vi "Beampointing_Multi_TRA2.vi"() -> ()   [LabVIEW 2020]
uses:
  Shared/GUI_Template/GUI_master/tcp new data cluster.ctl
  <userlib>/_OpenG.lib/array/array.llb/Filter 1D Array with Scalar (String)__ogtk.vi
  <vilib>/Utility/file.llb/Write To Spreadsheet File (string).vi
  <vilib>/Utility/file.llb/Read From Spreadsheet File (string).vi
  <vilib>/Analysis/NI_AALBase.lvlib
  GUI_Beampointing_single_TRA/Ctrs/move.ctl
  Ctrs/beam detection.ctl
  Shared/GUI_Template/GUI_master/tcp_new_data_event.ctl
panel:
  out "size(s) 6":i32
  out "x-y*floor(x/y)":dbl
  out "config path":string
  out "motor refs 7":refnum<vi>[](array[refnum])
  out "Moving Y":string
  out "Moving X":string
  out "particles":T1(array[cluster])
  out "motor refs 6":refnum<vi>[](array[refnum])
  out "millisecond timer value":u32
  out "motor refs 5":refnum<vi>[](array[refnum])
  out "appended path":path
  out "motor refs 4":refnum<vi>[](array[refnum])
  in  "active Axis ref 3":cluster{"Ref X":refnum<vi>, "Ref Y":refnum<vi>}
  out "motor refs 3":refnum<vi>[](array[refnum])
  in  "active man refs":cluster{"Ref X":refnum<vi>, "Ref Y":refnum<vi>}
  out "motor refs 2":refnum<vi>[](array[refnum])
  in  "Numeric":dbl
  out "Current State":string
  in  "output cluster 2":T5 {"detection para"."smal para"."Measurement Parameter" items=["Center of Mass X", "Center of Mass Y", "First Pixel X", "First Pixel Y", "Bounding Rect Left", "Bounding Rect Top", "Bounding Rect Right", "Bounding Rect Bottom", "Max Feret Diameter Start X", "Max Feret Diameter Start Y", "Max Feret Diameter End X", "Max Feret Diameter End Y", "Max Horiz. Segment Length Left", "Max Horiz. Segment Length Right", "Max Horiz. Segment Length Row", "-", "Bounding Rect Width", "Bounding Rect Height", "Bounding Rect Diagonal", "Perimeter", "Convex Hull Perimeter", "Holes' Perimeter", "Max Feret Diameter", "Equivalent Ellipse Major Axis", "Equivalent Ellipse Minor Axis", "Equivalent Ellipse Minor Axis (Feret)", "Equivalent Rect Long Side", "Equivalent Rect Short Side", "Equivalent Rect Diagonal", "Equivalent Rect Short Side (Feret)", "Average Horiz. Segment Length", "Average Vert. Segment Length", "Hydraulic Radius", "Waddel Disk Diameter", "-", "Area", "Holes' Area", "Particle & Holes' Area", "Convex Hull Area", "Image Area", "-", "Number of Holes", "Number of Horiz. Segments", "Number of Vert. Segments", "-", "Orientation", "Max Feret Diameter Orientation", "-", "% Area/Image Area", "% Area/(Particle & Holes' Area)", "Ratio of Equivalent Ellipse Axes", "Ratio of Equivalent Rect Sides", "-", "Elongation Factor", "Compactness Factor", "Heywood Circularity Factor", "Type Factor", "-", "Sum X", "Sum Y", "Sum XX", "Sum XY", "Sum YY", "Sum XXX", "Sum XXY", "Sum XYY", "Sum YYY", "-", "Moment of Inertia XX", "Moment of Inertia XY", "Moment of Inertia YY", "Moment of Inertia XXX", "Moment of Inertia XXY", "Moment of Inertia XYY", "Moment of Inertia YYY", "Norm. Moment of Inertia XX", "Norm. Moment of Inertia XY", "Norm. Moment of Inertia YY", "Norm. Moment of Inertia XXX", "Norm. Moment of Inertia XXY", "Norm. Moment of Inertia XYY", "Norm. Moment of Inertia YYY", "Hu Moment 1", "Hu Moment 2", "Hu Moment 3", "Hu Moment 4", "Hu Moment 5", "Hu Moment 6", "Hu Moment 7"]; "detection para"."smal para"."Range Lower Value" format="%.2f"; "detection para"."smal para"."Range Upper Value" format="%.2f"; "detection para"."detection method" items=["clustering", "entropy", "metric", "moments", "inter-class variance"]; "detection para"."Filter" items=["No Filter", "Median Filter", "Low Pass Filter"]}
  out "CCDs":string[](array[string])
  in  "GUIdevice 12":string
  in  "GUIdevice 11":string
  in  "GUIdevice 10":string
  in  "GUIdevice 9":string
  out "error out 2":errorcluster
  in  "active cams":string[](array[string])
  in  "Motor Y":dbl[][](array[numeric])
  in  "Motor X":dbl[][](array[numeric])
  out "Names":string[](array[string])
  in  "Offset X stats":dbl[][](array[numeric])
  in  "Offset Y stats":dbl[][](array[numeric])
  out "Box":T6(array[cluster])
  in  "Tab Control 2":enum32{"Config ", "Main", "History"}(tab)=enum."Main"
  in  "associated motors":T7 {"Motor CCD 12" items=["M20", "SIM", "M22", ""]; "Motor CCD 11" items=["M20", "SIM", "M22", ""]; "Motor CCD 10" items=["M20", "SIM", "M22", ""]; "Motor CCD 9" items=["M20", "SIM", "M22", ""]; "Motor CCD 8" items=["M20", "SIM", "M22", ""]; "Motor CCD 7" items=["M20", "SIM", "M22", ""]; "Motor CCD 6" items=["M20", "SIM", "M22", ""]; "Motor CCD 5" items=["M20", "SIM", "M22", ""]; "Motor CCD 4" items=["M20", "SIM", "M22", ""]; "Motor CCD 3" items=["M20", "SIM", "M22", ""]; "Motor CCD 2" items=["M20", "SIM", "M22", ""]; "Motor CCD 1" items=["M20", "SIM", "M22", ""]}
  out "Cameras":T8
  out "Status":cluster{i32, i32, "Centroid X":dbl[][]}(graph)
  in  "Exposure:12":dbl=0.095 min=0.0001 max=1.0 format="%#_6f"
  in  "Triggerdelay::12":dbl=0.003 min=0.0 max=0.09 format="%#_6f"
  in  "Exposure::11":dbl=0.095 min=0.0001 max=1.0 format="%#_6f"
  in  "Triggerdelay::11":dbl=0.003 min=0.0 max=0.09 format="%#_6f"
  in  "Exposure::10":dbl=0.095 min=0.0001 max=1.0 format="%#_6f"
  in  "Triggerdelay::10":dbl=0.003 min=0.0 max=0.09 format="%#_6f"
  in  "Exposure::9":dbl=0.095 min=0.0001 max=1.0 format="%#_6f"
  in  "Triggerdelay::9":dbl=0.003 min=0.0 max=0.09 format="%#_6f"
  in  "Trigger::9":bool
  in  "Trigger::10":bool caption="Trigger:10"
  in  "Trigger::11":bool
  in  "Trigger::12":bool
  in  "Target.Y::9":dbl=45.0 caption="T9y" min=0.0 max=2000.0 format="%#_6f"
  in  "Target.X::9":dbl=47.0 caption="Tx9" min=0.0 max=2000.0 format="%#_6f"
  in  "Target.Y::10":dbl=45.0 caption="T10y" min=0.0 max=2000.0 format="%#_6f"
  in  "Target.X::10":dbl=47.0 caption="T10x" min=0.0 max=2000.0 format="%#_6f"
  in  "Target.Y::11":dbl=45.0 caption="T11y" min=0.0 max=2000.0 format="%#_6f"
  in  "Target.X::11":dbl=47.0 caption="T11x" min=0.0 max=2000.0 format="%#_6f"
  in  "Target.Y::12":dbl=45.0 caption="T12y" min=0.0 max=2000.0 format="%#_6f"
  in  "Target.X::12":dbl=47.0 caption="T12x" min=0.0 max=2000.0 format="%#_6f"
  in  "Exposure::8":dbl=0.095 min=0.0001 max=1.0 format="%#_6f"
  in  "Triggerdelay::8":dbl=0.003 min=0.0 max=0.09 format="%#_6f"
  in  "Trigger::8":bool
  in  "Target.Y::8":dbl=45.0 caption="T8y" min=0.0 max=2000.0 format="%#_6f"
  in  "Target.X::8":dbl=47.0 caption="T8x" min=0.0 max=2000.0 format="%#_6f"
  in  "Target.Y::7":dbl=45.0 caption="T7x" min=0.0 max=2000.0 format="%#_6f"
  in  "Target.X::7":dbl=47.0 caption="T7y" min=0.0 max=2000.0 format="%#_6f"
  in  "Target.Y::6":dbl=45.0 caption="T6y" min=0.0 max=2000.0 format="%#_6f"
  in  "Target.X::6":dbl=47.0 caption="T6x" min=0.0 max=2000.0 format="%#_6f"
  in  "Target.Y::5":dbl=45.0 caption="T5y" min=0.0 max=2000.0 format="%#_6f"
  in  "Target.X::5":dbl=47.0 caption="T5x" min=0.0 max=2000.0 format="%#_6f"
  in  "Target.Y::4":dbl=45.0 caption="T4y" min=0.0 max=2000.0 format="%#_6f"
  in  "Target.X::4":dbl=47.0 caption="T4x" min=0.0 max=2000.0 format="%#_6f"
  in  "Target.Y::3":dbl=163.0 caption="T3y" min=0.0 max=2000.0 format="%#_6f"
  in  "Target.X::3":dbl=152.0 caption="T3x" min=0.0 max=2000.0 format="%#_6f"
  in  "Target.Y::2":dbl=74.0 caption="T2y" min=0.0 max=2000.0 format="%#_6f"
  in  "Target.X::2":dbl=75.0 caption="T2x" min=0.0 max=2000.0 format="%#_6f"
  in  "Target.Y::1":dbl=61.0 caption="T1y" min=0.0 max=2000.0 format="%#_6f"
  in  "Target.X::1":dbl=77.0 caption="T1x" min=0.0 max=2000.0 format="%#_6f"
  in  "Exposure::7":dbl=0.095 min=0.0001 max=1.0 format="%#_6f"
  in  "Triggerdelay::7":dbl=0.003 min=0.0 max=0.09 format="%#_6f"
  in  "Trigger::7":bool
  in  "Exposure::6":dbl=0.095 min=0.0001 max=1.0 format="%#_6f"
  in  "Triggerdelay::6":dbl=0.003 min=0.0 max=0.09 format="%#_6f"
  in  "Trigger::6":bool
  in  "Exposure::5":dbl=0.095 min=0.0001 max=1.0 format="%#_6f"
  in  "Triggerdelay::5":dbl=0.003 min=0.0 max=0.09 format="%#_6f"
  in  "Trigger::5":bool
  in  "Exposure::4":dbl=0.095 min=0.0001 max=1.0 format="%#_6f"
  in  "Triggerdelay::4":dbl=0.003 min=0.0 max=0.09 format="%#_6f"
  in  "Trigger::4":bool
  in  "Exposure::3":dbl=0.095 min=0.0001 max=1.0 format="%#_6f"
  in  "Triggerdelay::3":dbl=0.003 min=0.0 max=0.09 format="%#_6f"
  in  "Trigger::3":bool
  in  "Exposure::2":dbl=0.095 min=0.0001 max=1.0 format="%#_6f"
  in  "Triggerdelay::2":dbl=0.003 min=0.0 max=0.09 format="%#_6f"
  in  "Trigger::2":bool
  out "image::1":T9(plugin-control) caption="B3_TelLens2"
  out "image::2":T9(plugin-control) caption="B6_SwitchYNear"
  out "image::3":T9(plugin-control) caption="StagingM1Near"
  out "image::4":T9(plugin-control) caption="StagingM1Far"
  out "image::5":T9(plugin-control)
  out "image::6":T9(plugin-control)
  out "image::7":T9(plugin-control)
  out "image::8":T9(plugin-control)
  in  "Exposure::1":dbl=0.095 min=0.0001 max=1.0 format="%#_6f"
  in  "Triggerdelay::1":dbl=0.003 min=0.0 max=0.09 format="%#_6f"
  in  "Trigger::1":bool
  in  "UDP error message":string
  out "required Y":bool[](array[boolean])
  out "required X":bool[](array[boolean])
  out "detected":bool[](array[boolean])
  out "name array":string[](array[string])
  out "image::9":T9(plugin-control)
  out "image::10":T9(plugin-control)
  out "image::11":T9(plugin-control)
  out "image::12":T9(plugin-control)
  out "speedmode X":bool[](array[boolean])
  out "speedmode Y":bool[](array[boolean])
  out "CCD 9":cluster{timestamp[], dbl[]}[](graph)
  out "CCD 10":cluster{timestamp[], dbl[]}[](graph)
  out "CCD 11":cluster{timestamp[], dbl[]}[](graph)
  out "CCD 12":cluster{timestamp[], dbl[]}[](graph)
  out "CCD 5":cluster{timestamp[], dbl[]}[](graph)
  out "CCD 6":cluster{timestamp[], dbl[]}[](graph)
  out "CCD 7":cluster{timestamp[], dbl[]}[](graph)
  out "CCD 8":cluster{timestamp[], dbl[]}[](graph)
  out "CCD 2":cluster{timestamp[], dbl[]}[](graph)
  out "CCD 1":cluster{timestamp[], dbl[]}[](graph)
  out "CCD 3":cluster{timestamp[], dbl[]}[](graph)
  out "CCD 4":cluster{timestamp[], dbl[]}[](graph)
  in  "History Size":i32=500
  out "History Index":i32
  in  "Feedback Global":bool
  in  "detection para":T3[](array[typedef])=[{"Filter"=1, "Filter Para"={"X Size"=5, "Y Size"=5, "% Tolerance"=1}, "detection method"=4, "smal para"=[{"Measurement Parameter"=35, "Range Lower Value"=0.0, "Range Upper Value"=0.0, "Range"=TRUE, "Measurement Type"=FALSE}], "Remove small Objects"=TRUE, "Restrict to round Objects"=FALSE}, {"Filter"=1, "Filter Para"={"X Size"=5, "Y Size"=5, "% Tolerance"=1}, "detection method"=4, "smal para"=[{"Measurement Parameter"=35, "Range Lower Value"=0.0, "Range Upper Value"=500.0, "Range"=FALSE, "Measurement Type"=FALSE}], "Remove small Objects"=TRUE, "Restrict to round Objects"=FALSE}, {"Filter"=1, "Filter Para"={"X Size"=5, "Y Size"=5, "% Tolerance"=1}, "detection method"=4, "smal para"=[{"Measurement Parameter"=35, "Range Lower Value"=0.0, "Range Upper Value"=500.0, "Range"=TRUE, "Measurement Type"=FALSE}], "Remove small Objects"=TRUE, "Restrict to round Objects"=FALSE}, {"Filter"=1, "Filter Para"={"X Size"=5, "Y Size"=5, "% Tolerance"=1}, "detection method"=4, "smal para"=[{"Measurement Parameter"=35, "Range Lower Value"=0.0, "Range Upper Value"=500.0, "Range"=TRUE, "Measurement Type"=FALSE}], "Remove small Objects"=TRUE, "Restrict to round Objects"=FALSE}, {"Filter"=1, "Filter Para"={"X Size"=5, "Y Size"=5, "% Tolerance"=1}, "detection method"=4, "smal para"=[{"Measurement Parameter"=35, "Range Lower Value"=0.0, "Range Upper Value"=500.0, "Range"=TRUE, "Measurement Type"=FALSE}], "Remove small Objects"=TRUE, "Restrict to round Objects"=FALSE}, {"Filter"=1, "Filter Para"={"X Size"=5, "Y Size"=5, "% Tolerance"=1}, "detection method"=4, "smal para"=[{"Measurement Parameter"=35, "Range Lower Value"=0.0, "Range Upper Value"=500.0, "Range"=TRUE, "Measurement Type"=FALSE}], "Remove small Objects"=TRUE, "Restrict to round Objects"=FALSE}, {"Filter"=1, "Filter Para"={"X Size"=5, "Y Size"=5, "% Tolerance"=1}, "detection method"=4, "smal para"=[{"Measurement Parameter"=35, "Range Lower Value"=0.0, "Range Upper Value"=500.0, "Range"=TRUE, "Measurement Type"=FALSE}], "Remove small Objects"=TRUE, "Restrict to round Objects"=FALSE}, {"Filter"=1, "Filter Para"={"X Size"=5, "Y Size"=5, "% Tolerance"=1}, "detection method"=3, "smal para"=[{"Measurement Parameter"=35, "Range Lower Value"=0.0, "Range Upper Value"=0.0, "Range"=FALSE, "Measurement Type"=FALSE}], "Remove small Objects"=TRUE, "Restrict to round Objects"=FALSE}, {"Filter"=1, "Filter Para"={"X Size"=5, "Y Size"=5, "% Tolerance"=1}, "detection method"=4, "smal para"=[{"Measurement Parameter"=35, "Range Lower Value"=0.0, "Range Upper Value"=0.0, "Range"=FALSE, "Measurement Type"=FALSE}], "Remove small Objects"=TRUE, "Restrict to round Objects"=FALSE}, {"Filter"=1, "Filter Para"={"X Size"=5, "Y Size"=5, "% Tolerance"=1}, "detection method"=4, "smal para"=[{"Measurement Parameter"=35, "Range Lower Value"=0.0, "Range Upper Value"=500.0, "Range"=TRUE, "Measurement Type"=FALSE}], "Remove small Objects"=TRUE, "Restrict to round Objects"=FALSE}, {"Filter"=1, "Filter Para"={"X Size"=5, "Y Size"=5, "% Tolerance"=1}, "detection method"=4, "smal para"=[{"Measurement Parameter"=35, "Range Lower Value"=0.0, "Range Upper Value"=500.0, "Range"=TRUE, "Measurement Type"=FALSE}], "Remove small Objects"=TRUE, "Restrict to round Objects"=FALSE}, {"Filter"=1, "Filter Para"={"X Size"=5, "Y Size"=5, "% Tolerance"=1}, "detection method"=4, "smal para"=[{"Measurement Parameter"=35, "Range Lower Value"=0.0, "Range Upper Value"=500.0, "Range"=TRUE, "Measurement Type"=FALSE}], "Remove small Objects"=TRUE, "Restrict to round Objects"=FALSE}] {"smal para"."Measurement Parameter" items=["Center of Mass X", "Center of Mass Y", "First Pixel X", "First Pixel Y", "Bounding Rect Left", "Bounding Rect Top", "Bounding Rect Right", "Bounding Rect Bottom", "Max Feret Diameter Start X", "Max Feret Diameter Start Y", "Max Feret Diameter End X", "Max Feret Diameter End Y", "Max Horiz. Segment Length Left", "Max Horiz. Segment Length Right", "Max Horiz. Segment Length Row", "-", "Bounding Rect Width", "Bounding Rect Height", "Bounding Rect Diagonal", "Perimeter", "Convex Hull Perimeter", "Holes' Perimeter", "Max Feret Diameter", "Equivalent Ellipse Major Axis", "Equivalent Ellipse Minor Axis", "Equivalent Ellipse Minor Axis (Feret)", "Equivalent Rect Long Side", "Equivalent Rect Short Side", "Equivalent Rect Diagonal", "Equivalent Rect Short Side (Feret)", "Average Horiz. Segment Length", "Average Vert. Segment Length", "Hydraulic Radius", "Waddel Disk Diameter", "-", "Area", "Holes' Area", "Particle & Holes' Area", "Convex Hull Area", "Image Area", "-", "Number of Holes", "Number of Horiz. Segments", "Number of Vert. Segments", "-", "Orientation", "Max Feret Diameter Orientation", "-", "% Area/Image Area", "% Area/(Particle & Holes' Area)", "Ratio of Equivalent Ellipse Axes", "Ratio of Equivalent Rect Sides", "-", "Elongation Factor", "Compactness Factor", "Heywood Circularity Factor", "Type Factor", "-", "Sum X", "Sum Y", "Sum XX", "Sum XY", "Sum YY", "Sum XXX", "Sum XXY", "Sum XYY", "Sum YYY", "-", "Moment of Inertia XX", "Moment of Inertia XY", "Moment of Inertia YY", "Moment of Inertia XXX", "Moment of Inertia XXY", "Moment of Inertia XYY", "Moment of Inertia YYY", "Norm. Moment of Inertia XX", "Norm. Moment of Inertia XY", "Norm. Moment of Inertia YY", "Norm. Moment of Inertia XXX", "Norm. Moment of Inertia XXY", "Norm. Moment of Inertia XYY", "Norm. Moment of Inertia YYY", "Hu Moment 1", "Hu Moment 2", "Hu Moment 3", "Hu Moment 4", "Hu Moment 5", "Hu Moment 6", "Hu Moment 7"]; "smal para"."Range Lower Value" format="%.2f"; "smal para"."Range Upper Value" format="%.2f"; "detection method" items=["clustering", "entropy", "metric", "moments", "inter-class variance"]; "Filter" items=["No Filter", "Median Filter", "Low Pass Filter"]}
  in  "GUIdevice 8":string
  in  "Tab Control":T10(tab)=enum."Detection"
  in  "new tdms":bool
  in  "Save Stats":bool
  in  "Save Config":bool
  in  "Load Config":bool
  in  "update speed [ms]":i32=200
  in  "img to avg":i32=6 min=3 max=200
  in  "Reset History":bool
  in  "save path":path=path "W:/BP_DATA"
  in  "autodetect":bool
  in  "Detection Rate":dbl=0.9 min=0.001 max=1.0
  in  "Center":bool
  in  "Align":bool
  in  "Speedmode @":dbl=3.0 min=1.0 max=20.0
  in  "device ini":bool
  in  "beam detection para":T3={"Filter"=1, "Filter Para"={"X Size"=5, "Y Size"=5, "% Tolerance"=1}, "detection method"=4, "smal para"=[{"Measurement Parameter"=35, "Range Lower Value"=0.0, "Range Upper Value"=500.0, "Range"=FALSE, "Measurement Type"=FALSE}], "Remove small Objects"=TRUE, "Restrict to round Objects"=FALSE} {"smal para"."Measurement Parameter" items=["Center of Mass X", "Center of Mass Y", "First Pixel X", "First Pixel Y", "Bounding Rect Left", "Bounding Rect Top", "Bounding Rect Right", "Bounding Rect Bottom", "Max Feret Diameter Start X", "Max Feret Diameter Start Y", "Max Feret Diameter End X", "Max Feret Diameter End Y", "Max Horiz. Segment Length Left", "Max Horiz. Segment Length Right", "Max Horiz. Segment Length Row", "-", "Bounding Rect Width", "Bounding Rect Height", "Bounding Rect Diagonal", "Perimeter", "Convex Hull Perimeter", "Holes' Perimeter", "Max Feret Diameter", "Equivalent Ellipse Major Axis", "Equivalent Ellipse Minor Axis", "Equivalent Ellipse Minor Axis (Feret)", "Equivalent Rect Long Side", "Equivalent Rect Short Side", "Equivalent Rect Diagonal", "Equivalent Rect Short Side (Feret)", "Average Horiz. Segment Length", "Average Vert. Segment Length", "Hydraulic Radius", "Waddel Disk Diameter", "-", "Area", "Holes' Area", "Particle & Holes' Area", "Convex Hull Area", "Image Area", "-", "Number of Holes", "Number of Horiz. Segments", "Number of Vert. Segments", "-", "Orientation", "Max Feret Diameter Orientation", "-", "% Area/Image Area", "% Area/(Particle & Holes' Area)", "Ratio of Equivalent Ellipse Axes", "Ratio of Equivalent Rect Sides", "-", "Elongation Factor", "Compactness Factor", "Heywood Circularity Factor", "Type Factor", "-", "Sum X", "Sum Y", "Sum XX", "Sum XY", "Sum YY", "Sum XXX", "Sum XXY", "Sum XYY", "Sum YYY", "-", "Moment of Inertia XX", "Moment of Inertia XY", "Moment of Inertia YY", "Moment of Inertia XXX", "Moment of Inertia XXY", "Moment of Inertia XYY", "Moment of Inertia YYY", "Norm. Moment of Inertia XX", "Norm. Moment of Inertia XY", "Norm. Moment of Inertia YY", "Norm. Moment of Inertia XXX", "Norm. Moment of Inertia XXY", "Norm. Moment of Inertia XYY", "Norm. Moment of Inertia YYY", "Hu Moment 1", "Hu Moment 2", "Hu Moment 3", "Hu Moment 4", "Hu Moment 5", "Hu Moment 6", "Hu Moment 7"]; "smal para"."Range Lower Value" format="%.2f"; "smal para"."Range Upper Value" format="%.2f"; "detection method" items=["clustering", "entropy", "metric", "moments", "inter-class variance"]; "Filter" items=["No Filter", "Median Filter", "Low Pass Filter"]}
  in  "move config":T11={"Tolerance [%]"=0.1, "Stepsize"=0.0001, "Invert Axis"=TRUE, "Invert Direction X"=FALSE, "Invert Direction Y"=TRUE, "enable feedback"=FALSE, "Set Centriod Target"=FALSE}
  in  "Position 2":dbl=0.001 caption="Stepsize" min=0.0 max=999999.0 format="%_6f"
  in  "Position 1":dbl=0.001 caption="Stepsize" min=0.0 max=999999.0 format="%_6f"
  in  "Right":bool caption="RelativeMove.Axis 1.CCW::1"
  in  "Left":bool caption="RelativeMove.Axis 1.CW::1"
  in  "Down":bool caption="RelativeMove.Axis. 2.CCW::1"
  in  "Up":bool caption="RelativeMove.Axis 2.CW::1"
  in  "StepSize":dbl=0.001 caption="Stepsize" min=0.0 max=999999.0 format="%_1p"
  in  "active axis refs 2":T12(array[cluster])
  in  "active Axis ref":cluster{"Ref X":refnum<vi>, "Ref Y":refnum<vi>}
  in  "CCDs":u16(ring) items=["B3_TelLens2", "B6_SwitchYNear", "StagingM1Near", "StagingM1Far", "", "", "", "", "", "", "", ""]
  out "motor refs":refnum<vi>[](array[refnum])
  in  "Position.Axis 4::99":dbl=77.0 caption="Motor Axis 1" min=0.0 max=6.0 format="%#_6f"
  in  "Position.Axis 5::99":dbl=77.0 caption="Motor Axis 1" min=0.0 max=6.0 format="%#_6f"
  in  "Position.Axis 6::99":dbl=77.0 caption="Motor Axis 1" min=0.0 max=6.0 format="%#_6f"
  in  "Position.Axis 3::99":dbl=77.0 caption="Motor Axis 1" min=0.0 max=6.0 format="%#_6f"
  in  "Position.Axis 2::99":dbl=77.0 caption="Motor Axis 1" min=0.0 max=6.0 format="%#_6f"
  in  "Position.Axis 1::99":dbl=77.0 caption="Motor Axis 1" min=0.0 max=6.0 format="%#_6f"
  in  "GUIdevice 99":string="TREX TRA1"
  in  "move properties":T2[](array[typedef])=[{"Tolerance [%]"=0.1, "Stepsize"=0.0001, "Invert Direction X"=FALSE, "Invert Direction Y"=TRUE, "enable feedback"=FALSE, "Set Centriod Target"=FALSE}, {"Tolerance [%]"=0.1, "Stepsize"=0.0001, "Invert Direction X"=FALSE, "Invert Direction Y"=TRUE, "enable feedback"=FALSE, "Set Centriod Target"=FALSE}, {"Tolerance [%]"=0.1, "Stepsize"=0.0001, "Invert Direction X"=FALSE, "Invert Direction Y"=TRUE, "enable feedback"=FALSE, "Set Centriod Target"=FALSE}, {"Tolerance [%]"=0.1, "Stepsize"=0.0001, "Invert Direction X"=FALSE, "Invert Direction Y"=TRUE, "enable feedback"=FALSE, "Set Centriod Target"=FALSE}, {"Tolerance [%]"=0.1, "Stepsize"=0.0001, "Invert Direction X"=FALSE, "Invert Direction Y"=TRUE, "enable feedback"=FALSE, "Set Centriod Target"=FALSE}, {"Tolerance [%]"=0.1, "Stepsize"=0.0001, "Invert Direction X"=FALSE, "Invert Direction Y"=TRUE, "enable feedback"=FALSE, "Set Centriod Target"=FALSE}, {"Tolerance [%]"=0.1, "Stepsize"=0.0001, "Invert Direction X"=FALSE, "Invert Direction Y"=TRUE, "enable feedback"=FALSE, "Set Centriod Target"=FALSE}, {"Tolerance [%]"=0.1, "Stepsize"=0.0001, "Invert Direction X"=FALSE, "Invert Direction Y"=TRUE, "enable feedback"=FALSE, "Set Centriod Target"=FALSE}, {"Tolerance [%]"=0.1, "Stepsize"=0.0001, "Invert Direction X"=FALSE, "Invert Direction Y"=TRUE, "enable feedback"=FALSE, "Set Centriod Target"=FALSE}, {"Tolerance [%]"=0.1, "Stepsize"=0.0001, "Invert Direction X"=FALSE, "Invert Direction Y"=TRUE, "enable feedback"=FALSE, "Set Centriod Target"=FALSE}, {"Tolerance [%]"=0.1, "Stepsize"=0.0001, "Invert Direction X"=FALSE, "Invert Direction Y"=TRUE, "enable feedback"=FALSE, "Set Centriod Target"=FALSE}, {"Tolerance [%]"=0.1, "Stepsize"=0.0001, "Invert Direction X"=FALSE, "Invert Direction Y"=TRUE, "enable feedback"=FALSE, "Set Centriod Target"=FALSE}, {"Tolerance [%]"=0.1, "Stepsize"=0.0001, "Invert Direction X"=FALSE, "Invert Direction Y"=TRUE, "enable feedback"=FALSE, "Set Centriod Target"=FALSE}]
  in  "Time":timestamp[][](array[timestamp])
  in  "Mean Size":dbl[][](array[numeric])
  in  "Size":dbl[][](array[numeric])
  in  "active CCDs":i32(listbox)
  in  "Offset Y":dbl[][](array[numeric])
  in  "Offset X":dbl[][](array[numeric])
  in  "Mean Centroid X":dbl[][](array[numeric])
  in  "Mean Centroid Y":dbl[][](array[numeric])
  in  "Centroid Y":dbl[][](array[numeric])
  in  "Centroid X":dbl[][](array[numeric])
  in  "GUIdevice 7":string
  in  "GUIdevice 6":string
  in  "GUIdevice 5":string
  in  "GUIdevice 4":string
  in  "GUIdevice 3":string="TargetCam10Hz_Diode"
  in  "GUIdevice 2":string="StagingM1Far"
  in  "insert tag":bool=TRUE
  in  "stop":bool
  in  "GUIdevice 1":string="StagingM1Near"
  out "tcp data event":T13
  out "error IO 2":errorcluster
  # "x [Tolerance]"
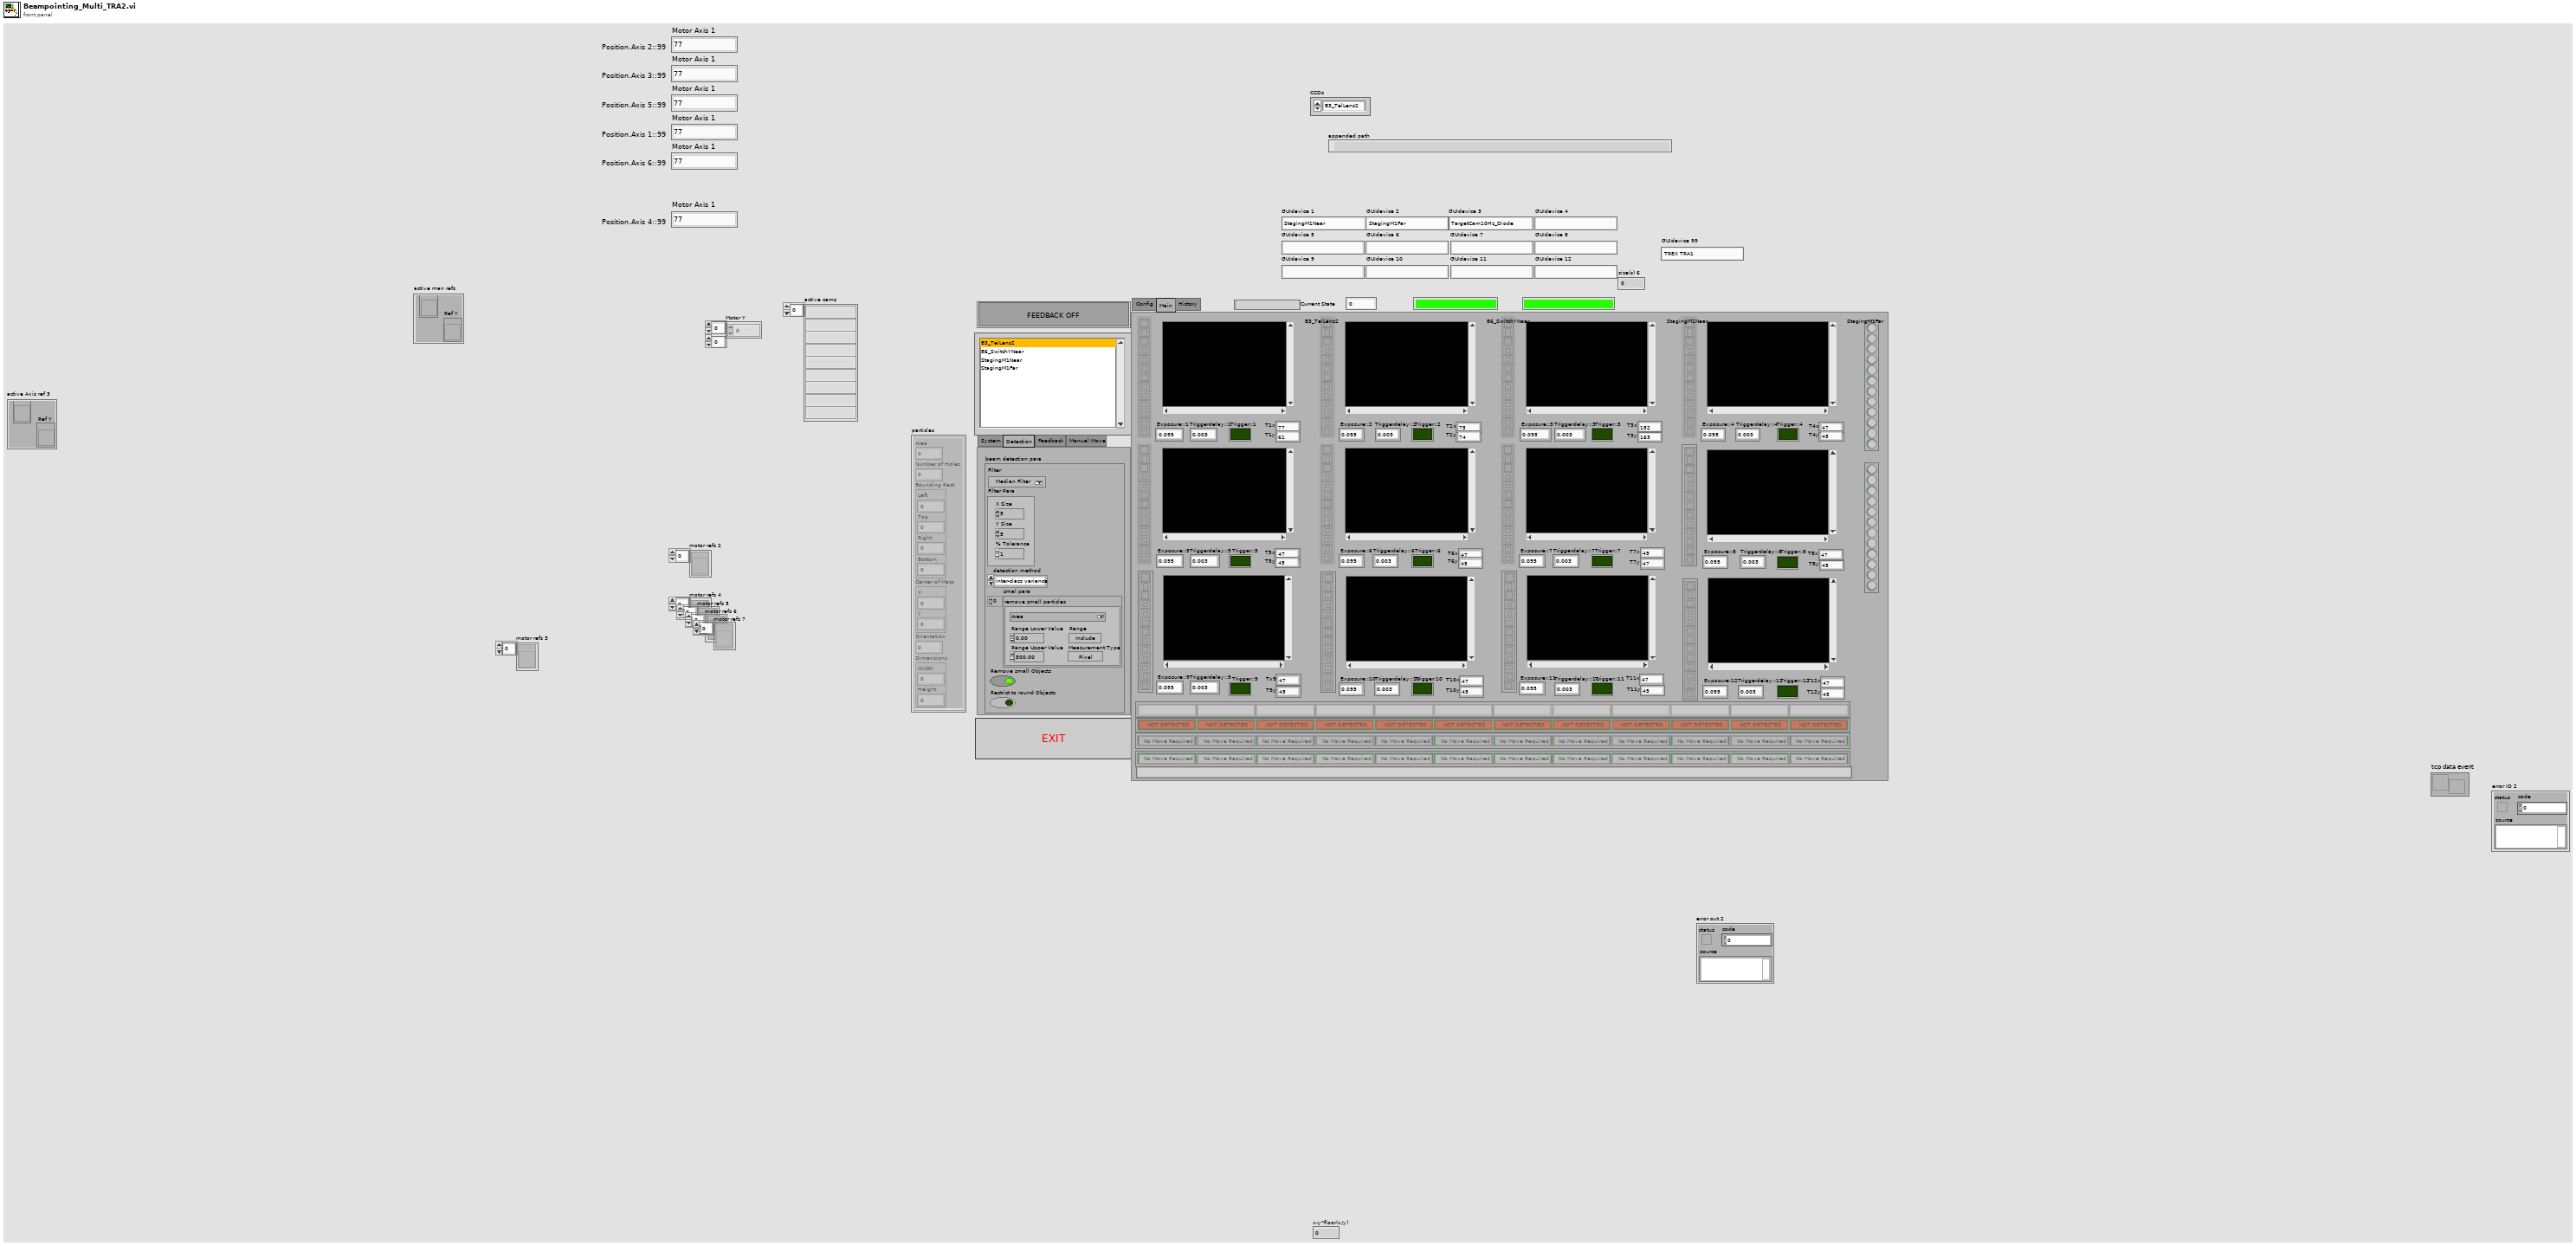
[diagram p1: front panel]
types:
  T1 = cluster{"Area":dbl, "Number of Holes":dbl, "Bounding Rect":cluster{"Left":dbl, "Top":dbl, "Right":dbl, "Bottom":dbl}, "Center of Mass":cluster{"X":dbl, "Y":dbl}, "Orientation":dbl, "Dimensions":cluster{"Width":dbl, "Height":dbl}}[]
  T2 = typedef "move.ctl" = cluster{"Tolerance [%]":dbl, "Stepsize":dbl, "Invert Direction X":bool, "Invert Direction Y":bool, "enable feedback":bool, "Set Centriod Target":bool}
  T3 = typedef "beam detection.ctl" = cluster{"Filter":u16, "Filter Para":cluster{"X Size":i32, "Y Size":i32, "% Tolerance":i32}, "detection method":i32, "smal para":cluster{"Measurement Parameter":T4, "Range Lower Value":dbl, "Range Upper Value":dbl, "Range":bool, "Measurement Type":bool}[], "Remove small Objects":bool, "Restrict to round Objects":bool}
  T4 = typedef "Particle Parameters" = i32
  T5 = cluster{"CCDs":string[], "move properties":T2[], "detection para":T3[], "thresholds":cluster{"Lower value":sgl, "Upper value":sgl}[], "Value":cluster{"Motor CCD 1":u16, "Motor CCD 2":u16, "Motor CCD 3":u16, "Motor CCD 4":u16, "Motor CCD 5":u16, "Motor CCD 6":u16, "Motor CCD 7":u16, "Motor CCD 8":u16, "Motor CCD 9":u16, "Motor CCD 10":u16, "Motor CCD 11":u16, "Motor CCD 12":u16}}
  T6 = cluster{"Left":dbl, "Top":dbl, "Right":dbl, "Bottom":dbl}[]
  T7 = cluster{"Motor CCD 1":u16, "Motor CCD 2":u16, "Motor CCD 3":u16, "Motor CCD 4":u16, "Motor CCD 5":u16, "Motor CCD 6":u16, "Motor CCD 7":u16, "Motor CCD 8":u16, "Motor CCD 9":u16, "Motor CCD 10":u16, "Motor CCD 11":u16, "Motor CCD 12":u16}
  T8 = cluster{"[0]":string, "[1]":string, "[2]":string, "[3]":string, "[4]":string, "[5]":string, "[6]":string, "[7]":string, "[8]":string, "[8] 2":string, "[8] 3":string, "[8] 4":string}
  T9 = typedef "IMAQ Image.ctl" = refnum<image>
  T10 = enum32{"System", "Detection", "Feedback", "Manual Move"}
  T11 = typedef "move.ctl" = cluster{"Tolerance [%]":dbl, "Stepsize":dbl, "Invert Axis":bool, "Invert Direction X":bool, "Invert Direction Y":bool, "enable feedback":bool, "Set Centriod Target":bool}
  T12 = cluster{"Ref X":refnum<vi>, "Ref Y":refnum<vi>}[]
  T13 = typedef "tcp_new_data_event.ctl" = refnum<user-event>
  T14 = typedef "tcp new data cluster.ctl" = cluster{"EventEnum":enum16{"new data", "connection status update"}, "Device name":string}
  T15 = cluster{"Left":i32, "Top":i32, "Right":i32, "Bottom":i32}
  T16 = enum32{"invalid app kind", "Development System", "Run Time System", "Student Edition", "Embedded LabVIEW", "Evaluation", "Custom"}
  T17 = enum16{"open", "open or create", "create or replace", "create", "open (read-only)"}
  T18 = enum32{"Invalid", "Standard", "Closed", "Hidden", "Minimized", "Maximized"}
  T19 = enum16{"open", "replace", "create", "open or create", "replace or create", "replace or create with confirmation"}
  T20 = enum8{"Enabled", "Disabled", "Disabled and Grayed Out"}
  T21 = typedef "Image Type" = u32
  T22 = cluster{"[0]":string, "[1]":string, "[2]":string, "[3]":string, "[4]":string, "[5]":string, "[6]":string, "[7]":string, "[8]":string, "[9]":string, "[10]":string, "[11]":string}
  T23 = cluster{"Target.X::1":refnum<vi>, "Target.Y::1":refnum<vi>}
  T24 = cluster{"Target.X::2":refnum<vi>, "Target.Y::2":refnum<vi>}
  T25 = cluster{"Target.X::3":refnum<vi>, "Target.Y::3":refnum<vi>}
  T26 = cluster{"Target.X::4":refnum<vi>, "Target.Y::4":refnum<vi>}
  T27 = cluster{"Target.X::5":refnum<vi>, "Target.Y::5":refnum<vi>}
  T28 = cluster{"Target.X::6":refnum<vi>, "Target.Y::6":refnum<vi>}
  T29 = cluster{"Target.X::7":refnum<vi>, "Target.Y::7":refnum<vi>}
  T30 = cluster{"Target.X::8":refnum<vi>, "Target.Y::8":refnum<vi>}
  T31 = cluster{"Target.X::12":refnum<vi>, "Target.Y::12":refnum<vi>}
  T32 = cluster{"Target.X::9":refnum<vi>, "Target.Y::9":refnum<vi>}
  T33 = cluster{"Target.X::10":refnum<vi>, "Target.Y::10":refnum<vi>}
  T34 = cluster{"Target.X::11":refnum<vi>, "Target.Y::11":refnum<vi>}
  T35 = cluster{"Target.X::12":refnum<vi>, "Target.Y::12":refnum<vi>}[]
  T36 = cluster{"Left":dbl, "Top":dbl, "Right":dbl, "Bottom":dbl}
  T37 = cluster{"Core":cluster{"Current VI Reference":refnum<vi>, "Close Panel on Exit?":bool}, "detection para":T3[], "thresholds":cluster{"Lower value":sgl, "Upper value":sgl}[], "Centroid X":dbl[][], "Centroid Y":dbl[][], "img to avg":i32, "Mean Centroid X":dbl[][], "Mean Centroid Y":dbl[][], "Offset X":dbl[][], "Offset Y":dbl[][], "Offset X stats ":dbl[][], "Offset Y stats ":dbl[][], "Size":dbl[][], "Mean Size":dbl[][], "Time":timestamp[][], "move properties":T2[], "active axis refs 2":cluster{"Ref X":refnum<vi>, "Ref Y":refnum<vi>}[], "active ccd":i32, "Feedback global":bool, "Motor X":dbl[][], "Motor Y":dbl[][], "active cams":string[], "Data Value Reference out":refnum<k34>, "active man refs":cluster{"Ref X":refnum<vi>, "Ref Y":refnum<vi>}, "detected":bool[], "speedmode X":bool[], "speedmode Y":bool[]}
  T38 = cluster{"Current VI Reference":refnum<vi>, "Close Panel on Exit?":bool}
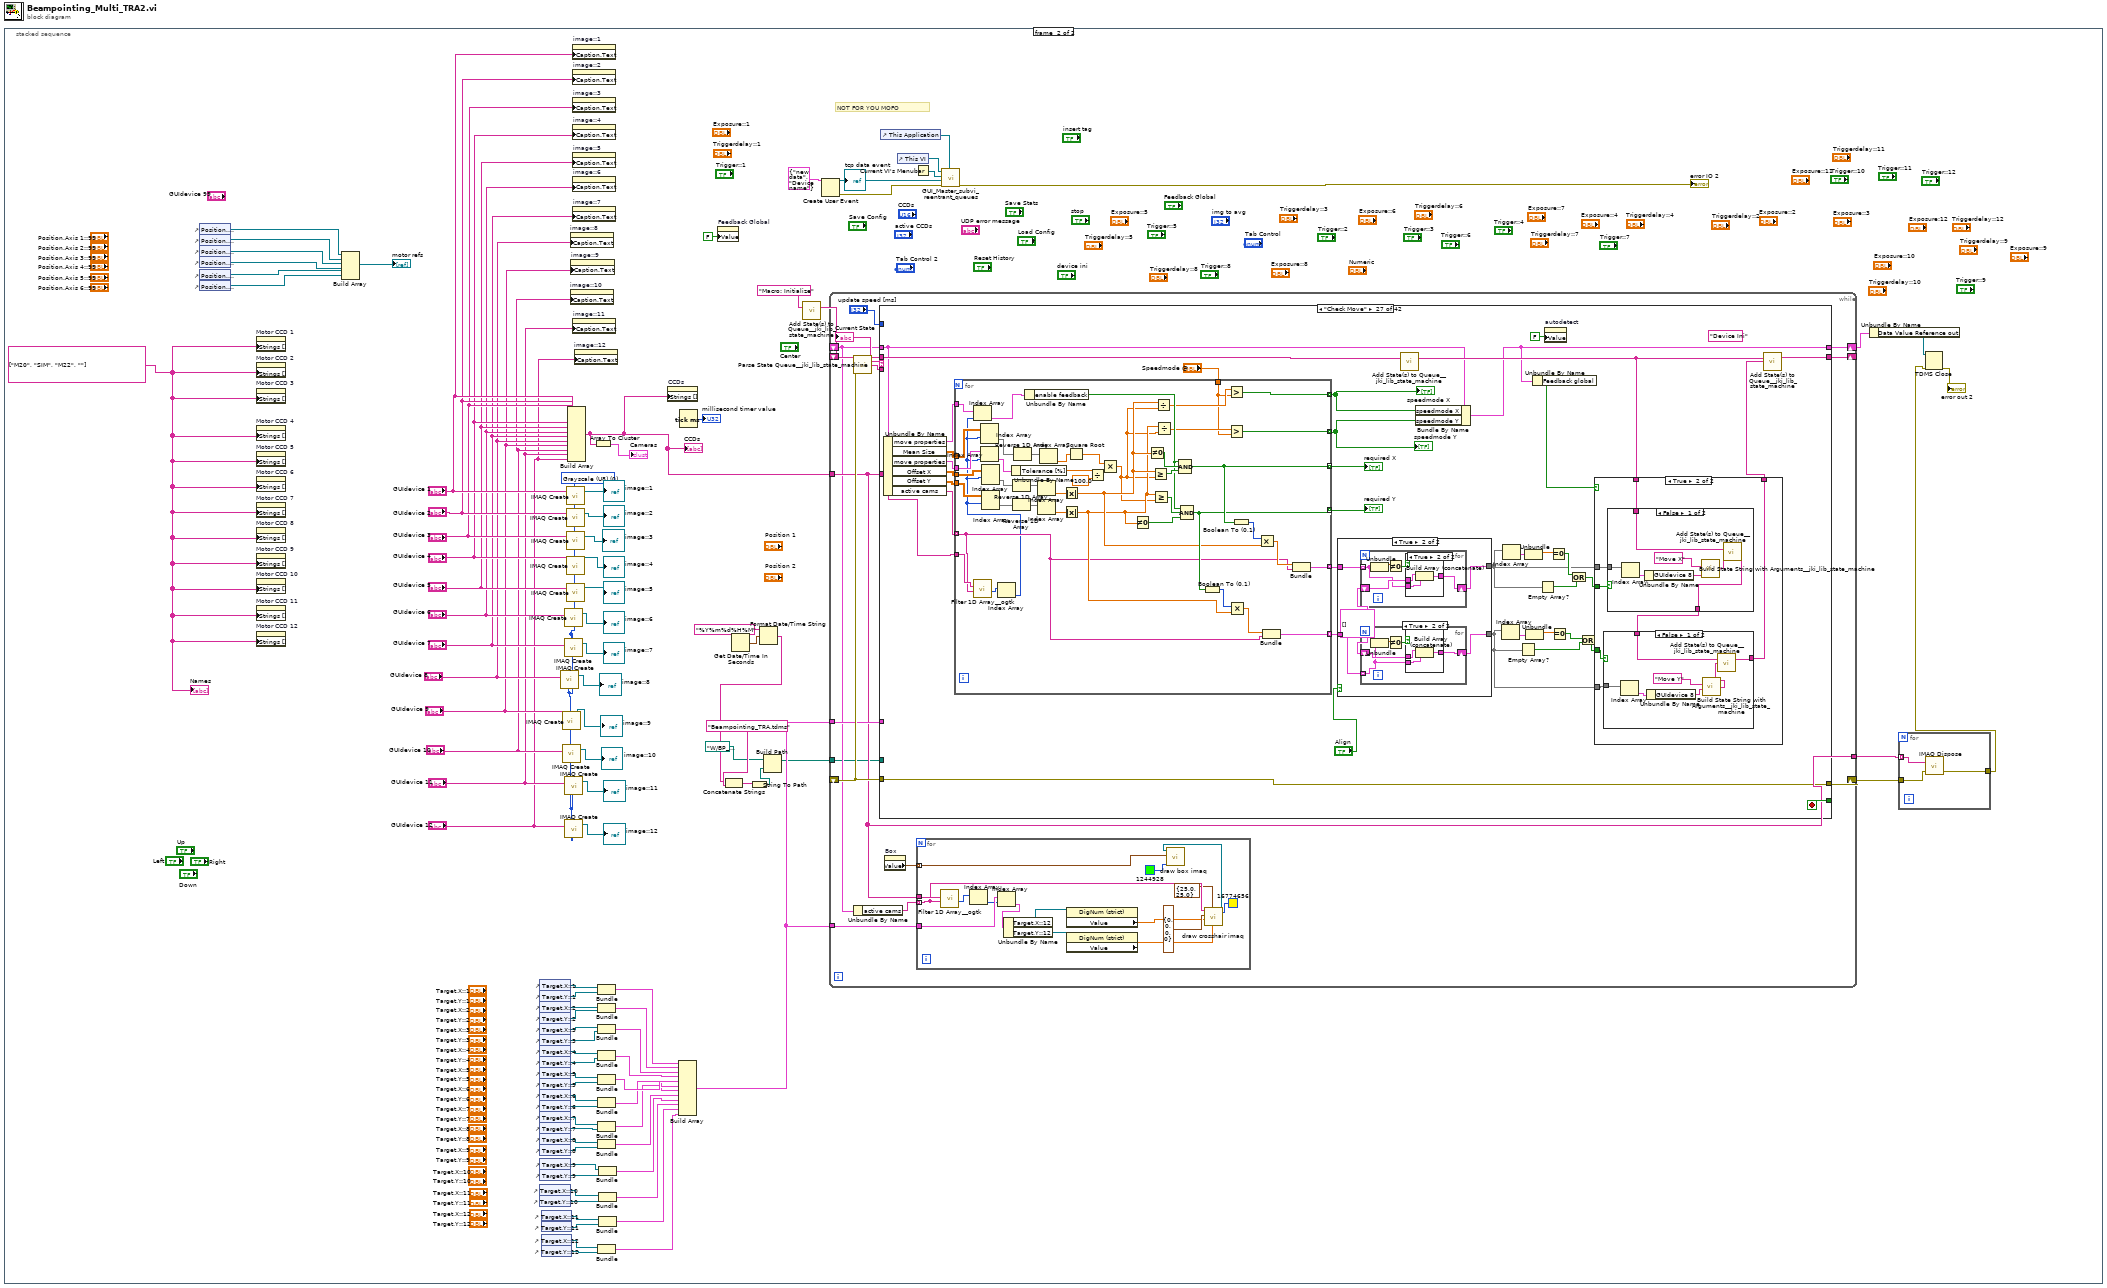
[diagram p0: block diagram]
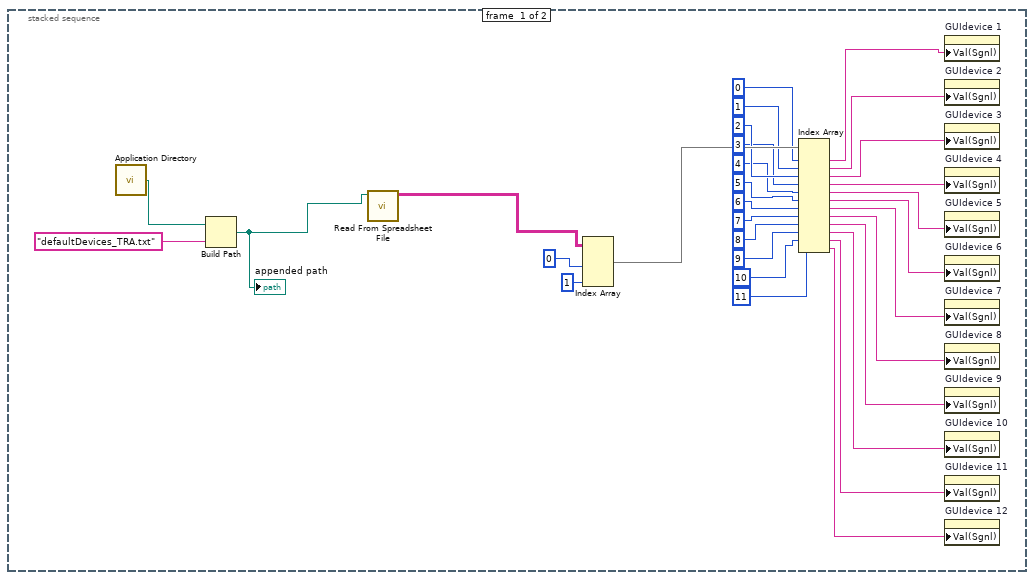
[diagram p2: hidden frame]
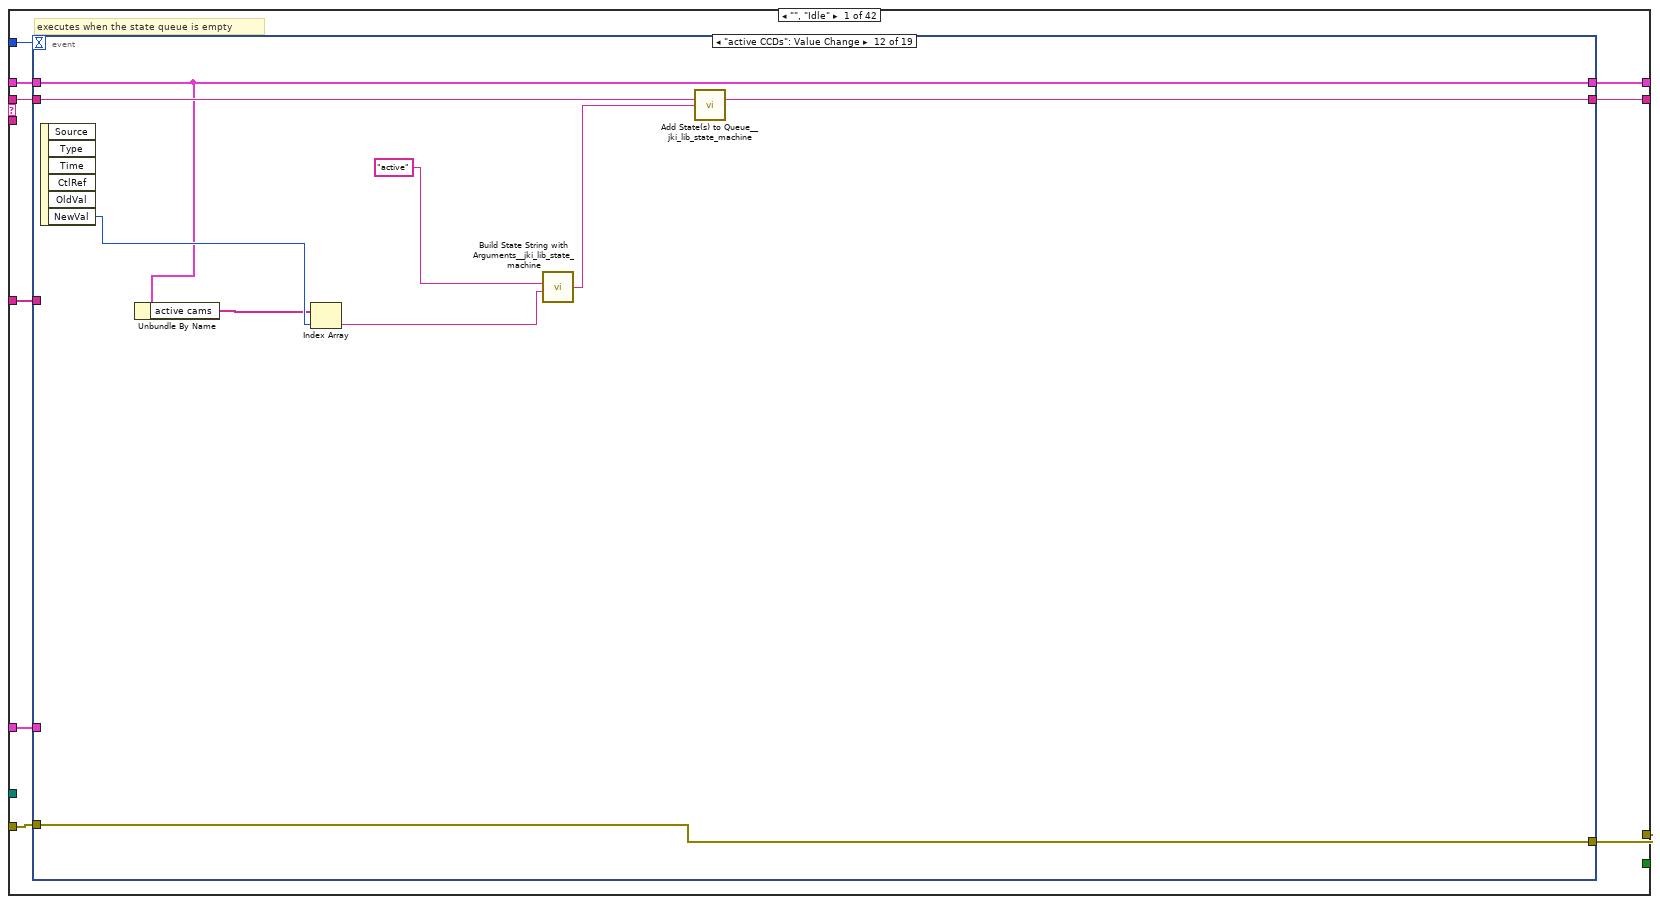
[diagram p3: hidden frame]
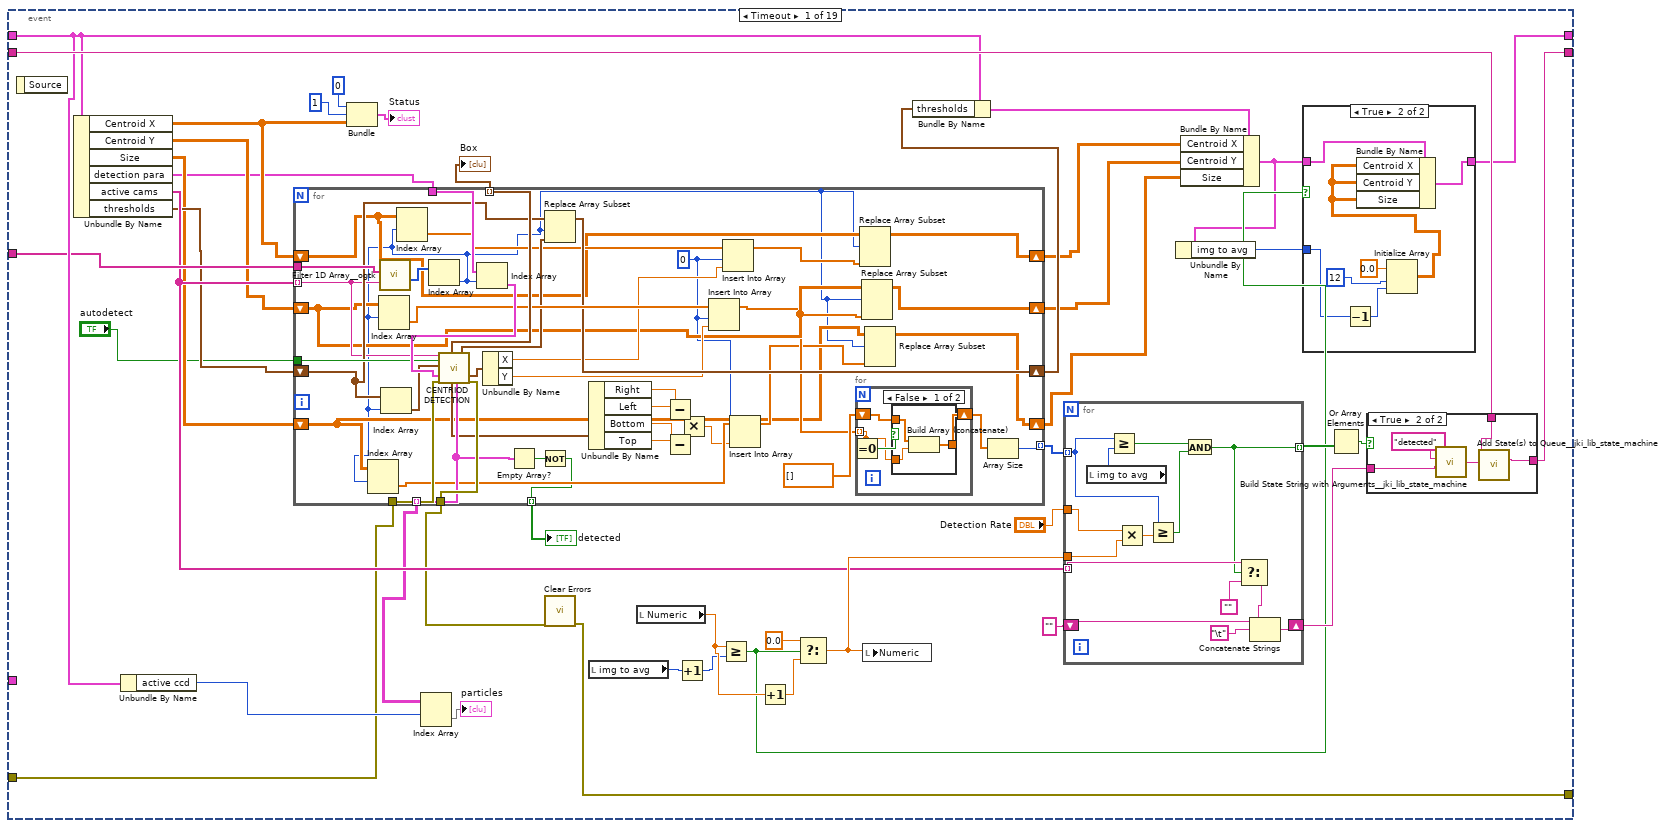
[diagram p4: hidden frame]
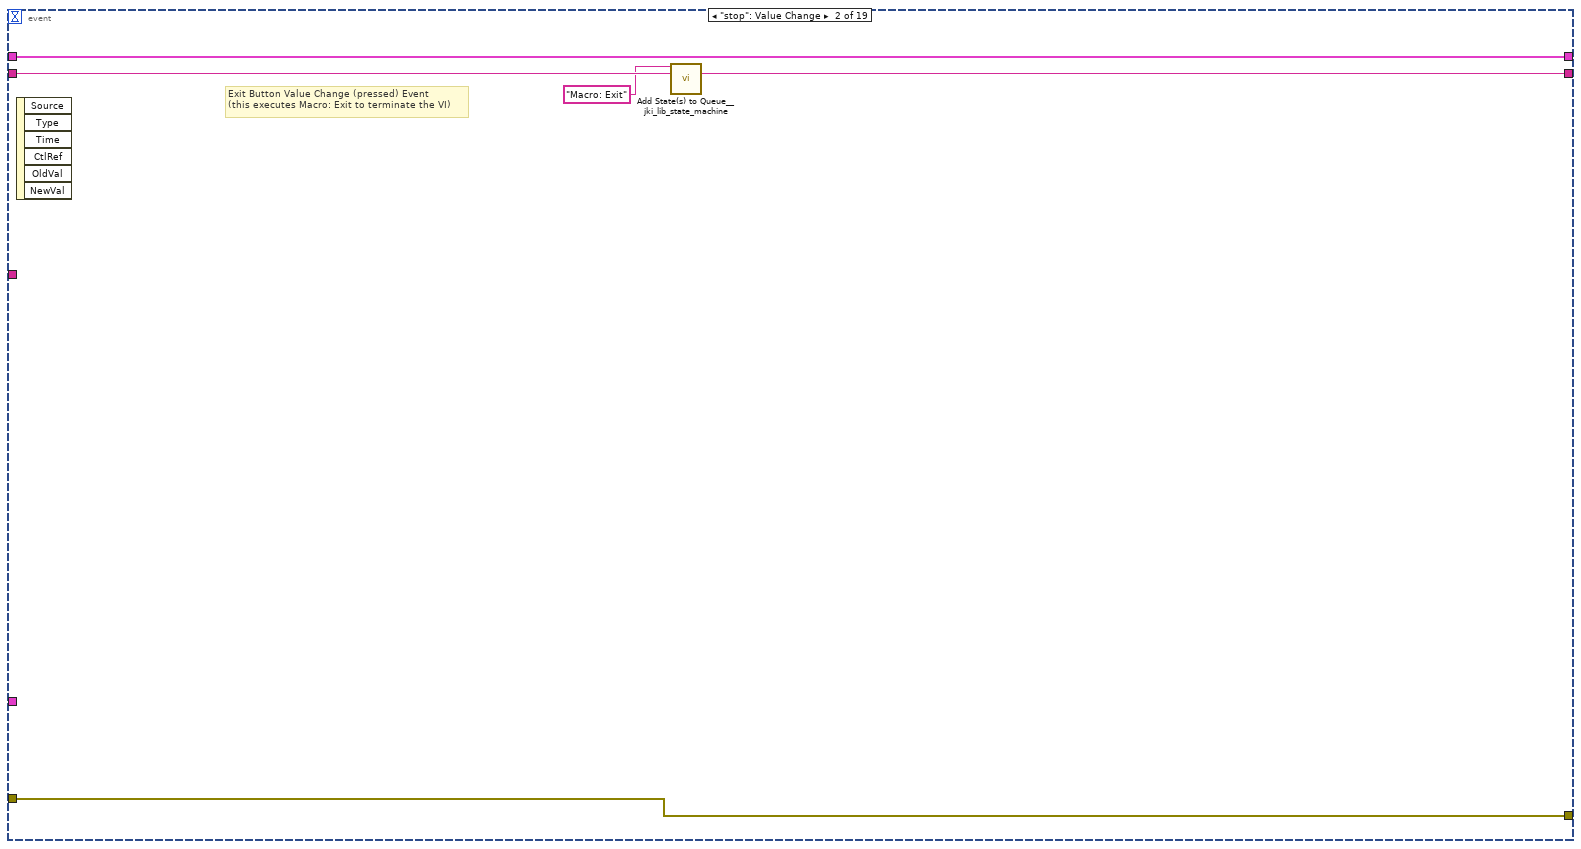
[diagram p8: hidden frame]
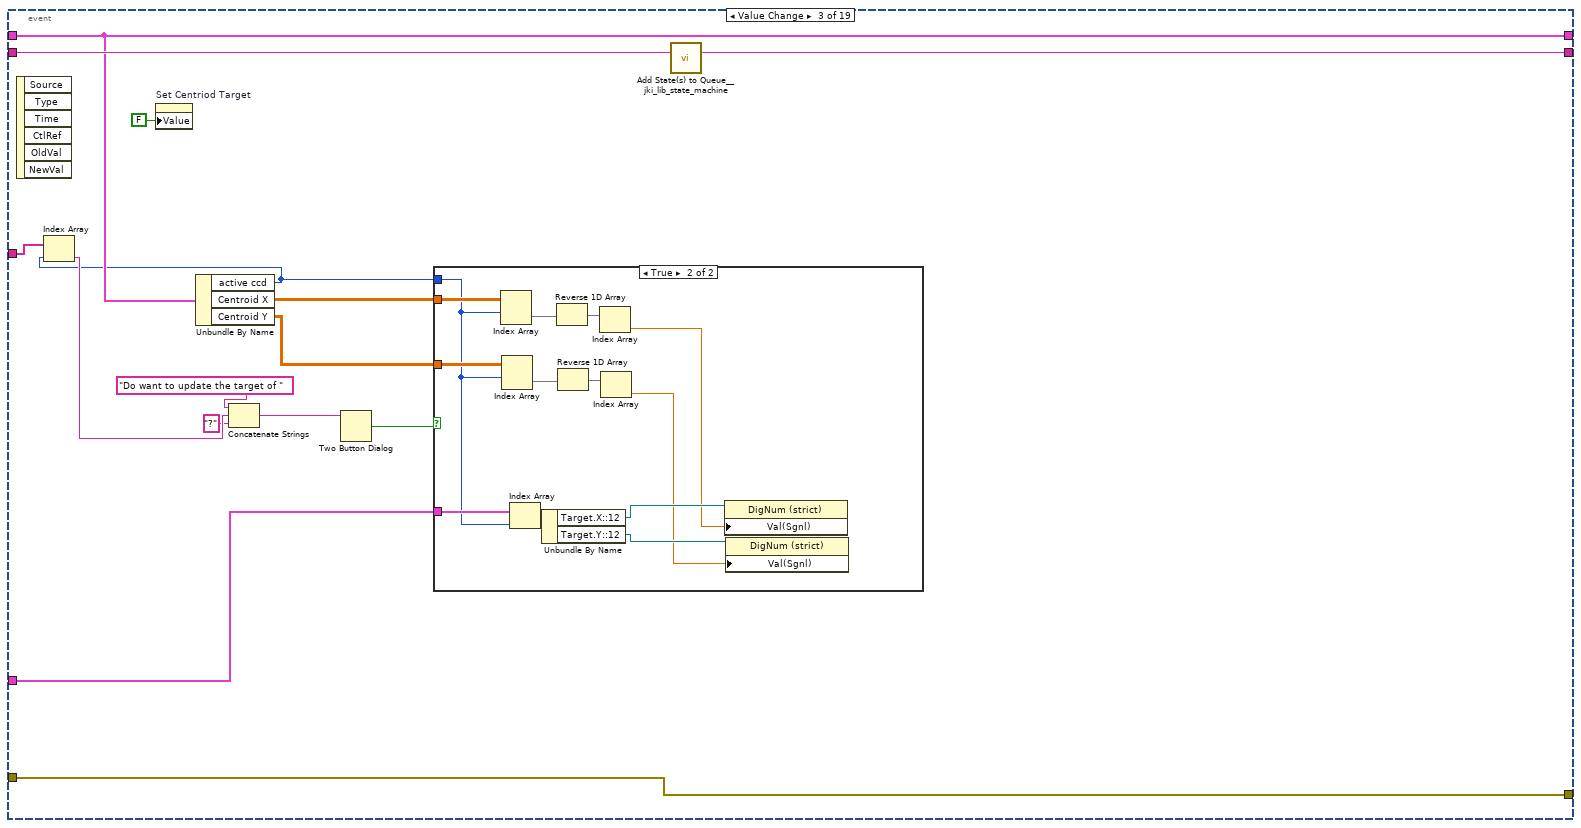
[diagram p9: hidden frame]
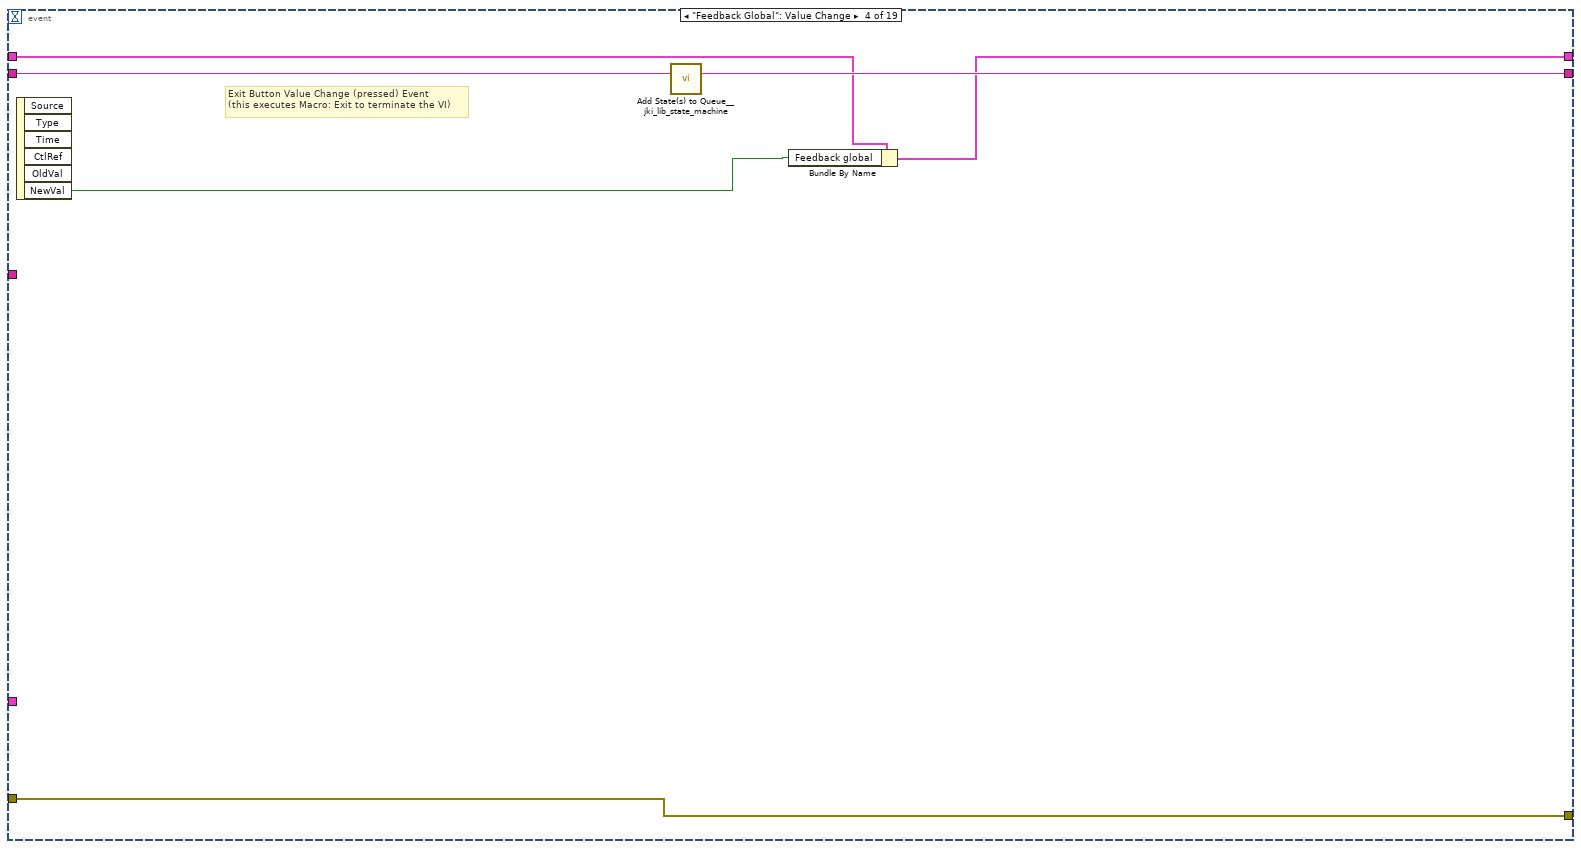
[diagram p11: hidden frame]
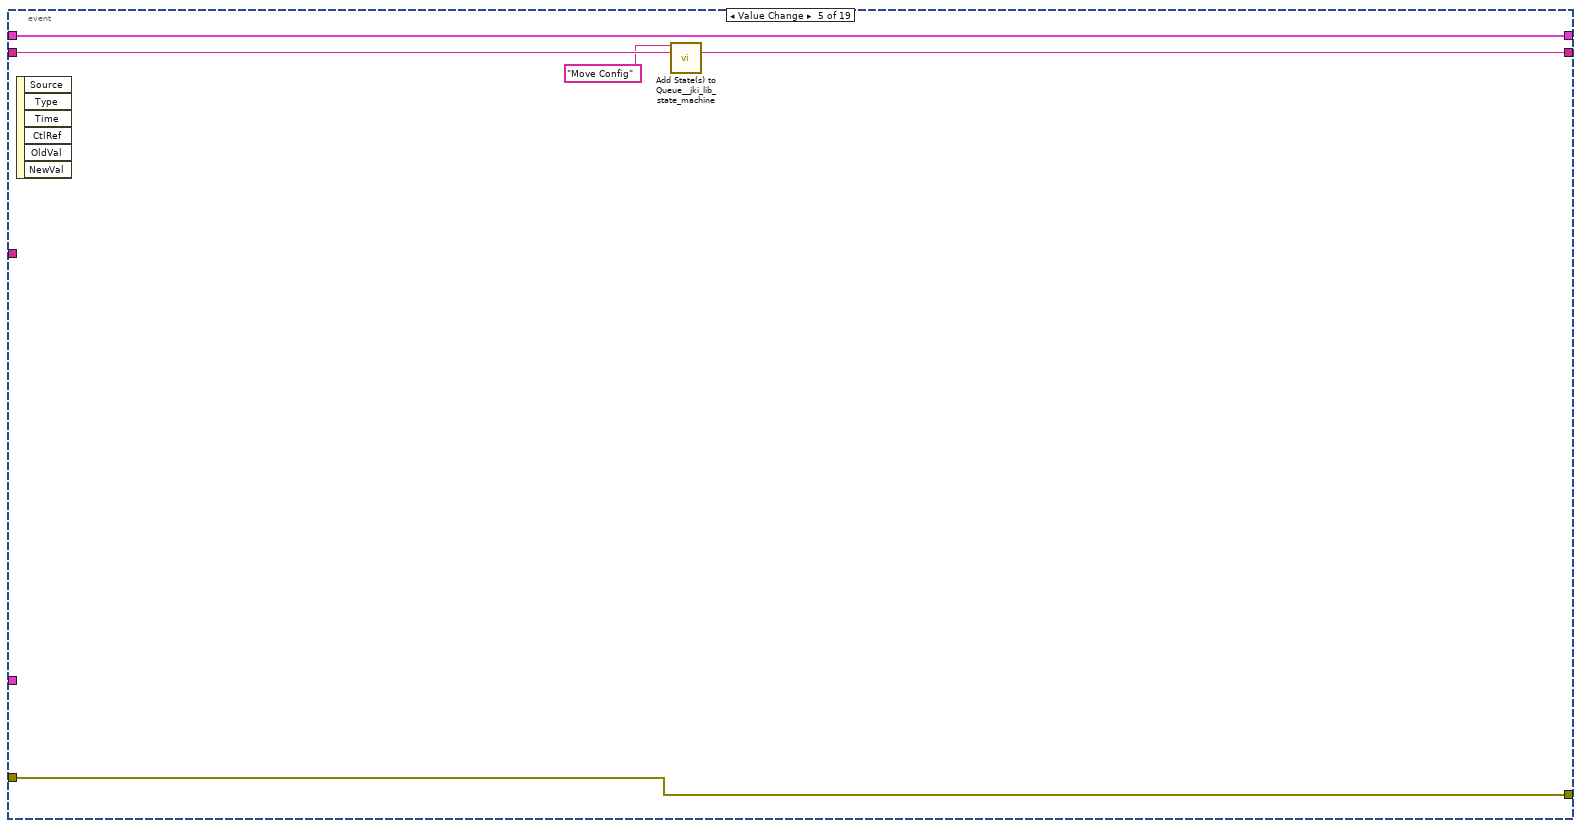
[diagram p12: hidden frame]
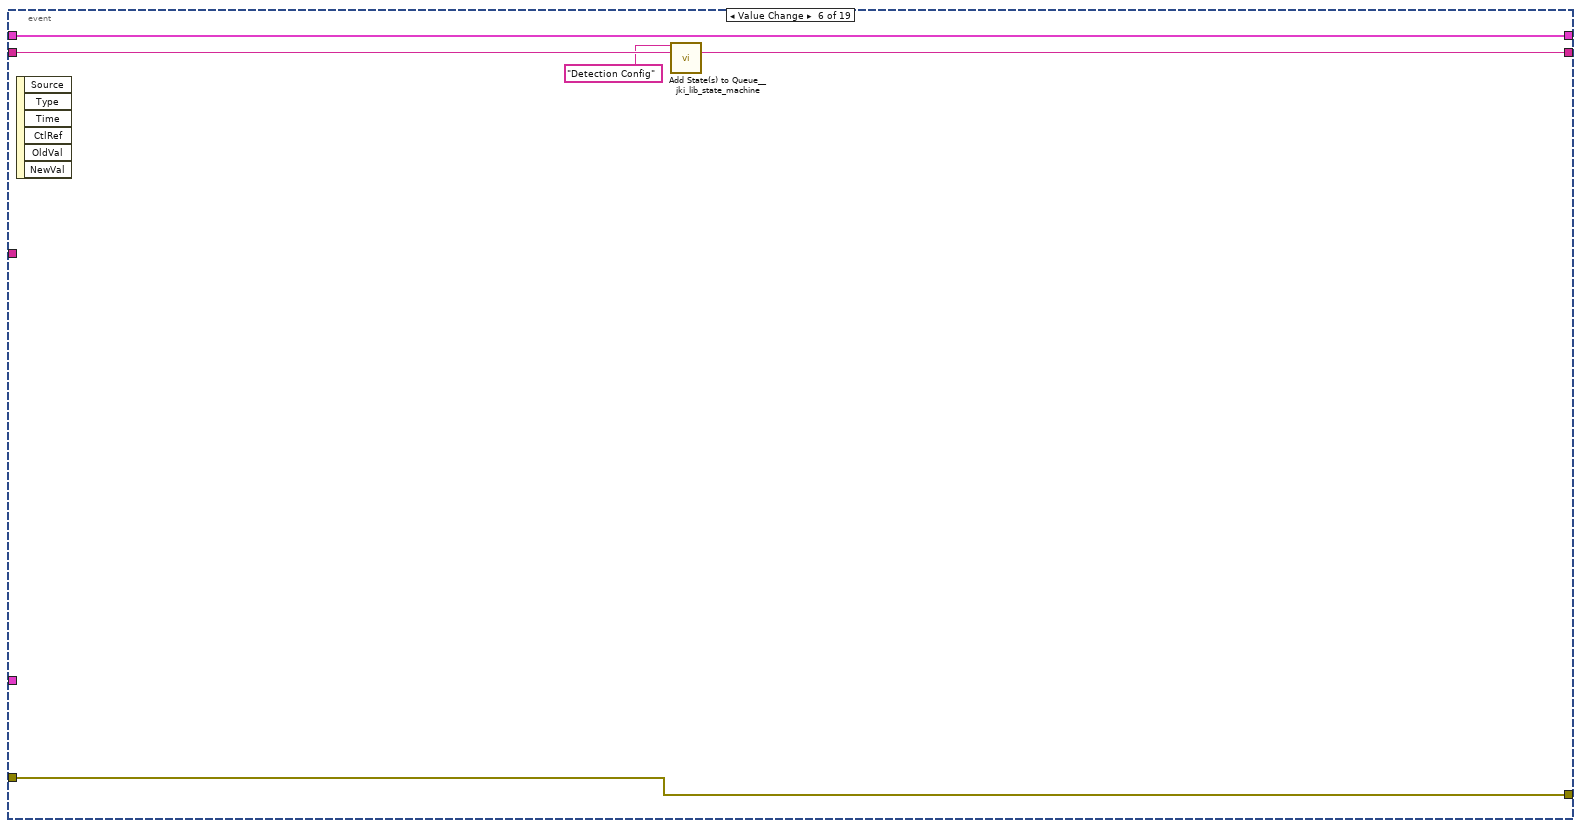
[diagram p13: hidden frame]
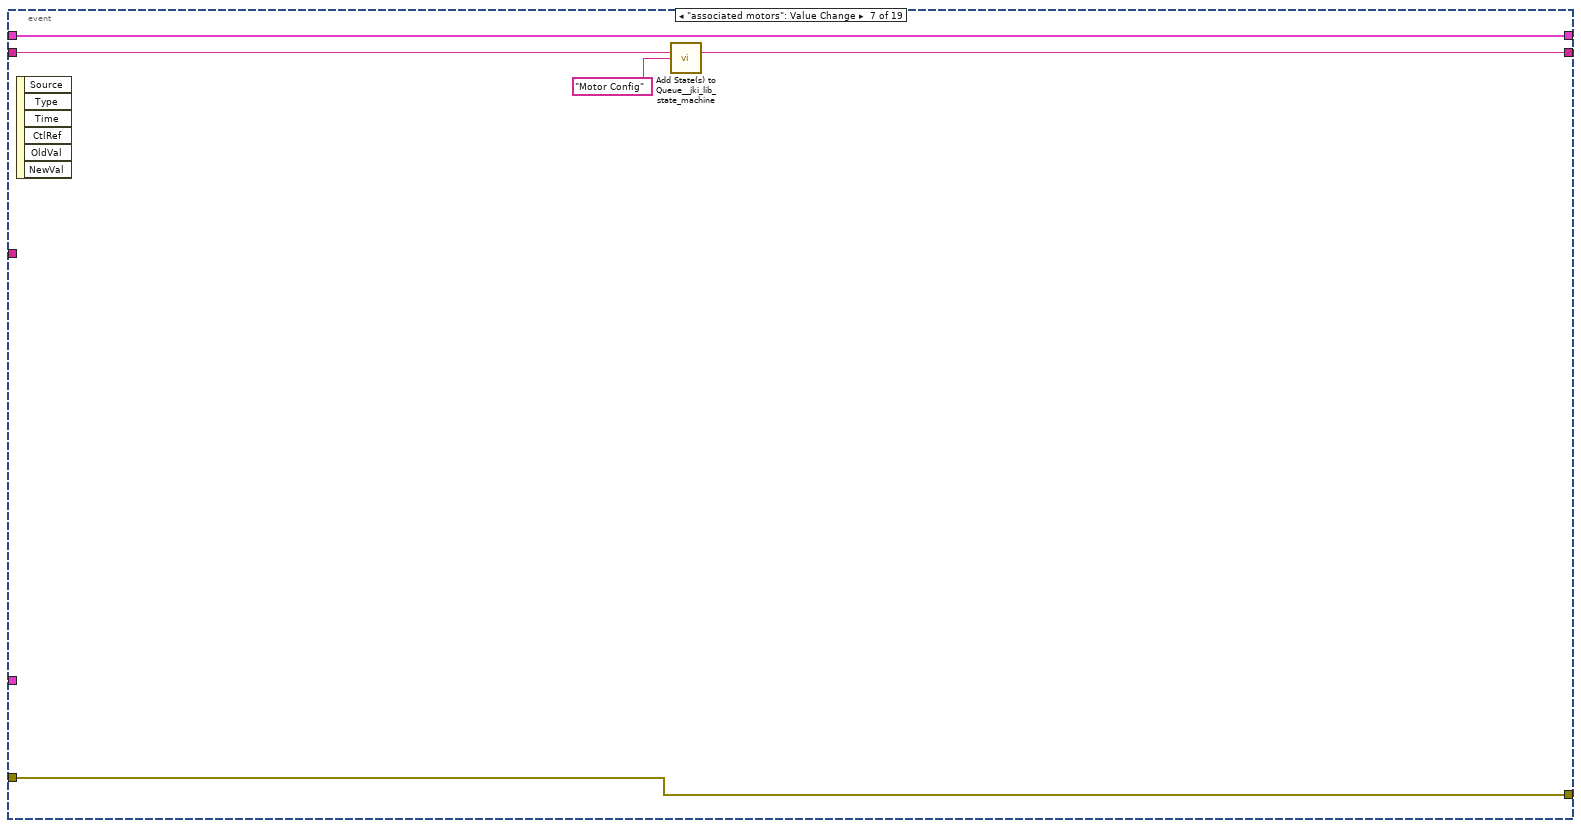
[diagram p14: hidden frame]
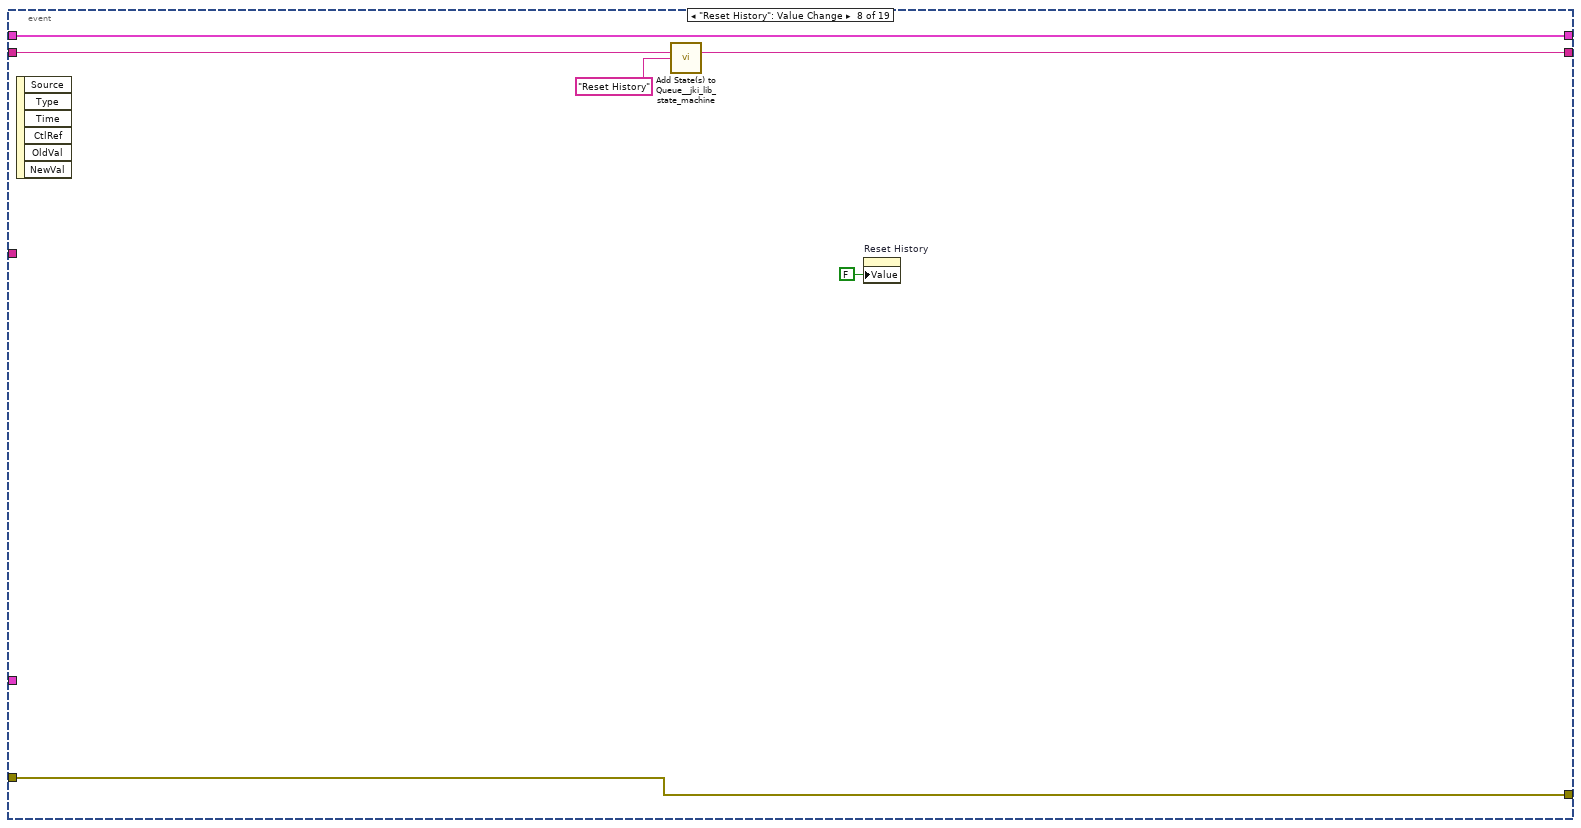
[diagram p15: hidden frame]
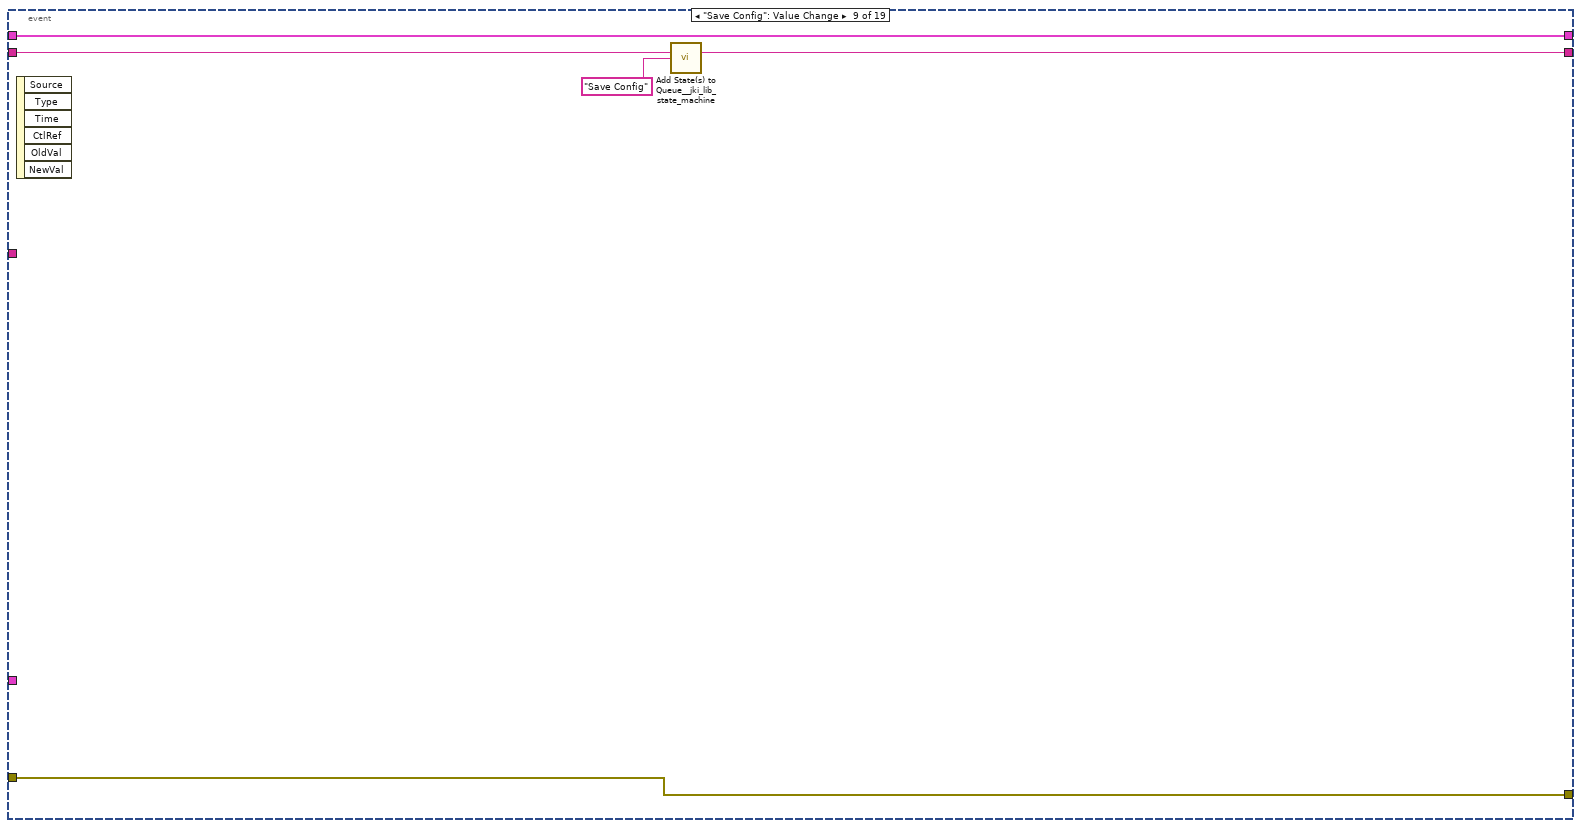
[diagram p16: hidden frame]
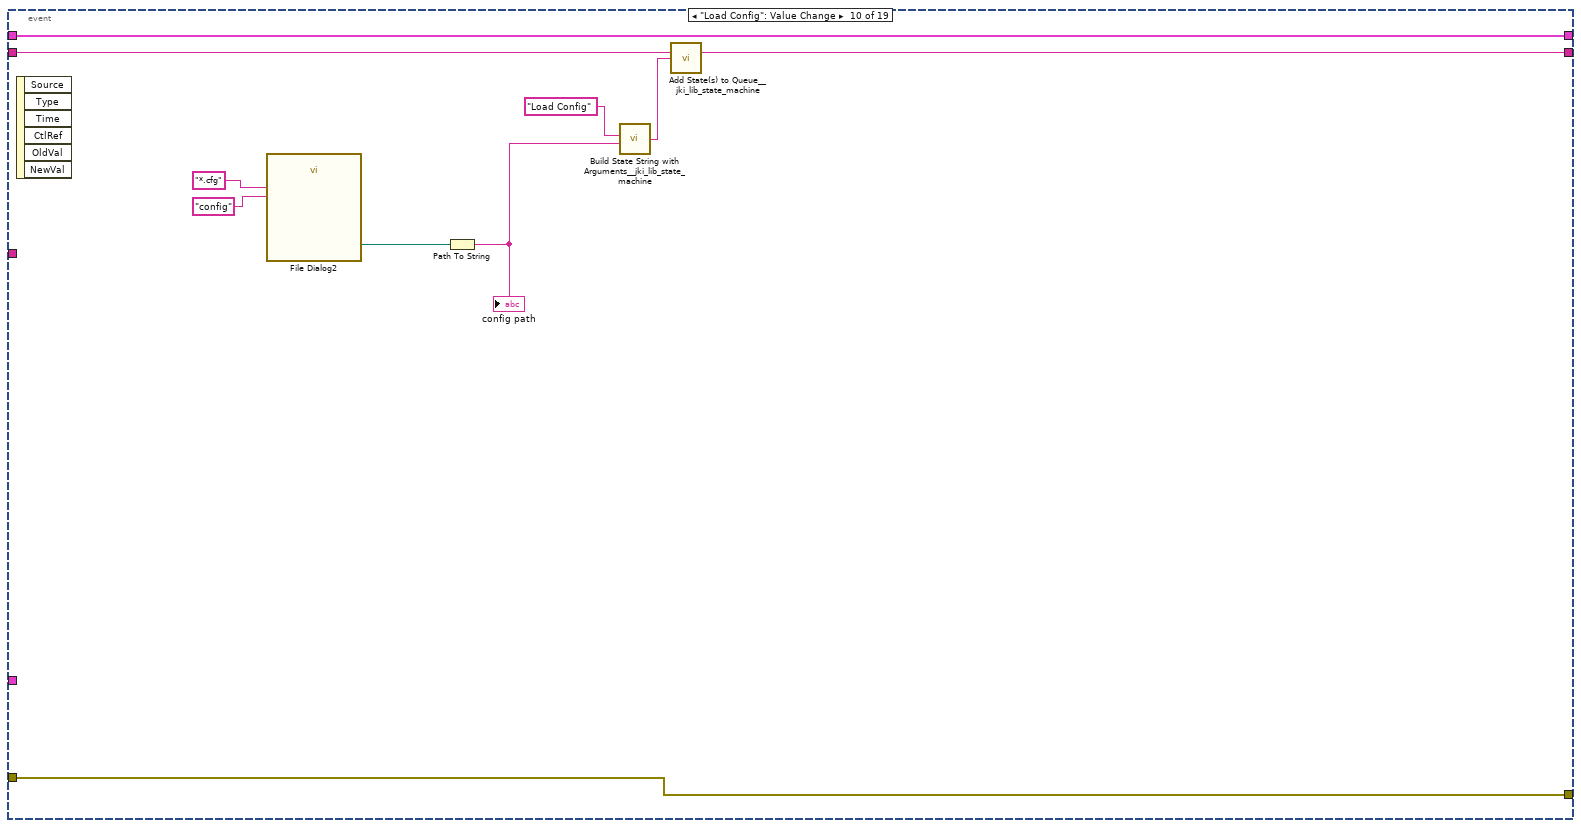
[diagram p17: hidden frame]
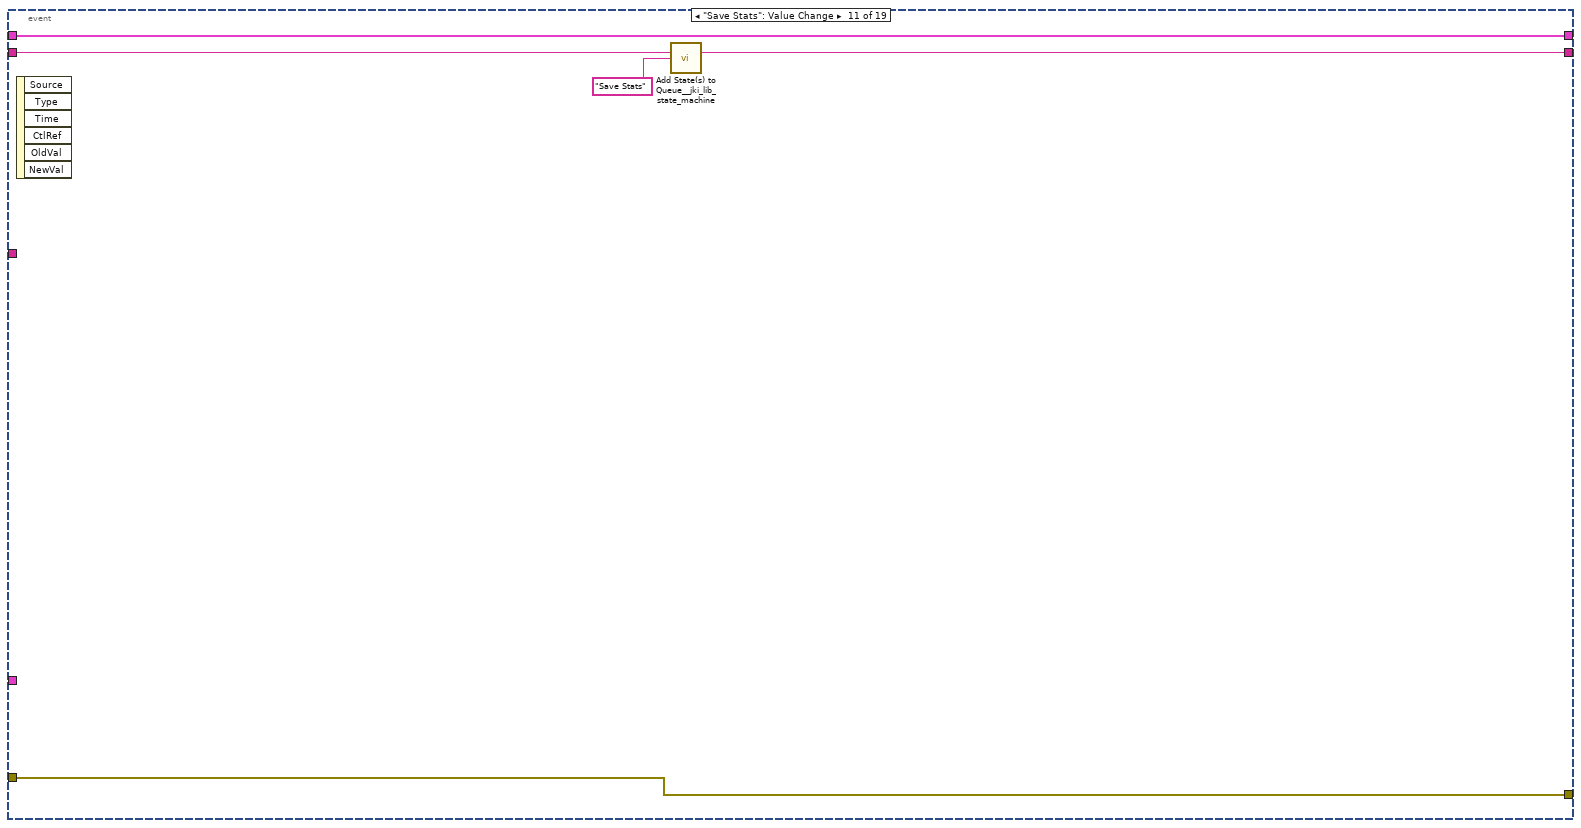
[diagram p18: hidden frame]
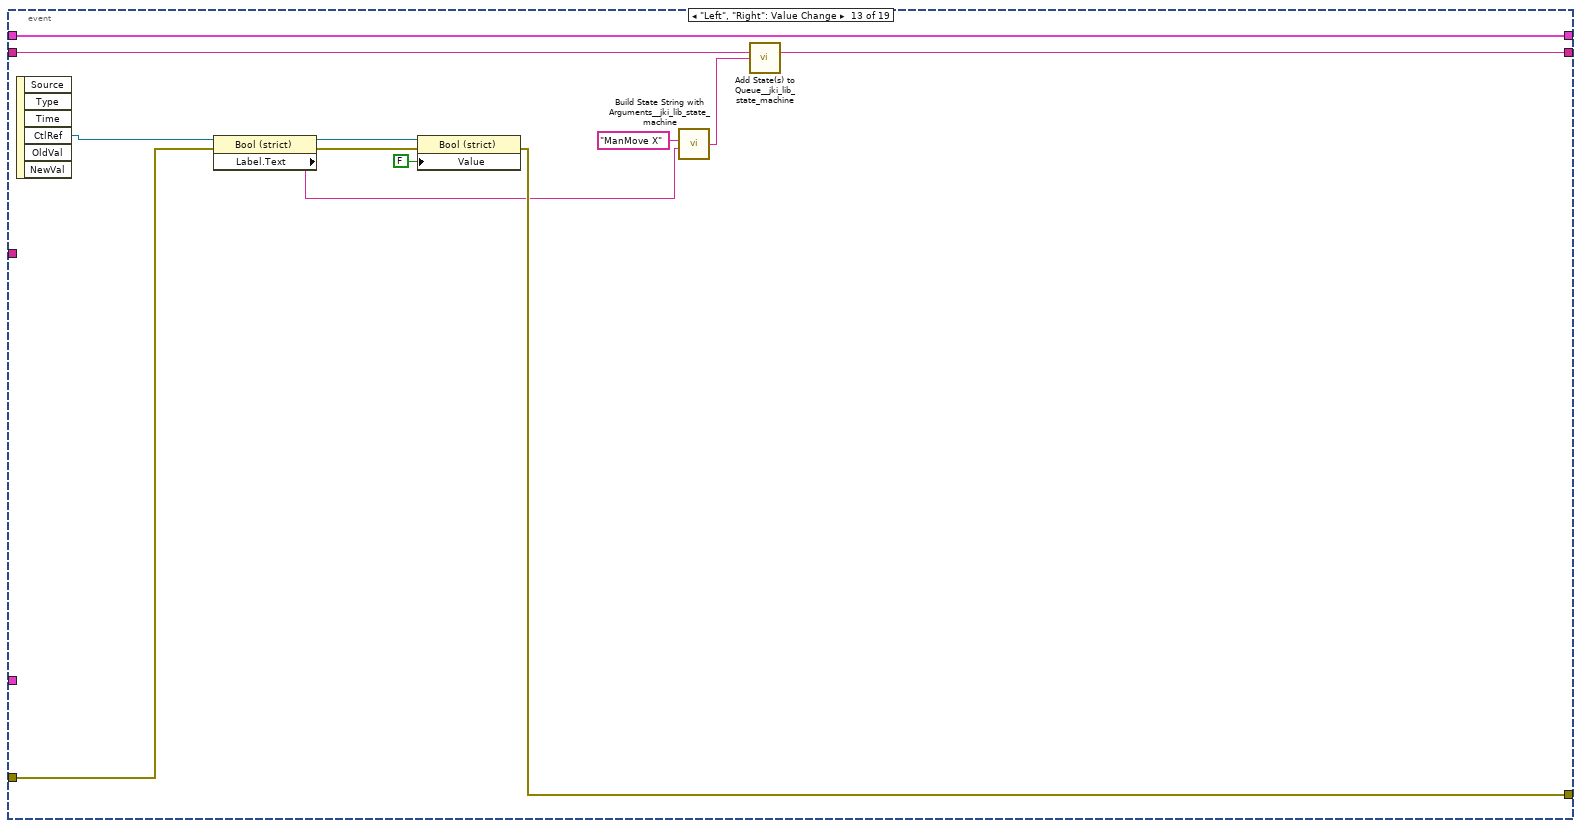
[diagram p19: hidden frame]
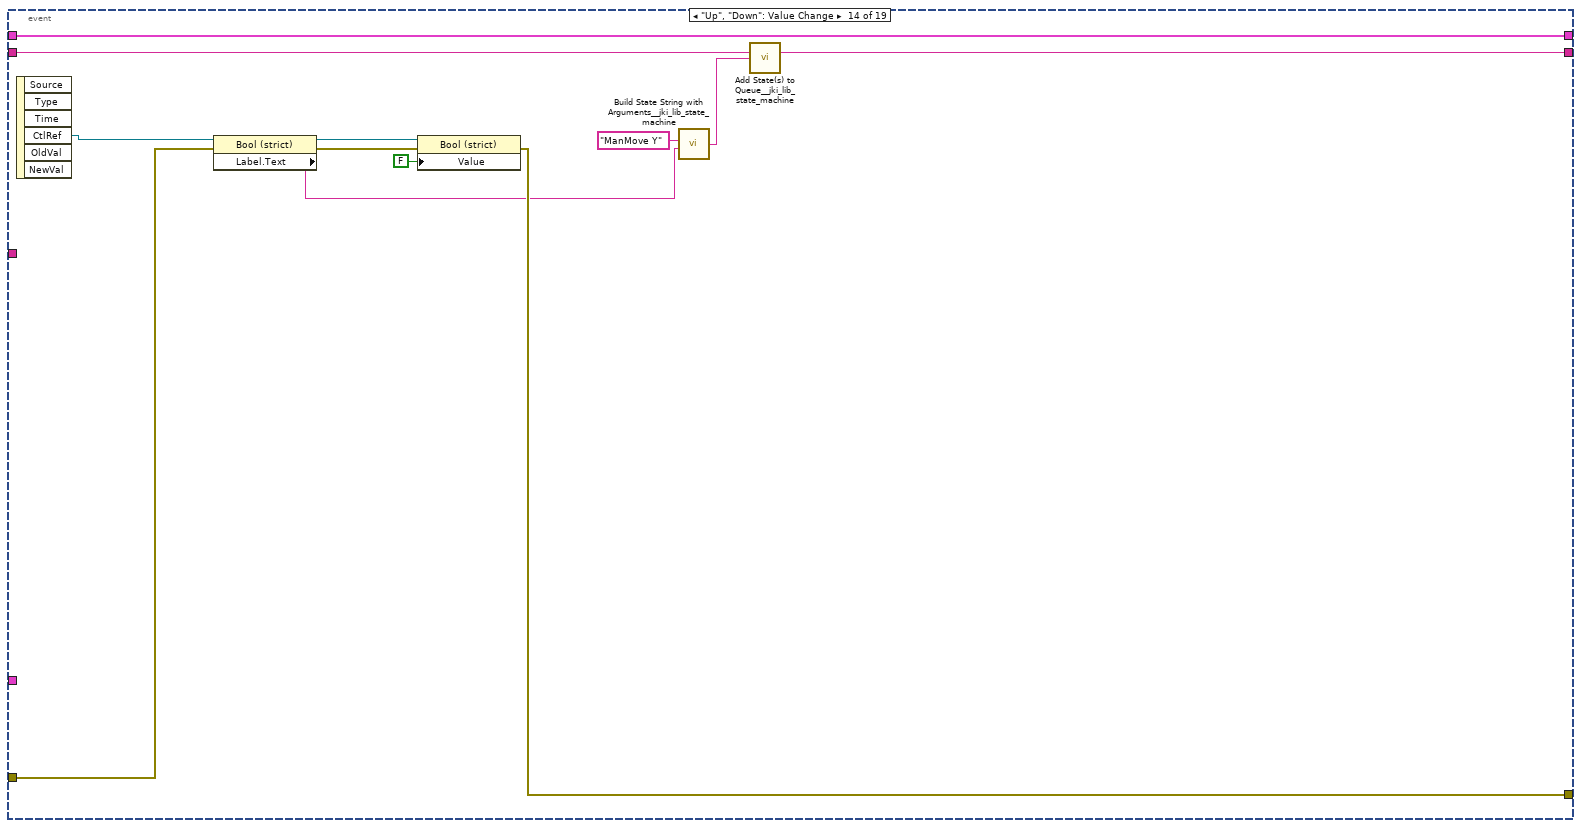
[diagram p20: hidden frame]
diagram:
  n1 = stacked-sequence {
    frame #0 {
      n2 = call <vilib>:"Application Directory.vi"() -> ("Application Directory"=w31:path)
      n3 = Build Path(base path=w31, name or relative path="defaultDevices_TRA.txt") -> (appended path=w29:path)
      "appended path" <- w29
      n4 = call-poly <vilib>:"Read From Spreadsheet File.vi"("file path (dialog if empty)"=w29) -> ("all rows"=w28:string[][])  [unwired: 6 in, 4 out]
      n5 = Index Array(array=w28, index (col) #1=0 ("disabled index (col)"), index (col) #2=1 ("index (col)")) -> (element #1=w25:string[])  [unwired: 2 in, 1 out]
      n6 = Index Array(array=w25, index #1=0 ("index"), index #2=1 ("index"), index #3=2 ("index"), index #4=3 ("index"), index #5=4 ("index"), index #6=5 ("index"), index #7=6 ("index"), index #8=7 ("index"), index #9=8 ("index"), index #10=9 ("index"), index #11=10 ("index"), index #12=11 ("index")) -> (element #1=w12:string, element #2=w11:string, element #3=w10:string, element #4=w9:string, element #5=w8:string, element #6=w7:string, element #7=w6:string, element #8=w5:string, element #9=w4:string, element #10=w3:string, element #11=w2:string, element #12=w1:string)
      n7 = property on="GUIdevice 1" class="Str"("Val(Sgnl)"=w12) -> ()  [unwired: 2 in, 2 out]
      n8 = property on="GUIdevice 2" class="Str"("Val(Sgnl)"=w11) -> ()  [unwired: 2 in, 2 out]
      n9 = property on="GUIdevice 3" class="Str"("Val(Sgnl)"=w10) -> ()  [unwired: 2 in, 2 out]
      n10 = property on="GUIdevice 4" class="Str"("Val(Sgnl)"=w9) -> ()  [unwired: 2 in, 2 out]
      n11 = property on="GUIdevice 5" class="Str"("Val(Sgnl)"=w8) -> ()  [unwired: 2 in, 2 out]
      n12 = property on="GUIdevice 6" class="Str"("Val(Sgnl)"=w7) -> ()  [unwired: 2 in, 2 out]
      n13 = property on="GUIdevice 7" class="Str"("Val(Sgnl)"=w6) -> ()  [unwired: 2 in, 2 out]
      n14 = property on="GUIdevice 8" class="Str"("Val(Sgnl)"=w5) -> ()  [unwired: 2 in, 2 out]
      n15 = property on="GUIdevice 9" class="Str"("Val(Sgnl)"=w4) -> ()  [unwired: 2 in, 2 out]
      n16 = property on="GUIdevice 10" class="Str"("Val(Sgnl)"=w3) -> ()  [unwired: 2 in, 2 out]
      n17 = property on="GUIdevice 11" class="Str"("Val(Sgnl)"=w2) -> ()  [unwired: 2 in, 2 out]
      n18 = property on="GUIdevice 12" class="Str"("Val(Sgnl)"=w1) -> ()  [unwired: 2 in, 2 out]
    }
    frame #1 {
      w34 = string[] ["M20", "SIM", "M22", ""] ("elements")
      w38 = T21 0 items=["Grayscale (U8)", "Grayscale (I16)", "Grayscale (SGL)", "Complex (CSG)", "RGB (U32)", "HSL (U32)", "RGB (U64)", "Grayscale (U16)"] ("Image Type")
      # "NOT FOR YOU MOFO"
      n19 = control-ref of="Position.Axis 1::99"() -> (w112:refnum<vi>)
      n20 = control-ref of="Position.Axis 2::99"() -> (w111:refnum<vi>)
      n21 = control-ref of="Position.Axis 3::99"() -> (w110:refnum<vi>)
      n22 = control-ref of="Position.Axis 4::99"() -> (w109:refnum<vi>)
      n23 = control-ref of="Position.Axis 5::99"() -> (w108:refnum<vi>)
      n24 = control-ref of="Position.Axis 6::99"() -> (w107:refnum<vi>)
      n25 = property on="Motor CCD 1" class="Ring (strict)"("Strings []"=w34) -> ()  [unwired: 2 in, 2 out]
      n26 = property on="Motor CCD 2" class="Ring (strict)"("Strings []"=w34) -> ()  [unwired: 2 in, 2 out]
      n27 = property on="Motor CCD 3" class="Ring (strict)"("Strings []"=w34) -> ()  [unwired: 2 in, 2 out]
      n28 = property on="Motor CCD 4" class="Ring (strict)"("Strings []"=w34) -> ()  [unwired: 2 in, 2 out]
      n29 = property on="Motor CCD 5" class="Ring (strict)"("Strings []"=w34) -> ()  [unwired: 2 in, 2 out]
      n30 = property on="Motor CCD 6" class="Ring (strict)"("Strings []"=w34) -> ()  [unwired: 2 in, 2 out]
      n31 = property on="Motor CCD 7" class="Ring (strict)"("Strings []"=w34) -> ()  [unwired: 2 in, 2 out]
      n32 = property on="Motor CCD 8" class="Ring (strict)"("Strings []"=w34) -> ()  [unwired: 2 in, 2 out]
      n33 = property on="Motor CCD 9" class="Ring (strict)"("Strings []"=w34) -> ()  [unwired: 2 in, 2 out]
      n34 = property on="Motor CCD 10" class="Ring (strict)"("Strings []"=w34) -> ()  [unwired: 2 in, 2 out]
      n35 = property on="Motor CCD 11" class="Ring (strict)"("Strings []"=w34) -> ()  [unwired: 2 in, 2 out]
      n36 = property on="Motor CCD 12" class="Ring (strict)"("Strings []"=w34) -> ()  [unwired: 2 in, 2 out]
      n37 = Build Array(w112, w111, w110, w109, w108, w107) -> (→"motor refs":refnum<vi>[])
      n38 = control-ref of="Target.X::1"() -> (w93:refnum<vi>)
      n39 = control-ref of="Target.Y::1"() -> (w92:refnum<vi>)
      n40 = control-ref of="Target.X::2"() -> (w91:refnum<vi>)
      n41 = control-ref of="Target.Y::2"() -> (w90:refnum<vi>)
      n42 = control-ref of="Target.X::3"() -> (w89:refnum<vi>)
      n43 = control-ref of="Target.Y::3"() -> (w88:refnum<vi>)
      n44 = control-ref of="Target.X::4"() -> (w87:refnum<vi>)
      n45 = control-ref of="Target.Y::4"() -> (w86:refnum<vi>)
      n46 = control-ref of="Target.X::5"() -> (w85:refnum<vi>)
      n47 = control-ref of="Target.Y::5"() -> (w84:refnum<vi>)
      n48 = control-ref of="Target.X::6"() -> (w83:refnum<vi>)
      n49 = control-ref of="Target.Y::6"() -> (w82:refnum<vi>)
      n50 = control-ref of="Target.X::7"() -> (w81:refnum<vi>)
      n51 = control-ref of="Target.Y::7"() -> (w80:refnum<vi>)
      n52 = control-ref of="Target.X::8"() -> (w79:refnum<vi>)
      n53 = control-ref of="Target.Y::8"() -> (w78:refnum<vi>)
      n54 = control-ref of="Target.X::9"() -> (w55:refnum<vi>)
      n55 = control-ref of="Target.Y::9"() -> (w54:refnum<vi>)
      n56 = control-ref of="Target.X::10"() -> (w53:refnum<vi>)
      n57 = control-ref of="Target.Y::10"() -> (w52:refnum<vi>)
      n58 = control-ref of="Target.X::11"() -> (w51:refnum<vi>)
      n59 = control-ref of="Target.Y::11"() -> (w50:refnum<vi>)
      n60 = control-ref of="Target.X::12"() -> (w49:refnum<vi>)
      n61 = control-ref of="Target.Y::12"() -> (w48:refnum<vi>)
      n62 = call "IMAQ Create"("Image Name"="GUIdevice 8", "Image Type"=w38) -> ("New Image"=→"image::8":T9)  [unwired: 3 in, 1 out]
      n63 = call "IMAQ Create"("Image Name"="GUIdevice 9", "Image Type"=w38) -> ("New Image"=→"image::9":T9)  [unwired: 3 in, 1 out]
      n64 = call "IMAQ Create"("Image Name"="GUIdevice 10", "Image Type"=w38) -> ("New Image"=→"image::10":T9)  [unwired: 3 in, 1 out]
      n65 = call "IMAQ Create"("Image Name"="GUIdevice 6", "Image Type"=w38) -> ("New Image"=→"image::6":T9)  [unwired: 3 in, 1 out]
      n66 = call "IMAQ Create"("Image Name"="GUIdevice 7", "Image Type"=w38) -> ("New Image"=→"image::7":T9)  [unwired: 3 in, 1 out]
      n67 = call "IMAQ Create"("Image Name"="GUIdevice 11", "Image Type"=w38) -> ("New Image"=→"image::11":T9)  [unwired: 3 in, 1 out]
      n68 = call "IMAQ Create"("Image Name"="GUIdevice 12", "Image Type"=w38) -> ("New Image"=→"image::12":T9)  [unwired: 3 in, 1 out]
      n69 = call "IMAQ Create"("Image Name"="GUIdevice 2") -> ("New Image"=→"image::2":T9)  [unwired: 4 in, 1 out]
      n70 = call "IMAQ Create"("Image Name"="GUIdevice 4", "Image Type"=w38) -> ("New Image"=→"image::4":T9)  [unwired: 3 in, 1 out]
      n71 = call "IMAQ Create"("Image Name"="GUIdevice 1", "Image Type"=w38) -> ("New Image"=→"image::1":T9)  [unwired: 3 in, 1 out]
      n72 = call "IMAQ Create"("Image Name"="GUIdevice 3", "Image Type"=w38) -> ("New Image"=→"image::3":T9)  [unwired: 3 in, 1 out]
      n73 = call "IMAQ Create"("Image Name"="GUIdevice 5", "Image Type"=w38) -> ("New Image"=→"image::5":T9)  [unwired: 3 in, 1 out]
      n74 = Build Array("GUIdevice 1", "GUIdevice 2", "GUIdevice 3", "GUIdevice 4", "GUIdevice 5", "GUIdevice 6", "GUIdevice 7", "GUIdevice 8", "GUIdevice 9", "GUIdevice 10", "GUIdevice 11", "GUIdevice 12") -> (w67:string[])
      "CCDs" <- w67
      n75 = property on="image::8" class="ImageControl"("Caption.Text"="GUIdevice 8") -> ()  [unwired: 2 in, 2 out]
      n76 = property on="image::10" class="ImageControl"("Caption.Text"="GUIdevice 10") -> ()  [unwired: 2 in, 2 out]
      n77 = property on="image::9" class="ImageControl"("Caption.Text"="GUIdevice 9") -> ()  [unwired: 2 in, 2 out]
      n78 = property on="image::1" class="ImageControl"("Caption.Text"="GUIdevice 1") -> ()  [unwired: 2 in, 2 out]
      n79 = property on="image::2" class="ImageControl"("Caption.Text"="GUIdevice 2") -> ()  [unwired: 2 in, 2 out]
      n80 = property on="image::3" class="ImageControl"("Caption.Text"="GUIdevice 3") -> ()  [unwired: 2 in, 2 out]
      n81 = property on="image::4" class="ImageControl"("Caption.Text"="GUIdevice 4") -> ()  [unwired: 2 in, 2 out]
      n82 = property on="image::5" class="ImageControl"("Caption.Text"="GUIdevice 5") -> ()  [unwired: 2 in, 2 out]
      n83 = property on="image::6" class="ImageControl"("Caption.Text"="GUIdevice 6") -> ()  [unwired: 2 in, 2 out]
      n84 = property on="image::7" class="ImageControl"("Caption.Text"="GUIdevice 7") -> ()  [unwired: 2 in, 2 out]
      n85 = property on="image::11" class="ImageControl"("Caption.Text"="GUIdevice 11") -> ()  [unwired: 2 in, 2 out]
      n86 = property on="image::12" class="ImageControl"("Caption.Text"="GUIdevice 12") -> ()  [unwired: 2 in, 2 out]
      n87 = Array To Cluster(array=w67) -> (cluster=→"Cameras":T22)
      n88 = Bundle("Target.X::1"=w93, "Target.Y::1"=w92) -> (w77:T23)  [unwired: 1 in]
      n89 = Bundle("Target.X::2"=w91, "Target.Y::2"=w90) -> (w76:T24)  [unwired: 1 in]
      n90 = Bundle("Target.X::3"=w89, "Target.Y::3"=w88) -> (w75:T25)  [unwired: 1 in]
      n91 = Bundle("Target.X::4"=w87, "Target.Y::4"=w86) -> (w68:T26)  [unwired: 1 in]
      n92 = Bundle("Target.X::5"=w85, "Target.Y::5"=w84) -> (w74:T27)  [unwired: 1 in]
      n93 = Bundle("Target.X::6"=w83, "Target.Y::6"=w82) -> (w73:T28)  [unwired: 1 in]
      n94 = Bundle("Target.X::7"=w81, "Target.Y::7"=w80) -> (w72:T29)  [unwired: 1 in]
      n95 = Bundle("Target.X::8"=w79, "Target.Y::8"=w78) -> (w71:T30)  [unwired: 1 in]
      n96 = Bundle("Target.X::12"=w49, "Target.Y::12"=w48) -> (w44:T31)  [unwired: 1 in]
      n97 = Bundle("Target.X::9"=w55, "Target.Y::9"=w54) -> (w47:T32)  [unwired: 1 in]
      n98 = Bundle("Target.X::10"=w53, "Target.Y::10"=w52) -> (w46:T33)  [unwired: 1 in]
      n99 = Bundle("Target.X::11"=w51, "Target.Y::11"=w50) -> (w45:T34)  [unwired: 1 in]
      n100 = property on="CCDs" class="Ring (strict)"("Strings []"=w67) -> ()  [unwired: 2 in, 2 out]
      n101 = Build Array(w77, w76, w75, w68, w74, w73, w72, w71, w47, w46, w45, w44) -> (w70:T35)
      n102 = Tick Count (ms)() -> (millisecond timer value=→"millisecond timer value":u32)
      n103 = property on="Feedback Global" class="Bool (strict)"("Value"=FALSE ("Feedback Global")) -> ()  [unwired: 2 in, 2 out]
      n104 = Get Date/Time In Seconds() -> (seconds since 1Jan1904=w57:timestamp)
      n105 = Format Date/Time String(time format string (%c)="%Y%m%d%H%M", seconds (now)=w57) -> (date/time string=w56:string)  [unwired: 1 in]
      n106 = Concatenate Strings(w56, "Beampointing_TRA.tdms" ("string")) -> (w60:string)
      n107 = String To Path(string=w60) -> (path=w59:path)
      n108 = Build Path(base path=path "W:/BP_DATA", name or relative path=w59) -> (appended path=w62:path)
      n109 = call <vilib>:"Add State(s) to Queue__jki_lib_state_machine.vi"("State(s) in (\"\")"="Macro: Initialize") -> ("States Out"=w114:string)  [unwired: 14 in]
      n110 = Create User Event(user event datatype=T14 {"EventEnum"=enum."new data", "Device name"="Device name"} ("New Event")) -> (user event=w122:refnum<user-event>, error out=w124:errorcluster)  [unwired: 1 in]
      "tcp data event" <- w122
      n111 = while "JKI - String-Based Queued State Machine (Basic) v1.0" {
        shift-right: [w141] -> w66
        shift-left: _ -> [w134]
        shift-right: [w144] -> w94
        shift-left: _ -> [w140]
        shift-right: [w143] -> _
        shift-left: w114 -> [w145]
        tunnel: w70 -> [w138]
        tunnel: w67 -> [w136]
        tunnel: [w136] -> w95
        tunnel: w70 -> [w137]
        tunnel: w62 -> [w132]
        stop <- w142 stop-if-true
        n112 = Unbundle By Name(w134) -> ("active cams"=w133:string[])
        n113 = call <vilib>:"Parse State Queue__jki_lib_state_machine.vi"("State Queue"=w145, "Error In (no error)"=w140) -> ("Remaining States"=w147:string, "Current State"=w148:string, "Arguments"=w146:string)  [unwired: 11 in]
        "Current State" <- w148
        n114 = case shown="\"Check Move\"" w148 {
          selector: w148 -> [_ _ w443 _ _ _ _ _ _ _ _ _ _ _ _ _ _ _ _ _ _ _ _ _ _ _ _ _ _ _ _ _ _ _ _ _ _ _ _ _ _ _]
          tunnel: w147 -> [w173 w442 w447 w465 w471 w476 w480 w522 w528 w532 w536 w542 w553 w577 w586 w596 w600 w624 w725 w777 w807 w816 w838 w859 w863 w879 w1024 w1163 w1243 w1307 w1378 w1454 w1478 w1493 w1576 w1628 w1638 w1673 w1714 w1734 w1745 w1768]
          tunnel: w146 -> [_ _ _ _ _ _ _ _ _ _ _ w537 w548 _ _ _ _ w617 w678 _ w792 _ _ _ _ w880 _ w1138 w1229 w1293 w1353 w1448 _ _ _ _ _ _ _ _ w1749 _]
          tunnel: w134 -> [w171 w439 w445 w455 w468 w474 w477 _ w523 w529 w534 w540 w547 w574 w583 w588 w597 w614 w715 w775 w788 w812 w830 w852 w860 w868 w1005 w1156 w1239 w1303 w1371 w1450 w1475 w1490 w1556 w1625 w1635 w1646 w1700 w1731 w1748 w1759]
          tunnel: [w170 w440 w449 w463 errorcluster {"status"=FALSE, "code"=0, "source"=""} ("error out") w473 w478 w484 w525 w530 w533 w538 w550 w575 w584 w594 w598 w618 w681 w766 w796 w814 w836 w857 w861 w913 w1037 w1161 w1241 w1305 w1376 w1443 w1476 w1491 w1569 w1626 w1636 w1671 w1692 w1732 w1743 w1766] -> w144
          tunnel: w140 -> [w169 w440 w448 w463 w467 w473 w478 w485 w526 w530 w533 w539 w551 w575 w584 w594 w598 w619 w679 w767 w795 w814 w836 w857 w861 w913 w1037 w1161 w1241 w1305 w1376 w1444 w1476 w1491 w1570 w1626 w1636 w1671 w1694 w1732 w1743 w1766]
          tunnel: [w172 w441 w446 w464 w470 w475 w479 w521 w527 w531 w535 w541 w552 w576 w585 w595 w599 w608 w724 w776 w806 w815 w837 w858 w862 w884 w1038 w1162 w1242 w1306 w1377 w1453 w1477 w1492 w1575 w1627 w1637 w1672 w1713 w1733 w1744 w1767] -> w143
          tunnel: [_ _ _ _ _ TRUE _ _ _ _ _ _ _ _ _ _ _ _ _ _ _ _ _ _ _ _ _ _ _ _ _ _ _ _ _ _ _ _ _ _ _ _] -> w142
          tunnel: [w166 w439 w445 w454 w468 w474 w477 w491 w523 w529 w534 w540 w547 w574 w583 w588 w597 w621 w714 w775 w801 w811 w829 w851 w860 w906 w1004 w1156 w1239 w1303 w1371 w1452 w1475 w1490 w1556 w1624 w1635 w1646 w1699 w1731 w1747 w1758] -> w141
          tunnel: "update speed [ms]" -> [w168 _ _ _ _ _ _ _ _ _ _ _ _ _ _ _ _ _ _ _ _ _ _ _ _ _ _ _ _ _ _ _ _ _ _ _ _ _ _ _ _ _]
          tunnel: w138 -> [w165 _ _ _ _ _ _ _ _ _ _ _ _ _ _ _ _ _ _ _ _ _ _ _ _ w904 _ _ _ _ _ _ _ _ _ _ _ _ _ w1716 _ _]
          tunnel: w136 -> [w167 _ _ _ _ _ _ _ _ _ _ _ _ _ _ _ _ w623 w713 _ w802 _ _ _ _ w872 w1003 w1160 _ _ w1375 w1449 _ w1479 _ _ _ w1645 _ _ _ _]
          tunnel: w132 -> [_ _ _ _ _ _ _ w483 _ _ _ _ _ _ _ _ _ w620 _ _ _ _ _ _ _ _ _ _ _ _ _ _ _ _ _ _ _ _ _ _ _ _]
          frame "", "Idle" {
            # "executes when the state queue is empty"
            n115 = event shown="[11] \"active CCDs\": Value Change" {
              selector: _ -> [_ _ _ _ _ _ _ _ _ _ _ _ _ _ _ _ _ _ _]
              dyn-events: _ -> [_ _ _ _ _ _ _ _ _ _ _ _ _ _ _ _ _ _ _]
              timeout: w168 -> [_ _ _ _ _ _ _ _ _ _ _ _ _ _ _ _ _ _ _]
              tunnel: w173 -> [w212 w300 w315 w334 w339 w344 w349 w355 w360 w370 w375 w384 w396 w408 w413 w418 w424 w428 w438]
              tunnel: [w199 w299 w314 w333 w338 w343 w348 w354 w359 w369 w374 w383 w395 w407 w412 w417 w423 w426 w437] -> w172
              tunnel: w171 -> [w195 w297 w311 w330 w336 w341 w346 w352 w357 w367 w372 w377 w394 w406 w411 w416 w422 w429 w435]
              tunnel: [w211 w298 w313 w332 w337 w342 w347 w353 w358 w368 w373 w382 w389 w401 w410 w415 w421 w425 w436] -> w170
              tunnel: w169 -> [w186 w298 w313 w332 w337 w342 w347 w353 w358 w368 w373 w382 w390 w402 w410 w415 w421 w425 w436]
              tunnel: [w198 w297 w311 w329 w336 w341 w346 w352 w357 w367 w372 w377 w394 w406 w411 w416 w422 w429 w435] -> w166
              tunnel: w167 -> [w191 _ w307 _ _ _ _ _ _ _ _ _ _ _ _ _ _ _ _]
              tunnel: w165 -> [_ _ w309 _ _ _ _ _ _ _ _ _ _ _ _ _ _ _ _]
              event Timeout {
                n116 = event-data() -> ()  [unwired: 1 in, 1 out]
                n117 = Unbundle By Name(w195) -> ("Centroid X"=w192:dbl[][], "Centroid Y"=w189:dbl[][], "Size"=w187:dbl[][], "detection para"=w182:T3[], "active cams"=w190:string[], "thresholds"=w188:cluster{"Lower value":sgl, "Upper value":sgl}[])
                n118 = Unbundle By Name(w195) -> ("active ccd"=w194:i32)
                n119 = for {
                  tunnel: w190 -> [w233] mode=indexing
                  tunnel: [w234] -> w177 mode=indexing
                  tunnel: w191 -> [w256]
                  tunnel: w182 -> [w254]
                  tunnel: [w217] -> w176 mode=indexing
                  tunnel: [w252] -> w185 mode=indexing
                  tunnel: [w250] -> w193 mode=indexing
                  tunnel: "autodetect" -> [w244]
                  tunnel: w186 -> [w257]
                  tunnel: [w258] -> w184
                  shift-right: [w241] -> w181
                  shift-left: w188 -> [w243]
                  shift-right: [w228] -> w180
                  shift-left: w192 -> [w230]
                  shift-right: [w224] -> w179
                  shift-left: w189 -> [w226]
                  shift-right: [w218] -> w178
                  shift-left: w187 -> [w220]
                  w222 = 0 ("index")
                  n120 = call-poly <userlib>:"Filter 1D Array__ogtk.vi"("items to filter"=w233, "array"=w256) -> ("filtered item indices"=w255:i32[])  [unwired: 4 in, 1 out]
                  n121 = Index Array(array=w255) -> (element=w219:i32)  [unwired: 1 in]
                  n122 = Index Array(array=w220, index (row)=w219) -> (element=w248:dbl[])  [unwired: 1 in]
                  n123 = Index Array(array=w226, index (row)=w219) -> (element=w249:dbl[])  [unwired: 1 in]
                  n124 = Index Array(array=w243, index=w219) -> (element=w247:cluster{"Lower value":sgl, "Upper value":sgl})
                  n125 = Index Array(array=w230, index (row)=w219) -> (element=w232:dbl[])  [unwired: 1 in]
                  n126 = Index Array(array=w254, index=w219) -> (element=w251:T3)
                  n127 = call "CENTRIOD DETECTION.vi"("Refnum in"=w233, "auto threshold"=w244, "Threshold Range In"=w247, "beam detection para"=w251, "error in (no error)"=w257) -> ("Bounding Rect"=w250:T36, "Particle Reports (Pixels)"=w252:T1, "Threshold Range Out"=w242:cluster{"Lower value":sgl, "Upper value":sgl}, "Centriod"=w259:cluster{"X":dbl, "Y":dbl}, "error out"=w258:errorcluster)  [unwired: 7 in, 3 out]
                  n128 = Unbundle By Name(w259) -> ("X"=w231:dbl, "Y"=w227:dbl)
                  n129 = Empty Array?(array=w252) -> (empty?=w253:bool)
                  n130 = Not(x=w253) -> (.not. x?=w217:bool)
                  n131 = Replace Array Subset(array=w243, new element=w242, index=w219) -> (w241:cluster{"Lower value":sgl, "Upper value":sgl}[])
                  n132 = Unbundle By Name(w250) -> ("Right"=w240:dbl, "Left"=w239:dbl, "Bottom"=w238:dbl, "Top"=w237:dbl)
                  n133 = Subtract(x=w240, y=w239) -> (x-y=w235:dbl)
                  n134 = Subtract(x=w238, y=w237) -> (x-y=w236:dbl)
                  n135 = Multiply(x=w235, y=w236) -> (x*y=w223:dbl)
                  n136 = Insert Into Array(array=w249, index=w222, new element=w227) -> (w225:dbl[])
                  n137 = Insert Into Array(array=w232, index=w222, new element=w231) -> (w229:dbl[])
                  n138 = Insert Into Array(array=w248, index=w222, new element=w223) -> (w221:dbl[])
                  n139 = for {
                    shift-right: [w260] -> w245
                    shift-left: dbl[] [] ("Array 4") -> [w263]
                    tunnel: w225 -> [w261] mode=indexing
                    n140 = Equal To 0?(x=w261) -> (x = 0?=w262:bool)
                    n141 = case shown="False" w262 {
                      tunnel: w263 -> [w266 w267]
                      tunnel: w261 -> [w265 _]
                      tunnel: [w264 w267] -> w260
                      frame False {
                        n142 = Build Array (concatenate)(w266, w265) -> (w264:dbl[])
                      }
                      frame True {
                      }
                    }
                  }
                  n143 = Replace Array Subset(array=w230, new element=w229, index (row)=w219) -> (w228:dbl[][])  [unwired: 1 in]
                  n144 = Replace Array Subset(array=w226, new element=w225, index (row)=w219) -> (w224:dbl[][])  [unwired: 1 in]
                  n145 = Replace Array Subset(array=w220, new element=w221, index (row)=w219) -> (w218:dbl[][])  [unwired: 1 in]
                  n146 = Array Size(array=w245) -> (size(s)=w234:i32)
                }
                "detected" <- w176
                "Box" <- w193
                n147 = Bundle(0, 1, "Centroid X"=w192) -> (→"Status":cluster{i32, i32, "Centroid X":dbl[][]})  [unwired: 1 in]
                n148 = Index Array(array=w185, index (row)=w194) -> (element=→"particles":T1)  [unwired: 1 in]
                n149 = call <vilib>:"Clear Errors.vi"("error in (no error)"=w184) -> ("error out"=w211:errorcluster)  [unwired: 5 in, 1 out]
                n150 = local read "img to avg"() -> (w201:i32)
                n151 = local read "Numeric"() -> (w204:dbl)
                n152 = Increment(x=w201) -> (x+1=w200:i32)
                n153 = Greater Or Equal?(x=w204, y=w200) -> (x >= y?=w197:bool)
                n154 = Increment(x=w204) -> (x+1=w203:dbl)
                n155 = Select(t=0.0, s=w197, f=w203) -> (s? t:f=w202:dbl)
                n156 = local write "Numeric"(w202) -> ()
                n157 = Bundle By Name(cluster=w195, "thresholds"=w181) -> (w207:T37)
                n158 = for {
                  tunnel: w177 -> [w288] mode=indexing
                  tunnel: w190 -> [w295] mode=indexing
                  shift-right: [w290] -> w213
                  shift-left: "" ("GUIdevice 7") -> [w293]
                  tunnel: [w283] -> w215 mode=indexing
                  tunnel: "Detection Rate" -> [w287]
                  tunnel: w202 -> [w285]
                  n159 = local read "img to avg"() -> (w289:i32)
                  n160 = Greater Or Equal?(x=w288, y=w289) -> (x >= y?=w284:bool)
                  n161 = Multiply(x=w287, y=w285) -> (x*y=w286:dbl)
                  n162 = Greater Or Equal?(x=w288, y=w286) -> (x >= y?=w282:bool)
                  n163 = And(x=w284, y=w282) -> (x .and. y?=w283:bool)
                  n164 = Select(t=w295, s=w283, f="") -> (s? t:f=w291:string)
                  n165 = Concatenate Strings(w293, "\t", w291) -> (w290:string)
                }
                n166 = Bundle By Name(cluster=w207, "Centroid X"=w180, "Centroid Y"=w179, "Size"=w178) -> (w175:T37)
                n167 = Unbundle By Name(w175) -> ("img to avg"=w174:i32)
                n168 = case shown="True" w197 {
                  tunnel: w175 -> [w268 w275]
                  tunnel: [w268 w274] -> w198
                  tunnel: w174 -> [_ w270]
                  frame False {
                  }
                  frame True {
                    n169 = Decrement(x=w270) -> (x-1=w273:i32)
                    n170 = Initialize Array(0.0 ("element"), 12 ("dimension size"), w273) -> (w269:dbl[][])
                    n171 = Bundle By Name(cluster=w275, "Centroid X"=w269, "Centroid Y"=w269, "Size"=w269) -> (w274:T37)
                  }
                }
                n172 = Or Array Elements(Boolean array=w215) -> (logical OR=w214:bool)
                n173 = case shown="True" w214 {
                  tunnel: w213 -> [_ w280]
                  tunnel: w212 -> [w276 w278]
                  tunnel: [w276 w277] -> w199
                  frame False {
                  }
                  frame True {
                    n174 = call <vilib>:"Build State String with Arguments__jki_lib_state_machine.vi"("Arguments (\"\")"=w280, "State"="detected") -> ("State with Arguments"=w279:string)  [unwired: 4 in]
                    n175 = call <vilib>:"Add State(s) to Queue__jki_lib_state_machine.vi"("State(s) in (\"\")"=w278, "State(s) at Back (\"\")"=w279) -> ("States Out"=w277:string)  [unwired: 13 in]
                  }
                }
              }
              event "stop": Value Change {
                # "Exit Button Value Change (pressed) Event\n(this executes Macro: Exit to terminate the VI)"
                n176 = event-data() -> ()  [unwired: 1 in, 6 out]
                n177 = call <vilib>:"Add State(s) to Queue__jki_lib_state_machine.vi"("State(s) in Front (\"\")"="Macro: Exit", "State(s) in (\"\")"=w300) -> ("States Out"=w299:string)  [unwired: 13 in]
              }
              event Value Change {
                n178 = event-data() -> ()  [unwired: 1 in, 6 out]
                n179 = property on="Set Centriod Target" class="Bool (strict)"("Value"=FALSE) -> ()  [unwired: 2 in, 2 out]
                n180 = Unbundle By Name(w311) -> ("active ccd"=w303:i32, "Centroid X"=w302:dbl[][], "Centroid Y"=w301:dbl[][])
                n181 = Index Array(array=w307, index=w303) -> (element=w306:string)
                n182 = Concatenate Strings("Do want to update the target of " ("message"), w306, "?" ("string")) -> (w304:string)
                n183 = Two Button Dialog(message=w304) -> (T button?=w310:bool)  [unwired: 2 in]
                n184 = case shown="True" w310 {
                  tunnel: w309 -> [_ w322]
                  tunnel: w303 -> [_ w321]
                  tunnel: w302 -> [_ w328]
                  tunnel: w301 -> [_ w323]
                  frame False {
                  }
                  frame True {
                    n185 = Index Array(array=w328, index (row)=w321) -> (element=w327:dbl[])  [unwired: 1 in]
                    n186 = Index Array(array=w323, index (row)=w321) -> (element=w324:dbl[])  [unwired: 1 in]
                    n187 = Index Array(array=w322, index=w321) -> (element=w320:T31)
                    n188 = Unbundle By Name(w320) -> ("Target.X::12"=w319:refnum<vi>, "Target.Y::12"=w317:refnum<vi>)
                    n189 = Reverse 1D Array(array=w327) -> (reversed array=w326:dbl[])
                    n190 = Reverse 1D Array(array=w324) -> (reversed array=w325:dbl[])
                    n191 = Index Array(array=w326) -> (element=w318:dbl)  [unwired: 1 in]
                    n192 = Index Array(array=w325) -> (element=w316:dbl)  [unwired: 1 in]
                    n193 = property class="DigNum (strict)"(reference=w319, "Val(Sgnl)"=w318) -> ()  [unwired: 1 in, 2 out]
                    n194 = property class="DigNum (strict)"(reference=w317, "Val(Sgnl)"=w316) -> ()  [unwired: 1 in, 2 out]
                  }
                }
                n195 = call <vilib>:"Add State(s) to Queue__jki_lib_state_machine.vi"("State(s) in (\"\")"=w315) -> ("States Out"=w314:string)  [unwired: 14 in]
              }
              event "Feedback Global": Value Change {
                # "Exit Button Value Change (pressed) Event\n(this executes Macro: Exit to terminate the VI)"
                n196 = event-data() -> ("NewVal"=w331:bool)  [unwired: 1 in, 5 out]
                n197 = call <vilib>:"Add State(s) to Queue__jki_lib_state_machine.vi"("State(s) in (\"\")"=w334) -> ("States Out"=w333:string)  [unwired: 14 in]
                n198 = Bundle By Name(cluster=w330, "Feedback global"=w331) -> (w329:T37)
              }
              event Value Change {
                n199 = event-data() -> ()  [unwired: 1 in, 6 out]
                n200 = call <vilib>:"Add State(s) to Queue__jki_lib_state_machine.vi"("State(s) in Front (\"\")"="Move Config", "State(s) in (\"\")"=w339) -> ("States Out"=w338:string)  [unwired: 13 in]
              }
              event Value Change {
                n201 = event-data() -> ()  [unwired: 1 in, 6 out]
                n202 = call <vilib>:"Add State(s) to Queue__jki_lib_state_machine.vi"("State(s) in Front (\"\")"="Detection Config", "State(s) in (\"\")"=w344) -> ("States Out"=w343:string)  [unwired: 13 in]
              }
              event "associated motors": Value Change {
                n203 = event-data() -> ()  [unwired: 1 in, 6 out]
                n204 = call <vilib>:"Add State(s) to Queue__jki_lib_state_machine.vi"("State(s) in (\"\")"=w349, "State(s) at Back (\"\")"="Motor Config" ("State(s) at Back (\"\")")) -> ("States Out"=w348:string)  [unwired: 13 in]
              }
              event "Reset History": Value Change {
                n205 = event-data() -> ()  [unwired: 1 in, 6 out]
                n206 = call <vilib>:"Add State(s) to Queue__jki_lib_state_machine.vi"("State(s) in (\"\")"=w355, "State(s) at Back (\"\")"="Reset History" ("State(s) at Back (\"\")")) -> ("States Out"=w354:string)  [unwired: 13 in]
                n207 = property on="Reset History" class="Bool (strict)"("Value"=FALSE ("Reset History")) -> ()  [unwired: 2 in, 2 out]
              }
              event "Save Config": Value Change {
                n208 = event-data() -> ()  [unwired: 1 in, 6 out]
                n209 = call <vilib>:"Add State(s) to Queue__jki_lib_state_machine.vi"("State(s) in (\"\")"=w360, "State(s) at Back (\"\")"="Save Config" ("State(s) at Back (\"\")")) -> ("States Out"=w359:string)  [unwired: 13 in]
              }
              event "Load Config": Value Change {
                n210 = event-data() -> ()  [unwired: 1 in, 6 out]
                n211 = call "File Dialog2"("pattern (all files)"="*.cfg", "pattern label"="config") -> ("selected path"=w364:path)  [unwired: 10 in, 3 out]
                n212 = Path To String(path=w364) -> (string=w362:string)
                "config path" <- w362
                n213 = call <vilib>:"Build State String with Arguments__jki_lib_state_machine.vi"("Arguments (\"\")"=w362, "State"="Load Config" ("State(s) at Back (\"\")")) -> ("State with Arguments"=w361:string)  [unwired: 4 in]
                n214 = call <vilib>:"Add State(s) to Queue__jki_lib_state_machine.vi"("State(s) in (\"\")"=w370, "State(s) at Back (\"\")"=w361) -> ("States Out"=w369:string)  [unwired: 13 in]
              }
              event "Save Stats": Value Change {
                n215 = event-data() -> ()  [unwired: 1 in, 6 out]
                n216 = call <vilib>:"Add State(s) to Queue__jki_lib_state_machine.vi"("State(s) in (\"\")"=w375, "State(s) at Back (\"\")"="Save Stats" ("State(s) at Back (\"\")")) -> ("States Out"=w374:string)  [unwired: 13 in]
              }
              event "active CCDs": Value Change {
                n217 = event-data() -> ("NewVal"=w381:i32)  [unwired: 1 in, 5 out]
                n218 = Unbundle By Name(w377) -> ("active cams"=w376:string[])
                n219 = Index Array(array=w376, index=w381) -> (element=w379:string)
                n220 = call <vilib>:"Build State String with Arguments__jki_lib_state_machine.vi"("Arguments (\"\")"=w379, "State"="active" ("State(s) at Back (\"\")")) -> ("State with Arguments"=w378:string)  [unwired: 4 in]
                n221 = call <vilib>:"Add State(s) to Queue__jki_lib_state_machine.vi"("State(s) in (\"\")"=w384, "State(s) at Back (\"\")"=w378) -> ("States Out"=w383:string)  [unwired: 13 in]
              }
              event "Left", "Right": Value Change {
                n222 = event-data() -> ("CtlRef"=w393:refnum<vi>)  [unwired: 1 in, 5 out]
                n223 = property class="Bool (strict)"(reference=w393, error in=w390) -> (reference out=w392:refnum<vi>, error out=w391:errorcluster, "Label.Text"=w387:string)
                n224 = property class="Bool (strict)"(reference=w392, error in=w391, "Value"=FALSE) -> (error out=w389:errorcluster)  [unwired: 1 out]
                n225 = call <vilib>:"Build State String with Arguments__jki_lib_state_machine.vi"("Arguments (\"\")"=w387, "State"="ManMove X") -> ("State with Arguments"=w386:string)  [unwired: 4 in]
                n226 = call <vilib>:"Add State(s) to Queue__jki_lib_state_machine.vi"("State(s) in (\"\")"=w396, "State(s) at Back (\"\")"=w386) -> ("States Out"=w395:string)  [unwired: 13 in]
              }
              event "Up", "Down": Value Change {
                n227 = event-data() -> ("CtlRef"=w405:refnum<vi>)  [unwired: 1 in, 5 out]
                n228 = property class="Bool (strict)"(reference=w405, error in=w402) -> (reference out=w404:refnum<vi>, error out=w403:errorcluster, "Label.Text"=w399:string)
                n229 = property class="Bool (strict)"(reference=w404, error in=w403, "Value"=FALSE) -> (error out=w401:errorcluster)  [unwired: 1 out]
                n230 = call <vilib>:"Build State String with Arguments__jki_lib_state_machine.vi"("Arguments (\"\")"=w399, "State"="ManMove Y") -> ("State with Arguments"=w398:string)  [unwired: 4 in]
                n231 = call <vilib>:"Add State(s) to Queue__jki_lib_state_machine.vi"("State(s) in (\"\")"=w408, "State(s) at Back (\"\")"=w398) -> ("States Out"=w407:string)  [unwired: 13 in]
              }
              event "Center": Value Change {
                n232 = event-data() -> ()  [unwired: 1 in, 6 out]
                n233 = call <vilib>:"Add State(s) to Queue__jki_lib_state_machine.vi"("State(s) in (\"\")"=w413, "State(s) at Back (\"\")"="Center" ("State(s) at Back (\"\")")) -> ("States Out"=w412:string)  [unwired: 13 in]
              }
              event "new tdms": Value Change {
                n234 = event-data() -> ()  [unwired: 1 in, 6 out]
                n235 = call <vilib>:"Add State(s) to Queue__jki_lib_state_machine.vi"("State(s) in (\"\")"=w418, "State(s) at Back (\"\")"="newtdms" ("State(s) at Back (\"\")")) -> ("States Out"=w417:string)  [unwired: 13 in]
              }
              event "device ini": Value Change {
                n236 = event-data() -> ()  [unwired: 1 in, 6 out]
                n237 = property on="device ini" class="Bool (strict)"("Value"=FALSE ("test")) -> ()  [unwired: 2 in, 2 out]
                n238 = call <vilib>:"Add State(s) to Queue__jki_lib_state_machine.vi"("State(s) in (\"\")"=w424, "State(s) at Back (\"\")"="Device Ini" ("State(s) at Back (\"\")")) -> ("States Out"=w423:string)  [unwired: 13 in]
              }
              event "img to avg": Value Change {
                n239 = event-data() -> ("NewVal"=w430:i32)  [unwired: 1 in, 5 out]
                n240 = Number To Decimal String(number=w430) -> (decimal integer string=w432:string)  [unwired: 1 in]
                n241 = call <vilib>:"Build State String with Arguments__jki_lib_state_machine.vi"("Arguments (\"\")"=w432, "State"="ImgToAvg" ("State(s) at Back (\"\")")) -> ("State with Arguments"=w427:string)  [unwired: 4 in]
                n242 = call <vilib>:"Add State(s) to Queue__jki_lib_state_machine.vi"("State(s) in (\"\")"=w428, "State(s) at Back (\"\")"=w427) -> ("States Out"=w426:string)  [unwired: 13 in]
              }
              event Panel Close? {
                # "Discard the event because we'll close the front panel ourselves in Macro: Exit"
                # "Close Panel button (pressed) Event\n(this executes Macro: Exit to terminate the VI)"
                n243 = event-data() -> ()  [unwired: 1 in, 1 out]
                n244 = call <vilib>:"Add State(s) to Queue__jki_lib_state_machine.vi"("State(s) in Front (\"\")"="Macro: Exit", "State(s) in (\"\")"=w438) -> ("States Out"=w437:string)  [unwired: 13 in]
                n245 = event-data("Discard?"=TRUE) -> ()  [unwired: 1 in, 1 out]
              }
            }
          }
          frame "---------- Core ----------" {
            # "Do not put any code in this frame.\n(it is a separator no-op)"
            n246 = call <vilib>:"Add State(s) to Queue__jki_lib_state_machine.vi"("State(s) in (\"\")"=w442) -> ("States Out"=w441:string)  [unwired: 14 in]
          }
          frame Default {
            w452 = 42 items=["No error", "Argument error", "Memory is full", "Out of zone", "End of file", "File already open", "Generic file I/O error", "File not found", "File permission error", "Disk is full", "Duplicate path", "Too many files open", "System feature not enabled", "Resource file not found", "Cannot add resource", "Resource not found", "Image not found", "Image memory error", "Pen does not exist", "Config type invalid", "Config token not found", "Config parse error", "Config memory error", "Bad external code format", "Bad external code offset", "External code not present", "Null window", "Destroy window error", "Null menu", "Print aborted", "Bad print record", "Print driver error", "Windows error during printing", "Memory error during printing", "Print dialog error", "Generic print error", "Invalid device refnum", "Device not found", "Device parameter error", "Device unit error", "Cannot open device", "Device call aborted", "Generic error", "Cancelled by user", "Object ID too low", "Object ID too high", "Object not in heap", "Unknown heap", "Unknown object (invalid DefProc)", "Unknown object (DefProc not in table)", "Message out of range", "Invalid (null) method", "Unknown message", "Manager call not supported", "Bad address", "Network operation in progress", "Network operation timed out", "Connection is busy", "Network attribute not supported", "Network error", "Address in use", "System out of memory", "Connection aborted", "Connection refused", "Not connected", "Already connected", "Connection closed", "Initialization error (interapplication manager)", "Bad occurrence", "Wait on unbound occurrence handler", "Occurrence queue overflow", "Datalog type conflict", "Unused", "Unrecognized type (interapplication manager)", "Memory corrupt", "Failed to make temporary DLL", "Old CIN version", "Drag socket not found", "Failed to load drop-object", "Failed to register OLE object", "Failed to release OLE object", "Format specifier type mismatch", "Unknown format specifier", "Too few format specifiers", "Too many format specifiers", "Scan failed", "Newer CIN version", "Error converting to variant", "Runtime menu error", "Password tampered", "Variant attribute not found", "Incompatible variant data type", "Event data is not available", "Event Store is not present", "Occurrence is not found", "Event Queue is not created", "Event info is not available", "Refnum passed is NULL", "Error retrieving Class GUID", "Error retrieving CoClass GUID", "Error retrieving TypeLib GUID.", "Bad built application magic bytes.", "Specific driver is different from the specific driver associated with the Logical Name.", "There is no session opened to the class driver.", "Max Error", "MAX - Error with config objects", "MAX - Error loading configuration", "MAX - Group not supported"]
            # "Current State"
            # "Do not delete, rename, or modify this frame.\n(this is used to capture unhandled states and typos)"
            # "Handle mistyped state name (developer tool)"
            n247 = Format Into String(format string="Software Exception: Unhandled State \"%s\"." ("message"), error in=w448, w443) -> (resulting string=w451:string, error out=w450:errorcluster)  [unwired: 1 in]
            n248 = call <vilib>:"Error Cluster From Error Code.vi"("show call chain? (False)"=TRUE, "error in (no error)"=w450, "error message (\"\")"=w451, "error code (0)"=w452) -> ("error out"=w449:errorcluster)  [unwired: 5 in]
            n249 = call <vilib>:"Add State(s) to Queue__jki_lib_state_machine.vi"("State(s) in (\"\")"=w447) -> ("States Out"=w446:string)  [unwired: 14 in]
          }
          frame "Initialize Core Data" {
            # "Do not delete, rename, or modify this frame.\n(this is used to determine panel behavior on exit)"
            # "originally closed?"
            # "exe?"
            # "If panel starts closed or is an EXE, then close it when we exit"
            n250 = property class="VI"() -> ("Front Panel.Open"=w462:bool)  [unwired: 2 in, 2 out]
            n251 = property class="App"() -> ("App.Kind"=w461:T16)  [unwired: 2 in, 2 out]
            n252 = control-ref of="Current VI Reference"() -> (w456:refnum<vi>)
            n253 = Not(x=w462) -> (.not. x?=w459:bool)
            n254 = Equal?(x=w461, y=T16."Run Time System" ("Application:Kind")) -> (x = y?=w458:bool)
            n255 = Or(x=w459, y=w458) -> (x .or. y?=w457:bool)
            n256 = Bundle By Name(cluster=w455, "Core.Current VI Reference"=w456, "Core.Close Panel on Exit?"=w457) -> (w454:T37)
            n257 = call <vilib>:"Add State(s) to Queue__jki_lib_state_machine.vi"("State(s) in (\"\")"=w465) -> ("States Out"=w464:string)  [unwired: 14 in]
          }
          frame "Error Handler" {
            # "Unhandled Error -- Display it"
            # "Handle any errors here.\nYou can also output any states to clean-up after errors occur"
            # "Clear error"
            n258 = call <vilib>:"General Error Handler.vi"("error in (no error)"=w467) -> ()  [unwired: 10 in, 5 out]
            n259 = call <vilib>:"Add State(s) to Queue__jki_lib_state_machine.vi"("State(s) in Front (\"\")"="/* Post Error States", "State(s) in (\"\")"=w471) -> ("States Out"=w470:string)  [unwired: 13 in]
          }
          frame "Exit" {
            # "Do not put any code in this frame.\n(No errors that occur here will be handled.)"
            n260 = call <vilib>:"Add State(s) to Queue__jki_lib_state_machine.vi"("State(s) in (\"\")"=w476) -> ("States Out"=w475:string)  [unwired: 14 in]
          }
          frame "---------- Data ----------" {
            # "Do not put any code in this frame.\n(It is a separator no-op. You can make a copy of this frame to create a new Data frame)"
            n261 = call <vilib>:"Add State(s) to Queue__jki_lib_state_machine.vi"("State(s) in (\"\")"=w480) -> ("States Out"=w479:string)  [unwired: 14 in]
          }
          frame "Data: Initialize" {
            w481 = bool[] [FALSE, FALSE, FALSE, FALSE, TRUE, TRUE, TRUE, FALSE, FALSE, FALSE, FALSE, FALSE]  # detected
            w497 = bool[] [FALSE, FALSE, FALSE, FALSE, FALSE, FALSE, FALSE, FALSE, FALSE, FALSE, FALSE, TRUE]  # speedmode Y
            w498 = bool[] [FALSE, FALSE, FALSE, FALSE, FALSE, FALSE, FALSE, FALSE, FALSE, FALSE, FALSE, TRUE]  # speedmode X
            w500 = cluster{"Lower value":sgl, "Upper value":sgl}[] [{"Lower value"=93.0, "Upper value"=255.0}, {"Lower value"=105.0, "Upper value"=255.0}, {"Lower value"=0.0, "Upper value"=255.0}, {"Lower value"=127.0, "Upper value"=255.0}, {"Lower value"=0.0, "Upper value"=255.0}, {"Lower value"=0.0, "Upper value"=255.0}, {"Lower value"=0.0, "Upper value"=255.0}, {"Lower value"=0.0, "Upper value"=255.0}, {"Lower value"=0.0, "Upper value"=255.0}, {"Lower value"=0.0, "Upper value"=255.0}, {"Lower value"=0.0, "Upper value"=255.0}, {"Lower value"=0.0, "Upper value"=255.0}]  # thresholds
            w507 = FALSE  # Feedback global
            w509 = 0  # active ccd
            w493 = 2  # img to avg
            w520 = T38 {"Current VI Reference"=refnum, "Close Panel on Exit?"=FALSE}  # Core
            # "Initialize the shift-register data, here.\n(data names are defined by what you wire into the bundle function)"
            n262 = TDMS Open(6:FALSE ("disable buffering (T)"), 7:enum16{"1.0", "2.0"}."2.0" ("file format version (2.0)"), 8:w485, 10:T17."create or replace" ("operation"), 11:w483) -> (0:w489:errorcluster, 3:w490:refnum<k34>)  [unwired: 2 in]
            n263 = call "TDMSbuffersize.vi"("error in (no error)"=w489, "Data Value Reference in"=w490) -> ("error out"=w484:errorcluster, "Data Value Reference out"=w482:refnum<k34>)  [unwired: 8 in]
            n264 = call <vilib>:"Add State(s) to Queue__jki_lib_state_machine.vi"("State(s) in (\"\")"=w522) -> ("States Out"=w521:string)  [unwired: 14 in]
            n265 = Bundle("Core"=w520, "detection para"="detection para", "thresholds"=w500, "Centroid X"="Centroid X", "Centroid Y"="Centroid Y", "img to avg"=w493, "Mean Centroid X"="Mean Centroid X", "Mean Centroid Y"="Mean Centroid Y", "Offset X"="Offset X", "Offset Y"="Offset Y", "Offset X stats"="Offset X stats", "Offset Y stats"="Offset Y stats", "Size"="Size", "Mean Size"="Mean Size", "Time"="Time", "move properties"="move properties", "active axis refs 2"="active axis refs 2", "active ccd"=w509, "Feedback global"=w507, "Motor X"="Motor X", "Motor Y"="Motor Y", "active cams"="active cams", "Data Value Reference out"=w482, "active man refs"="active man refs", "detected"=w481, "speedmode X"=w498, "speedmode Y"=w497) -> (w492:T37)  [unwired: 1 in]
            n266 = Initialize Array(0.0 ("element"), 12 ("dimension size"), w493) -> (w496:dbl[][])
            n267 = Bundle By Name(cluster=w492, "Centroid X"=w496, "Centroid Y"=w496, "Size"=w496) -> (w491:T37)
          }
          frame "Data: Cleanup" {
            # "Cleanup any data and references, here.\n(this is called automatically, by the Macro: Exit)"
            n268 = Unbundle By Name(w523) -> ("Core.Current VI Reference"=w524:refnum<vi>)
            n269 = Close Reference(reference=w524, error in (no error)=w526) -> (error out=w525:errorcluster)
            n270 = call <vilib>:"Add State(s) to Queue__jki_lib_state_machine.vi"("State(s) in (\"\")"=w528) -> ("States Out"=w527:string)  [unwired: 14 in]
          }
          frame "---------- UI ----------" {
            # "Do not put any code in this frame.\n(It is a separator no-op. You can make a copy of this frame to create a new UI frame)"
            n271 = call <vilib>:"Add State(s) to Queue__jki_lib_state_machine.vi"("State(s) in (\"\")"=w532) -> ("States Out"=w531:string)  [unwired: 14 in]
          }
          frame "UI: Initialize" {
            # "Initialize the User Interface, here.\n(this is called automatically, by the Macro: Init)"
            n272 = call <vilib>:"Add State(s) to Queue__jki_lib_state_machine.vi"("State(s) in (\"\")"=w536) -> ("States Out"=w535:string)  [unwired: 14 in]
          }
          frame "UI: Cursor Set" {
            # "Argument"
            # "Set and Unset Cursor Busy.\n(Usage: \"UI: Cursor Set >> Busy|Idle\")"
            n273 = case shown="\"Idle\", Default" w537 {
              tunnel: w539 -> [w544 w546]
              tunnel: [w543 w545] -> w538
              frame "Idle", Default {
                n274 = call <vilib>:"Unset Busy.vi"("error in (no error)"=w544) -> ("error out"=w543:errorcluster)  [unwired: 10 in]
              }
              frame "Busy" {
                n275 = call <vilib>:"Set Busy.vi"("error in (no error)"=w546) -> ("error out"=w545:errorcluster)  [unwired: 9 in, 1 out]
              }
            }
            n276 = call <vilib>:"Add State(s) to Queue__jki_lib_state_machine.vi"("State(s) in (\"\")"=w542) -> ("States Out"=w541:string)  [unwired: 14 in]
          }
          frame "UI: Front Panel State" {
            # "Argument"
            # "Set Front Panel Open or Closed\n(Usage: \"UI: Front Panel State >> Open|Close\")"
            n277 = Unbundle By Name(w547) -> ("Core.Current VI Reference"=w549:refnum<vi>)
            n278 = case shown="\"Open\", Default" w548 {
              tunnel: w551 -> [w557 w568]
              tunnel: [w558 w569] -> w550
              tunnel: w549 -> [_ _]
              frame "Open", Default {
                n279 = property class="VI"(error in=w557) -> (reference out=w555:refnum<vi>, error out=w556:errorcluster, "Front Panel.Open"=w554:bool)  [unwired: 1 in]
                n280 = case shown="False" w554 {
                  tunnel: [w561 w564] -> w558
                  tunnel: w556 -> [w560 w564]
                  tunnel: w555 -> [w559 _]
                  frame False {
                    n281 = invoke class="VI" method="FP.Open"(reference=w559, error in=w560, "Activate"=TRUE, "State"=T18."Standard") -> (error out=w561:errorcluster)  [unwired: 1 in, 4 out]
                  }
                  frame True {
                  }
                }
              }
              frame "Close" {
                n282 = property class="VI"(error in=w568) -> (reference out=w566:refnum<vi>, error out=w567:errorcluster, "Front Panel.Open"=w565:bool)  [unwired: 1 in]
                n283 = case shown="True" w565 {
                  tunnel: [w570 w573] -> w569
                  tunnel: w567 -> [w570 w572]
                  tunnel: w566 -> [_ w571]
                  frame False {
                  }
                  frame True {
                    n284 = invoke class="VI" method="FP.Close"(reference=w571, error in=w572) -> (error out=w573:errorcluster)  [unwired: 1 in, 2 out]
                  }
                }
              }
            }
            n285 = call <vilib>:"Add State(s) to Queue__jki_lib_state_machine.vi"("State(s) in (\"\")"=w553) -> ("States Out"=w552:string)  [unwired: 14 in]
          }
          frame "---------- Macro ----------" {
            # "Do not put any code in this frame.\n(It is a separator no-op. You can make a copy of this frame to create a new Macro frame)"
            n286 = call <vilib>:"Add State(s) to Queue__jki_lib_state_machine.vi"("State(s) in (\"\")"=w577) -> ("States Out"=w576:string)  [unwired: 14 in]
          }
          frame "Macro: Initialize" {
            # "Initialization Macro\n(This is called once, when the VI starts)"
            n287 = property on="img to avg" class="DigNum (strict)"() -> ("Value"=w579:i32)  [unwired: 2 in, 2 out]
            n288 = Number To Decimal String(number=w579) -> (decimal integer string=w581:string)  [unwired: 1 in]
            n289 = call <vilib>:"Build State String with Arguments__jki_lib_state_machine.vi"("Arguments (\"\")"=w581, "State"="ImgToAvg") -> ("State with Arguments"=w578:string)  [unwired: 4 in]
            n290 = call <vilib>:"Add State(s) to Queue__jki_lib_state_machine.vi"("State(s) in Front (\"\")"="Data: Initialize\nInitialize Core Data\nUI: Initialize\nUI: Front Panel State >> Open\nDevice Ini >> 3000", "State(s) in (\"\")"=w586, "State(s) at Back (\"\")"=w578) -> ("States Out"=w585:string)  [unwired: 12 in]
          }
          frame "Macro: Exit" {
            # "Exit Macro\n(This is called once, when the VI exits)"
            n291 = Unbundle By Name(w588) -> ("Core.Close Panel on Exit?"=w587:bool)
            n292 = Select(t="UI: Front Panel State >> Close", s=w587, f="") -> (s? t:f=w591:string)
            n293 = call <vilib>:"Add State(s) to Queue__jki_lib_state_machine.vi"("State(s) in (\"\")"=w591, "State(s) at Back (\"\")"="Data: Cleanup\nExit") -> ("States Out"=w589:string)  [unwired: 13 in]
            n294 = call <vilib>:"Add State(s) to Queue__jki_lib_state_machine.vi"("State(s) in Front (\"\")"=w589, "State(s) in (\"\")"=w596) -> ("States Out"=w595:string)  [unwired: 13 in]
          }
          frame "---------- Ini and Configure ----------" {
            # "Template Separator\n(You can make a copy of, or modify, this frame)"
            n295 = call <vilib>:"Add State(s) to Queue__jki_lib_state_machine.vi"("State(s) in (\"\")"=w600) -> ("States Out"=w599:string)  [unwired: 14 in]
          }
          frame "Device Ini" {
            # "Your code here.\n(You can make a copy of, or modify, this frame)"
            n296 = Empty String/Path?(string/path=w617) -> (empty?=w616:bool)
            n297 = case shown="False" w616 {
              tunnel: w617 -> [w658 _]
              tunnel: [w657 0] -> w615
              frame False {
                n298 = Decimal String To Number(string=w658) -> (number=w657:i32)  [unwired: 2 in, 1 out]
              }
              frame True {
              }
            }
            n299 = flat-sequence {
              tunnel: w623 -> [w661]
              tunnel: [w661] -> w622
              tunnel: w615 -> [w660]
              tunnel: w622 -> [w664]
              tunnel: [w662] -> w606
              frame #0 {
                n300 = Wait (ms)(milliseconds to wait=w660) -> ()  [unwired: 1 out]
              }
              frame #1 {
                n301 = for {
                  tunnel: w664 -> [w666] mode=indexing
                  shift-right: [w667] -> w662
                  shift-left: string[] [] -> [w668]
                  n302 = call "send command.vi"("Device Name"=w666) -> ("status"=w669:bool)  [unwired: 4 in]
                  n303 = Wait (ms)(milliseconds to wait=u32 5) -> ()  [unwired: 1 out]
                  n304 = case shown="True" w669 {
                    tunnel: w668 -> [w670 w673]
                    tunnel: [w670 w672] -> w667
                    tunnel: w666 -> [_ w671]
                    frame False {
                    }
                    frame True {
                      n305 = Build Array (concatenate)(w673, w671) -> (w672:string[])
                    }
                  }
                }
              }
            }
            n306 = Unbundle By Name(w614) -> ("active cams"=w607:string[])
            n307 = call <vilib>:"Add State(s) to Queue__jki_lib_state_machine.vi"("State(s) in (\"\")"=w624) -> ("States Out"=w609:string)  [unwired: 14 in]
            n308 = Equal?(x=w607, y=w606) -> (x = y?=w613:bool[])
            n309 = Empty Array?(array=w607) -> (empty?=w612:bool)
            n310 = Not(x=w612) -> (.not. x?=w611:bool)
            n311 = Build Array (concatenate)(w613, w611) -> (w610:bool[])
            n312 = Array Size(array=w606) -> (size(s)=w605:i32)
            n313 = Array Size(array=w607) -> (size(s)=w604:i32)
            n314 = And Array Elements(Boolean array=w610) -> (logical AND=w602:bool)
            n315 = Equal?(x=w605, y=w604) -> (x = y?=w603:bool)
            n316 = And(x=w603, y=w602) -> (x .and. y?=w601:bool)
            n317 = case shown="False" w601 {
              tunnel: [w639 w656] -> w621
              tunnel: w620 -> [_ _]
              tunnel: w619 -> [w636 w655]
              tunnel: [w636 w655] -> w618
              tunnel: w614 -> [w632 w656]
              tunnel: w606 -> [w633 _]
              tunnel: w609 -> [w638 w654]
              tunnel: [w626 w654] -> w608
              frame False {
                n318 = property on="active CCDs" class="LstBox (strict)"("Item Names"=w633) -> ()  [unwired: 2 in, 2 out]
                n319 = Array Size(array=w633) -> (size(s)=w646:i32)
                n320 = Initialize Array(0.0 ("element"), w646, 0 ("dimension size")) -> (w641:dbl[][])
                n321 = Unbundle By Name(w632) -> ("img to avg"=w631:i32)
                n322 = Bundle By Name(cluster=w632, "active cams"=w633) -> (w640:T37)
                n323 = Initialize Array(0.0 ("element"), 12 ("dimension size"), w631) -> (w630:dbl[][])
                n324 = Bundle By Name(cluster=w640, "Offset X stats"=w641, "Offset Y stats"=w641, "Centroid X"=w630, "Centroid Y"=w630, "Mean Centroid X"=w641, "Mean Centroid Y"=w641, "Offset X"=w641, "Offset Y"=w641, "Size"=w630, "Mean Size"=w641, "Motor X"=w641, "Motor Y"=w641) -> (w639:T37)
                n325 = for {
                  N: 1 -> [_]
                  shift-right: [w648] -> w644
                  shift-left: timestamp[][] [] ("Time") -> [w650]
                  n326 = for {
                    N: 12 -> [_]
                    tunnel: w650 -> [w653] mode=indexing
                    tunnel: [w651] -> w648 mode=indexing
                    n327 = Get Date/Time In Seconds() -> (seconds since 1Jan1904=w652:timestamp)
                    n328 = Build Array (concatenate)(w653, w652) -> (w651:timestamp[])
                  }
                }
                n329 = property on="config path" class="Str"() -> ("Value"=w628:string)  [unwired: 2 in, 2 out]
                n330 = call <vilib>:"Add State(s) to Queue__jki_lib_state_machine.vi"("State(s) in Front (\"\")"="newtdms\nMove Config\nMotor Config\nDetection Config\nactive\nCenter" ("State(s) in Front (\"\")"), "State(s) in (\"\")"=w638) -> ("States Out"=w627:string)  [unwired: 13 in]
                n331 = call <vilib>:"Build State String with Arguments__jki_lib_state_machine.vi"("Arguments (\"\")"=w628, "State"="Load Config" ("State(s) in Front (\"\")")) -> ("State with Arguments"=w625:string)  [unwired: 4 in]
                n332 = call <vilib>:"Add State(s) to Queue__jki_lib_state_machine.vi"("State(s) in (\"\")"=w627, "State(s) at Back (\"\")"=w625) -> ("States Out"=w626:string)  [unwired: 13 in]
                n333 = property on="Time" class="Arr (strict)"("Value"=w644) -> ()  [unwired: 2 in, 2 out]
                "name array" <- w633
              }
              frame True {
              }
            }
          }
          frame "Load Config" {
            # "Your code here.\n(You can make a copy of, or modify, this frame)"
            n334 = Unbundle By Name(w715) -> ("detection para"=w721:T3[], "move properties"=w718:T2[], "thresholds"=w711:cluster{"Lower value":sgl, "Upper value":sgl}[])
            n335 = Empty String/Path?(string/path=w678) -> (empty?=w677:bool)
            n336 = case shown="False" w677 {
              tunnel: [w731 T5 {"CCDs"=[], "move properties"=[], "detection para"=[], "thresholds"=[], "Value"={"Motor CCD 1"=0, "Motor CCD 2"=0, "Motor CCD 3"=0, "Motor CCD 4"=0, "Motor CCD 5"=0, "Motor CCD 6"=0, "Motor CCD 7"=0, "Motor CCD 8"=0, "Motor CCD 9"=0, "Motor CCD 10"=0, "Motor CCD 11"=0, "Motor CCD 12"=0}} ("output cluster 2")] -> w723
              tunnel: [w729 w738] -> w682
              tunnel: w679 -> [w728 w738]
              tunnel: w678 -> [w727 _]
              frame False {
                n337 = String To Path(string=w727) -> (path=w726:path)
                n338 = Open/Create/Replace File(file path (use dialog)=w726, error in=w728, operation (0:open)=T19."open or create") -> (refnum out=w733:refnum<file>, error out=w734:errorcluster)  [unwired: 3 in, 1 out]
                n339 = Read from Binary File(5:"output cluster 2", 8:w734, 11:w733) -> (0:w735:errorcluster, 2:w731:T5, 3:w736:refnum<file>)  [unwired: 3 in, 1 out]
                n340 = Close File(refnum=w736, error in=w735) -> (error out=w729:errorcluster)  [unwired: 1 out]
              }
              frame True {
              }
            }
            n341 = property on="Load Config" class="Bool (strict)"("Value"=FALSE ("Load Config")) -> ()  [unwired: 2 in, 2 out]
            n342 = Unbundle By Name(w723) -> ("Value"=w709:T7, "CCDs"=w722:string[], "detection para"=w720:T3[], "move properties"=w719:T2[], "thresholds"=w712:cluster{"Lower value":sgl, "Upper value":sgl}[])
            n343 = Cluster To Array(cluster=w709) -> (array=w710:u16[])
            n344 = call <vilib>:"Add State(s) to Queue__jki_lib_state_machine.vi"("State(s) in (\"\")"=w725, "State(s) at Back (\"\")"="Motor Config" ("State(s) at Back (\"\")")) -> ("States Out"=w724:string)  [unwired: 13 in]
            n345 = for {
              tunnel: w722 -> [w754]
              tunnel: w720 -> [w756]
              tunnel: w719 -> [w755]
              shift-right: [w748] -> w717
              shift-left: w721 -> [w753]
              shift-right: [w746] -> w716
              shift-left: w718 -> [w752]
              tunnel: w713 -> [w751] mode=indexing
              tunnel: w712 -> [w747]
              shift-right: [w743] -> w675
              shift-left: w711 -> [w745]
              tunnel: w710 -> [w742]
              tunnel: [w739] -> w708 mode=indexing
              i -> [w740]
              n346 = call-poly <userlib>:"Filter 1D Array__ogtk.vi"("items to filter"=w751, "array"=w754) -> ("filtered item indices"=w757:i32[])  [unwired: 4 in, 1 out]
              n347 = Index Array(array=w757) -> (element=w741:i32)  [unwired: 1 in]
              n348 = Index Array(array=w742, index=w741) -> (element=w739:u16)
              n349 = Index Array(array=w756, index=w741) -> (element=w750:T3)
              n350 = Index Array(array=w755, index=w741) -> (element=w749:T2)
              n351 = Index Array(array=w747, index=w741) -> (element=w744:cluster{"Lower value":sgl, "Upper value":sgl})
              n352 = Replace Array Subset(array=w753, new element=w750, index=w740) -> (w748:T3[])
              n353 = Replace Array Subset(array=w752, new element=w749, index=w740) -> (w746:T2[])
              n354 = Replace Array Subset(array=w745, new element=w744, index=w740) -> (w743:cluster{"Lower value":sgl, "Upper value":sgl}[])
            }
            n355 = Array Size(array=w675) -> (size(s)=→"size(s) 6":i32)
            n356 = Index Array(array=w708, index #1=0 ("index (row)"), index #2=1 ("index (row)"), index #3=2 ("index (row)"), index #4=3 ("index (row)"), index #5=4 ("index (row)"), index #6=5 ("index (row)"), index #7=6 ("index (row)"), index #8=7 ("index (row)"), index #9=8 ("index (row)"), index #10=9 ("index (row)"), index #11=10 ("index (row)"), index #12=11 ("index (row)")) -> (element #1=w695:u16, element #2=w694:u16, element #3=w693:u16, element #4=w692:u16, element #5=w691:u16, element #6=w690:u16, element #7=w689:u16, element #8=w688:u16, element #9=w687:u16, element #10=w686:u16, element #11=w685:u16, element #12=w684:u16)
            n357 = Bundle By Name(cluster=w709, "Motor CCD 1"=w695, "Motor CCD 2"=w694, "Motor CCD 3"=w693, "Motor CCD 4"=w692, "Motor CCD 5"=w691, "Motor CCD 6"=w690, "Motor CCD 7"=w689, "Motor CCD 8"=w688, "Motor CCD 9"=w687, "Motor CCD 10"=w686, "Motor CCD 11"=w685, "Motor CCD 12"=w684) -> (w683:T7)
            n358 = Bundle By Name(cluster=w715, "detection para"=w717, "move properties"=w716, "thresholds"=w675) -> (w714:T37)
            n359 = property on="associated motors" class="Clust (strict)"(error in=w682, "Val(Sgnl)"=w683) -> (error out=w681:errorcluster)  [unwired: 1 in, 1 out]
          }
          frame "Save Config" {
            # "Your code here.\n(You can make a copy of, or modify, this frame)"
            n360 = Unbundle By Name(w775) -> ("move properties"=w761:T2[], "detection para"=w770:T3[], "thresholds"=w758:cluster{"Lower value":sgl, "Upper value":sgl}[])
            n361 = property on="associated motors" class="Clust (strict)"() -> ("Value"=w769:T7)  [unwired: 2 in, 2 out]
            n362 = property on="Save Config" class="Bool (strict)"("Value"=FALSE ("Save Config")) -> ()  [unwired: 2 in, 2 out]
            n363 = local read "CCDs"() -> (w759:string[])
            n364 = call "File Dialog"("pattern (all files)"="*.cfg", "pattern label"="config") -> ("selected path"=w763:path)  [unwired: 10 in, 3 out]
            n365 = Bundle("CCDs"=w759, "move properties"=w761, "detection para"=w770, "thresholds"=w758, "Value"=w769) -> (w762:T5)  [unwired: 1 in]
            n366 = Open/Create/Replace File(file path (use dialog)=w763, error in=w767, operation (0:open)=T19."replace or create with confirmation") -> (refnum out=w771:refnum<file>, error out=w772:errorcluster)  [unwired: 3 in, 1 out]
            n367 = Write to Binary File(file (use dialog)=w771, data=w762, error in=w772) -> (refnum out=w774:refnum<file>, error out=w773:errorcluster)  [unwired: 3 in, 1 out]
            n368 = Close File(refnum=w774, error in=w773) -> (error out=w766:errorcluster)  [unwired: 1 out]
            n369 = call <vilib>:"Add State(s) to Queue__jki_lib_state_machine.vi"("State(s) in (\"\")"=w777) -> ("States Out"=w776:string)  [unwired: 14 in]
          }
          frame "active" {
            # "Your code here.\n(You can make a copy of, or modify, this frame)"
            n370 = Empty String/Path?(string/path=w792) -> (empty?=w791:bool)
            n371 = Unbundle By Name(w788) -> ("move properties"=w804:T2[], "detection para"=w800:T3[])  [unwired: 1 out]
            n372 = Unbundle By Name(w788) -> ("active axis refs 2"=w787:T12)
            n373 = call-poly <userlib>:"Filter 1D Array__ogtk.vi"("items to filter"=w792, "array"=w802) -> ("filtered item indices"=w805:i32[])  [unwired: 4 in, 1 out]
            n374 = Index Array(array=w805) -> (element=w789:i32)  [unwired: 1 in]
            n375 = Select(t=0, s=w791, f=w789) -> (s? t:f=w785:i32)
            n376 = Index Array(array=w787, index=w785) -> (element=w786:cluster{"Ref X":refnum<vi>, "Ref Y":refnum<vi>})
            n377 = Unbundle By Name(w786) -> ("Ref X"=w784:refnum<vi>, "Ref Y"=w783:refnum<vi>)
            n378 = Index Array(array=w804, index=w785) -> (element=w803:T2)
            n379 = Index Array(array=w800, index=w785) -> (element=w799:T3)
            n380 = property on="move config" class="Clust (strict)"(error in=w795, "Value"=w803) -> (error out=w793:errorcluster)  [unwired: 1 in, 1 out]
            n381 = property on="beam detection para" class="Clust (strict)"(error in=w793, "Value"=w799) -> (error out=w794:errorcluster)  [unwired: 1 in, 1 out]
            n382 = call <vilib>:"Add State(s) to Queue__jki_lib_state_machine.vi"("State(s) in (\"\")"=w807) -> ("States Out"=w806:string)  [unwired: 14 in]
            n383 = property class="DigNum (strict)"(reference=w784, error in=w794) -> (error out=w780:errorcluster, "Value"=w782:dbl)  [unwired: 1 out]
            n384 = Bundle By Name(cluster="active Axis ref 3", "Ref X"=w784, "Ref Y"=w783) -> (w797:cluster{"Ref X":refnum<vi>, "Ref Y":refnum<vi>})
            n385 = Bundle By Name(cluster=w788, "active ccd"=w785, "active man refs"=w797) -> (w801:T37)
            n386 = property on="Position 1" class="DigNum (strict)"(error in=w780, "Value"=w782) -> (error out=w779:errorcluster)  [unwired: 1 in, 1 out]
            n387 = property class="DigNum (strict)"(reference=w783, error in=w779) -> (error out=w778:errorcluster, "Value"=w781:dbl)  [unwired: 1 out]
            n388 = property on="Position 2" class="DigNum (strict)"(error in=w778, "Value"=w781) -> (error out=w796:errorcluster)  [unwired: 1 in, 1 out]
          }
          frame "Detection Config" {
            # "Your code here.\n(You can make a copy of, or modify, this frame)"
            n389 = Unbundle By Name(w812) -> ("detection para"=w808:T3[], "active ccd"=w813:i32)
            n390 = Replace Array Subset(array=w808, new element="beam detection para", index=w813) -> (w809:T3[])
            n391 = Bundle By Name(cluster=w812, "detection para"=w809) -> (w811:T37)
            n392 = call <vilib>:"Add State(s) to Queue__jki_lib_state_machine.vi"("State(s) in (\"\")"=w816) -> ("States Out"=w815:string)  [unwired: 14 in]
          }
          frame "Motor Config" {
            # "Your code here.\n(You can make a copy of, or modify, this frame)"
            n393 = Unbundle By Name("associated motors") -> ("Motor CCD 1"=w833:u16, "Motor CCD 2"=w834:u16, "Motor CCD 3"=w835:u16, "Motor CCD 4"=w828:u16, "Motor CCD 5"=w827:u16, "Motor CCD 6"=w826:u16, "Motor CCD 7"=w825:u16, "Motor CCD 8"=w824:u16, "Motor CCD 9"=w823:u16, "Motor CCD 10"=w822:u16, "Motor CCD 11"=w821:u16, "Motor CCD 12"=w820:u16)
            n394 = Build Array(w833, w834, w835, w828, w827, w826, w825, w824, w823, w822, w821, w820) -> (w819:u16[])
            n395 = local read "motor refs"() -> (w831:refnum<vi>[])
            n396 = Increment(x=w819) -> (x+1=w818:u16[])
            n397 = for {
              tunnel: w818 -> [w850] mode=indexing
              tunnel: w831 -> [w845]
              tunnel: [w839] -> w817 mode=indexing
              n398 = Multiply(x=w850, y=u16 2) -> (x*y=w846:u16)
              n399 = Subtract(x=w846, y=u16 2) -> (x-y=w844:u16)
              n400 = Subtract(x=w846, y=u16 1) -> (x-y=w843:u16)
              n401 = Index Array(array=w845, index=w844) -> (element=w842:refnum<vi>)
              n402 = Index Array(array=w845, index=w843) -> (element=w841:refnum<vi>)
              n403 = Bundle By Name(cluster="active Axis ref", "Ref X"=w842, "Ref Y"=w841) -> (w839:cluster{"Ref X":refnum<vi>, "Ref Y":refnum<vi>})
            }
            n404 = call <vilib>:"Add State(s) to Queue__jki_lib_state_machine.vi"("State(s) in (\"\")"=w838) -> ("States Out"=w837:string)  [unwired: 14 in]
            n405 = Bundle By Name(cluster=w830, "active axis refs 2"=w817) -> (w829:T37)
          }
          frame "Move Config" {
            # "Your code here.\n(You can make a copy of, or modify, this frame)"
            n406 = Unbundle By Name(w852) -> ("move properties"=w856:T2[], "active ccd"=w855:i32)
            n407 = Replace Array Subset(array=w856, new element="move config", index=w855) -> (w853:T2[])
            n408 = Bundle By Name(cluster=w852, "move properties"=w853) -> (w851:T37)
            n409 = call <vilib>:"Add State(s) to Queue__jki_lib_state_machine.vi"("State(s) in (\"\")"=w859) -> ("States Out"=w858:string)  [unwired: 14 in]
          }
          frame "----------Centroid & Move----------" {
            # "Template Separator\n(You can make a copy of, or modify, this frame)"
            n410 = call <vilib>:"Add State(s) to Queue__jki_lib_state_machine.vi"("State(s) in (\"\")"=w863) -> ("States Out"=w862:string)  [unwired: 14 in]
          }
          frame "detected" {
            n411 = Unbundle By Name(w868) -> ("Offset X"=w903:dbl[][], "Offset Y"=w902:dbl[][], "Size"=w901:dbl[][], "Mean Size"=w900:dbl[][], "Time"=w897:timestamp[][], "Motor X"=w877:dbl[][], "active axis refs 2"=w876:T12, "Motor Y"=w875:dbl[][])
            n412 = Spreadsheet String To Array(format string="%s", spreadsheet string=w880, array type (2D Dbl)=string[] []) -> (array=w871:string[])  [unwired: 1 in]
            n413 = for {
              tunnel: w872 -> [w917] mode=indexing
              tunnel: w871 -> [w916]
              tunnel: [w915] -> w870 mode=indexing
              n414 = for {
                tunnel: w917 -> [w920]
                tunnel: [w919] -> w914 mode=indexing
                tunnel: w916 -> [w918] mode=indexing
                n415 = Equal?(x=w920, y=w918) -> (x = y?=w919:bool)
              }
              n416 = Or Array Elements(Boolean array=w914) -> (logical OR=w915:bool)
            }
            n417 = Unbundle By Name(w868) -> ("Mean Centroid X"=w908:dbl[][], "Mean Centroid Y"=w907:dbl[][], "Centroid X"=w910:dbl[][], "Centroid Y"=w909:dbl[][])
            n418 = call <vilib>:"Build State String with Arguments__jki_lib_state_machine.vi"("Arguments (\"\")"=w880, "State"="stats") -> ("State with Arguments"=w881:string)  [unwired: 4 in]
            n419 = call <vilib>:"Add State(s) to Queue__jki_lib_state_machine.vi"("State(s) in Front (\"\")"=w881, "State(s) in (\"\")"=w879) -> ("States Out"=w878:string)  [unwired: 13 in]
            n420 = for {
              tunnel: w910 -> [w970]
              tunnel: w909 -> [w969]
              tunnel: w908 -> [w968]
              tunnel: w907 -> [w967]
              tunnel: [w966] -> w894 mode=indexing
              tunnel: [w965] -> w905 mode=indexing
              tunnel: w904 -> [w964] mode=indexing
              tunnel: w903 -> [w963]
              tunnel: w902 -> [w962]
              tunnel: [w961] -> w869 mode=indexing
              tunnel: [w960] -> w895 mode=indexing
              tunnel: w901 -> [w959]
              tunnel: w900 -> [w958]
              tunnel: [w957] -> w899 mode=indexing
              tunnel: w897 -> [w956]
              tunnel: [w955] -> w896 mode=indexing
              tunnel: w877 -> [w947]
              tunnel: w876 -> [w946]
              tunnel: w875 -> [w945]
              tunnel: [w925] -> w874 mode=indexing
              tunnel: [w924] -> w873 mode=indexing
              tunnel: w870 -> [w923]
              i -> [w922]
              n421 = Unbundle By Name(w964) -> ("Target.X::12"=w929:refnum<vi>, "Target.Y::12"=w928:refnum<vi>)
              n422 = Index Array(array=w947, index (row)=w922) -> (element=w950:dbl[])  [unwired: 1 in]
              n423 = Index Array(array=w946, index=w922) -> (element=w949:cluster{"Ref X":refnum<vi>, "Ref Y":refnum<vi>})
              n424 = Index Array(array=w945, index (row)=w922) -> (element=w954:dbl[])  [unwired: 1 in]
              n425 = Index Array(array=w923, index=w922) -> (element=w921:bool)
              n426 = Index Array(array=w968, index (row)=w922) -> (element=w941:dbl[])  [unwired: 1 in]
              n427 = Index Array(array=w967, index (row)=w922) -> (element=w942:dbl[])  [unwired: 1 in]
              n428 = Index Array(array=w970, index (row)=w922) -> (element=w944:dbl[])  [unwired: 1 in]
              n429 = Index Array(array=w969, index (row)=w922) -> (element=w943:dbl[])  [unwired: 1 in]
              n430 = Index Array(array=w963, index (row)=w922) -> (element=w937:dbl[])  [unwired: 1 in]
              n431 = Index Array(array=w962, index (row)=w922) -> (element=w936:dbl[])  [unwired: 1 in]
              n432 = Index Array(array=w959, index (row)=w922) -> (element=w934:dbl[])  [unwired: 1 in]
              n433 = Index Array(array=w958, index (row)=w922) -> (element=w933:dbl[])  [unwired: 1 in]
              n434 = Index Array(array=w956, index (row)=w922) -> (element=w930:timestamp[])  [unwired: 1 in]
              n435 = Unbundle By Name(w949) -> ("Ref X"=w948:refnum<vi>, "Ref Y"=w952:refnum<vi>)
              n436 = property class="DigNum (strict)"(reference=w929) -> ("Value"=w927:dbl)  [unwired: 1 in, 2 out]
              n437 = property class="DigNum (strict)"(reference=w928) -> ("Value"=w926:dbl)  [unwired: 1 in, 2 out]
              n438 = call <vilib>:"Std Deviation and Variance.vi"("X"=w944) -> ("mean"=w940:dbl)  [unwired: 1 in, 2 out]
              n439 = call <vilib>:"Std Deviation and Variance.vi"("X"=w943) -> ("mean"=w939:dbl)  [unwired: 1 in, 2 out]
              n440 = call <vilib>:"Std Deviation and Variance.vi"("X"=w934) -> ("mean"=w932:dbl)  [unwired: 1 in, 2 out]
              n441 = Get Date/Time In Seconds() -> (seconds since 1Jan1904=w931:timestamp)
              n442 = property class="DigNum (strict)"(reference=w948) -> ("Value"=w951:dbl)  [unwired: 1 in, 2 out]
              n443 = property class="DigNum (strict)"(reference=w952) -> ("Value"=w953:dbl)  [unwired: 1 in, 2 out]
              n444 = Subtract(x=w927, y=w940) -> (x-y=w938:dbl)
              n445 = Subtract(x=w926, y=w939) -> (x-y=w935:dbl)
              n446 = case shown="True" w921 {
                tunnel: [w983 w1002] -> w966
                tunnel: [w971 w1001] -> w965
                tunnel: [w972 w1000] -> w961
                tunnel: [w973 w999] -> w960
                tunnel: [w974 w998] -> w957
                tunnel: [w975 w997] -> w955
                tunnel: w942 -> [w981 w996]
                tunnel: w941 -> [w982 w995]
                tunnel: w940 -> [_ w994]
                tunnel: w939 -> [_ w993]
                tunnel: w938 -> [_ w992]
                tunnel: w937 -> [w980 w991]
                tunnel: w936 -> [w979 w990]
                tunnel: w935 -> [_ w989]
                tunnel: w933 -> [w978 w988]
                tunnel: w932 -> [_ w987]
                tunnel: w931 -> [w976 w986]
                tunnel: w930 -> [w977 w985]
                frame False {
                  w984 = 0.0
                  n447 = Build Array (concatenate)(w982, w984) -> (w983:dbl[])
                  n448 = Build Array (concatenate)(w981, w984) -> (w971:dbl[])
                  n449 = Build Array (concatenate)(w980, w984) -> (w972:dbl[])
                  n450 = Build Array (concatenate)(w979, w984) -> (w973:dbl[])
                  n451 = Build Array (concatenate)(w978, w984) -> (w974:dbl[])
                  n452 = Build Array (concatenate)(w977, w976) -> (w975:timestamp[])
                }
                frame True {
                  n453 = Build Array (concatenate)(w995, w994) -> (w1002:dbl[])
                  n454 = Build Array (concatenate)(w996, w993) -> (w1001:dbl[])
                  n455 = Build Array (concatenate)(w991, w992) -> (w1000:dbl[])
                  n456 = Build Array (concatenate)(w990, w989) -> (w999:dbl[])
                  n457 = Build Array (concatenate)(w988, w987) -> (w998:dbl[])
                  n458 = Build Array (concatenate)(w985, w986) -> (w997:timestamp[])
                }
              }
              n459 = Build Array (concatenate)(w950, w951) -> (w925:dbl[])
              n460 = Build Array (concatenate)(w954, w953) -> (w924:dbl[])
            }
            n461 = local write "Numeric"(0.0 ("Numeric")) -> ()
            n462 = Array Size(array=w869) -> (size(s)=w893:i32[])
            n463 = Index Array(array=w893, index=1) -> (element=w891:i32)
            "History Index" <- w891
            n464 = call <vilib>:"Add State(s) to Queue__jki_lib_state_machine.vi"("State(s) in (\"\")"=w878, "State(s) at Back (\"\")"="Check Move\ntdms" ("State(s) at Back (\"\")")) -> ("States Out"=w885:string)  [unwired: 13 in]
            n465 = Unbundle By Name(w868) -> ("img to avg"=w865:i32)
            n466 = Initialize Array(0.0 ("element"), 12 ("dimension size"), w865) -> (w864:dbl[][])
            n467 = Greater?(x=w891, y="History Size") -> (0:w889:bool)
            n468 = Bundle By Name(cluster=w868, "Centroid X"=w864, "Centroid Y"=w864, "Mean Centroid X"=w894, "Mean Centroid Y"=w905, "Offset X"=w869, "Offset Y"=w895, "Mean Size"=w899, "Size"=w864, "Time"=w896, "Motor X"=w874, "Motor Y"=w873) -> (w906:T37)
            n469 = Select(t="history" ("State(s) at Back (\"\")"), s=w889, f="") -> (s? t:f=w886:string)
            n470 = call <vilib>:"Add State(s) to Queue__jki_lib_state_machine.vi"("State(s) in (\"\")"=w885, "State(s) at Back (\"\")"=w886) -> ("States Out"=w884:string)  [unwired: 13 in]
          }
          frame "Check Move" {
            (unwired) "Device Ini" ("State(s) in Front (\"\")")
            n471 = Unbundle By Name(w1005) -> ("move properties"=w1017:T2[], "Mean Size"=w1016:dbl[][], "move properties"=w1015:T2[], "Offset X"=w1014:dbl[][], "Offset Y"=w1013:dbl[][], "active cams"=w1012:string[])
            n472 = for {
              tunnel: w1015 -> [w1045]
              tunnel: w1014 -> [w1043]
              tunnel: w1013 -> [w1041]
              tunnel: w1016 -> [w1049]
              tunnel: [w1065] -> w1011 mode=indexing
              tunnel: [w1061] -> w1010 mode=indexing
              tunnel: w1012 -> [w1050] mode=indexing
              tunnel: [w1083] -> w1018 mode=indexing
              tunnel: [w1082] -> w1008 mode=indexing
              tunnel: w1017 -> [w1048]
              tunnel: [w1059] -> w1007 mode=indexing
              tunnel: [w1054] -> w1006 mode=indexing
              tunnel: "Speedmode @" -> [w1053]
              tunnel: w1003 -> [w1051]
              n473 = call-poly <userlib>:"Filter 1D Array__ogtk.vi"("items to filter"=w1050, "array"=w1051) -> ("filtered item indices"=w1052:i32[])  [unwired: 4 in, 1 out]
              n474 = Index Array(array=w1052) -> (element=w1039:i32)  [unwired: 1 in]
              n475 = Index Array(array=w1048, index=w1039) -> (element=w1047:T2)
              n476 = Index Array(array=w1049, index (row)=w1039) -> (element=w1046:dbl[])  [unwired: 1 in]
              n477 = Index Array(array=w1045, index=w1039) -> (element=w1044:T2)
              n478 = Index Array(array=w1043, index (row)=w1039) -> (element=w1042:dbl[])  [unwired: 1 in]
              n479 = Index Array(array=w1041, index (row)=w1039) -> (element=w1040:dbl[])  [unwired: 1 in]
              n480 = Unbundle By Name(w1044) -> ("Tolerance [%]"=w1076:dbl)
              n481 = Reverse 1D Array(array=w1042) -> (reversed array=w1081:dbl[])
              n482 = Reverse 1D Array(array=w1040) -> (reversed array=w1080:dbl[])
              n483 = Reverse 1D Array(array=w1046) -> (reversed array=w1075:dbl[])
              n484 = Unbundle By Name(w1047) -> ("enable feedback"=w1064:bool)
              n485 = Index Array(array=w1081) -> (element=w1079:dbl)  [unwired: 1 in]
              n486 = Index Array(array=w1080) -> (element=w1078:dbl)  [unwired: 1 in]
              n487 = Index Array(array=w1075) -> (element=w1074:dbl)  [unwired: 1 in]
              n488 = Absolute Value(x=w1079) -> (abs(x)=w1060:dbl)
              n489 = Absolute Value(x=w1078) -> (abs(x)=w1057:dbl)
              n490 = Square Root(x=w1074) -> (sqrt(x)=w1073:dbl)
              n491 = Divide(x=w1076, y=100.0) -> (x/y=w1072:dbl)
              n492 = Multiply(x=w1073, y=w1072) -> (x*y=w1056:dbl)
              n493 = Not Equal To 0?(x=w1057) -> (x != 0?=w1062:bool)
              n494 = Not Equal To 0?(x=w1060) -> (x != 0?=w1067:bool)
              n495 = Greater Or Equal?(x=w1060, y=w1056) -> (x >= y?=w1066:bool)
              n496 = Greater Or Equal?(x=w1057, y=w1056) -> (x >= y?=w1063:bool)
              n497 = Divide(x=w1060, y=w1056) -> (x/y=w1058:dbl)
              n498 = Divide(x=w1057, y=w1056) -> (x/y=w1055:dbl)
              n499 = Compound Arithmetic op=AND(w1064, w1067, w1066) -> (w1065:bool)
              n500 = Compound Arithmetic op=AND(w1064, w1063, w1062) -> (w1061:bool)
              n501 = Boolean To (0,1)(Boolean=w1061) -> (0, 1=w1068:i16)
              n502 = Greater?(x=w1058, y=w1053) -> (0:w1059:bool)
              n503 = Greater?(x=w1055, y=w1053) -> (0:w1054:bool)
              n504 = Multiply(x=w1068, y=w1057) -> (x*y=w1069:dbl)
              n505 = Boolean To (0,1)(Boolean=w1065) -> (0, 1=w1071:i16)
              n506 = Multiply(x=w1071, y=w1060) -> (x*y=w1070:dbl)
              n507 = Bundle(w1069, "GUIdevice 8"=w1050) -> (w1082:cluster{dbl, "GUIdevice 8":string})  [unwired: 1 in]
              n508 = Bundle(w1070, "GUIdevice 8"=w1050) -> (w1083:cluster{dbl, "GUIdevice 8":string})  [unwired: 1 in]
            }
            "required X" <- w1011
            "required Y" <- w1010
            "speedmode X" <- w1007
            "speedmode Y" <- w1006
            n509 = case shown="True" "Align" {
              tunnel: w1018 -> [w1089 w1094]
              tunnel: w1008 -> [w1088 w1091]
              tunnel: [w1087 w1093] -> w1021
              tunnel: [w1086 w1090] -> w1020
              frame False {
                n510 = Sort 1D Array(array=w1088) -> (sorted array=w1085:cluster{dbl, "GUIdevice 8":string}[])
                n511 = Sort 1D Array(array=w1089) -> (sorted array=w1084:cluster{dbl, "GUIdevice 8":string}[])
                n512 = Reverse 1D Array(array=w1085) -> (reversed array=w1086:cluster{dbl, "GUIdevice 8":string}[])
                n513 = Reverse 1D Array(array=w1084) -> (reversed array=w1087:cluster{dbl, "GUIdevice 8":string}[])
              }
              frame True {
                w1092 = cluster{dbl, "GUIdevice 8":string}[] [] ("Array")
                n514 = for {
                  shift-right: [w1104] -> w1093
                  shift-left: w1092 -> [w1106]
                  tunnel: w1094 -> [w1105] mode=indexing
                  n515 = Unbundle(w1105) -> (w1108:dbl)  [unwired: 1 out]
                  n516 = Not Equal To 0?(x=w1108) -> (x != 0?=w1107:bool)
                  n517 = case shown="True" w1107 {
                    tunnel: w1106 -> [w1109 w1112]
                    tunnel: w1105 -> [_ w1111]
                    tunnel: [w1109 w1110] -> w1104
                    frame False {
                    }
                    frame True {
                      n518 = Build Array (concatenate)(w1112, w1111) -> (w1110:cluster{dbl, "GUIdevice 8":string}[])
                    }
                  }
                }
                n519 = for {
                  shift-right: [w1095] -> w1090
                  shift-left: w1092 -> [w1097]
                  tunnel: w1091 -> [w1096] mode=indexing
                  n520 = Unbundle(w1096) -> (w1099:dbl)  [unwired: 1 out]
                  n521 = Not Equal To 0?(x=w1099) -> (x != 0?=w1098:bool)
                  n522 = case shown="True" w1098 {
                    tunnel: w1097 -> [w1100 w1103]
                    tunnel: w1096 -> [_ w1102]
                    tunnel: [w1100 w1101] -> w1095
                    frame False {
                    }
                    frame True {
                      n523 = Build Array (concatenate)(w1103, w1102) -> (w1101:cluster{dbl, "GUIdevice 8":string}[])
                    }
                  }
                }
              }
            }
            n524 = call <vilib>:"Add State(s) to Queue__jki_lib_state_machine.vi"("State(s) in (\"\")"=w1024) -> ("States Out"=w1023:string)  [unwired: 14 in]
            n525 = Bundle By Name(cluster=w1005, "speedmode X"=w1007, "speedmode Y"=w1006) -> (w1004:T37)
            n526 = Index Array(array=w1020) -> (element=w1025:cluster{dbl, "GUIdevice 8":string})  [unwired: 1 in]
            n527 = Index Array(array=w1021) -> (element=w1026:cluster{dbl, "GUIdevice 8":string})  [unwired: 1 in]
            n528 = Empty Array?(array=w1020) -> (empty?=w1028:bool)
            n529 = Unbundle(w1026) -> (w1034:dbl)  [unwired: 1 out]
            n530 = Unbundle(w1025) -> (w1030:dbl)  [unwired: 1 out]
            n531 = Unbundle By Name(w1004) -> ("Feedback global"=w1035:bool)
            n532 = Empty Array?(array=w1021) -> (empty?=w1032:bool)
            n533 = property on="autodetect" class="Bool (strict)"("Value"=FALSE ("autodetect")) -> ()  [unwired: 2 in, 2 out]
            n534 = Equal To 0?(x=w1034) -> (x = 0?=w1033:bool)
            n535 = Equal To 0?(x=w1030) -> (x = 0?=w1029:bool)
            n536 = Or(x=w1033, y=w1032) -> (x .or. y?=w1031:bool)
            n537 = Or(x=w1029, y=w1028) -> (x .or. y?=w1027:bool)
            n538 = case shown="True" w1035 {
              tunnel: w1031 -> [_ w1120]
              tunnel: w1021 -> [_ w1119]
              tunnel: w1027 -> [_ w1117]
              tunnel: w1020 -> [_ w1116]
              tunnel: w1023 -> [w1113 w1115]
              tunnel: [w1113 w1114] -> w1036
              frame False {
              }
              frame True {
                n539 = case shown="False" w1120 {
                  tunnel: w1119 -> [w1135 _]
                  tunnel: w1115 -> [w1131 w1136]
                  tunnel: [w1129 w1136] -> w1118
                  frame False {
                    n540 = Index Array(array=w1135) -> (element=w1134:cluster{dbl, "GUIdevice 8":string})  [unwired: 1 in]
                    n541 = Unbundle By Name(w1134) -> ("GUIdevice 8"=w1133:string)
                    n542 = call <vilib>:"Build State String with Arguments__jki_lib_state_machine.vi"("Arguments (\"\")"=w1133, "State"="Move X") -> ("State with Arguments"=w1130:string)  [unwired: 4 in]
                    n543 = call <vilib>:"Add State(s) to Queue__jki_lib_state_machine.vi"("State(s) in (\"\")"=w1131, "State(s) at Back (\"\")"=w1130) -> ("States Out"=w1129:string)  [unwired: 13 in]
                  }
                  frame True {
                  }
                }
                n544 = case shown="False" w1117 {
                  tunnel: w1116 -> [w1127 _]
                  tunnel: w1118 -> [w1123 w1128]
                  tunnel: [w1121 w1128] -> w1114
                  frame False {
                    n545 = Index Array(array=w1127) -> (element=w1126:cluster{dbl, "GUIdevice 8":string})  [unwired: 1 in]
                    n546 = Unbundle By Name(w1126) -> ("GUIdevice 8"=w1125:string)
                    n547 = call <vilib>:"Build State String with Arguments__jki_lib_state_machine.vi"("Arguments (\"\")"=w1125, "State"="Move Y") -> ("State with Arguments"=w1122:string)  [unwired: 4 in]
                    n548 = call <vilib>:"Add State(s) to Queue__jki_lib_state_machine.vi"("State(s) in (\"\")"=w1123, "State(s) at Back (\"\")"=w1122) -> ("States Out"=w1121:string)  [unwired: 13 in]
                  }
                  frame True {
                  }
                }
              }
            }
            n549 = call <vilib>:"Add State(s) to Queue__jki_lib_state_machine.vi"("State(s) in (\"\")"=w1023, "State(s) at Back (\"\")"=w1036) -> ("States Out"=w1038:string)  [unwired: 13 in]
          }
          frame "Move X" {
            # "Your code here.\n(You can make a copy of, or modify, this frame)"
            n550 = Unbundle By Name(w1156) -> ("Offset X"=w1155:dbl[][])
            n551 = call-poly <userlib>:"Filter 1D Array__ogtk.vi"("items to filter"=w1138, "array"=w1160) -> ("filtered item indices"=w1144:i32[])  [unwired: 4 in, 1 out]
            n552 = Unbundle By Name(w1156) -> ("active axis refs 2"=w1159:T12, "move properties"=w1143:T2[])
            n553 = for {
              tunnel: w1144 -> [w1165] mode=indexing
              tunnel: w1143 -> [w1169]
              shift-right: [w1164] -> w1141
              shift-left: i32[] [] ("filtered item indices") -> [w1167]
              n554 = Index Array(array=w1169, index=w1165) -> (element=w1168:T2)
              n555 = Unbundle By Name(w1168) -> ("enable feedback"=w1166:bool)
              n556 = case shown="True" w1166 {
                tunnel: w1167 -> [w1170 w1173]
                tunnel: w1165 -> [_ w1172]
                tunnel: [w1170 w1171] -> w1164
                frame False {
                }
                frame True {
                  n557 = Build Array (concatenate)(w1173, w1172) -> (w1171:i32[])
                }
              }
            }
            n558 = Index Array(array=w1141) -> (element=w1140:i32)  [unwired: 1 in]
            n559 = Index Array(array=w1155, index (row)=w1140) -> (element=w1154:dbl[])  [unwired: 1 in]
            n560 = Reverse 1D Array(array=w1154) -> (reversed array=w1153:dbl[])
            n561 = Index Array(array=w1159, index=w1140) -> (element=w1158:cluster{"Ref X":refnum<vi>, "Ref Y":refnum<vi>})
            n562 = Index Array(array=w1153) -> (element=w1151:dbl)  [unwired: 1 in]
            n563 = Index Array(array=w1143, index=w1140) -> (element=w1157:T2)
            n564 = Unbundle By Name(w1158) -> ("Ref X"=w1147:refnum<vi>, "Ref Y"=w1146:refnum<vi>)
            n565 = call <vilib>:"Build State String with Arguments__jki_lib_state_machine.vi"("Arguments (\"\")"=w1138, "State"="Wait" ("State(s) in Front (\"\")")) -> ("State with Arguments"=w1137:string)  [unwired: 4 in]
            n566 = Unbundle By Name(w1157) -> ("Invert Direction X"=w1148:bool, "Invert Axis"=w1152, "Stepsize"=w1149:dbl, "enable feedback"=w1145:bool)
            n567 = Greater Or Equal To 0?(x=w1151) -> (x >= 0?=w1150:bool)
            n568 = call <vilib>:"Add State(s) to Queue__jki_lib_state_machine.vi"("State(s) in Front (\"\")"=w1137, "State(s) in (\"\")"=w1163) -> ("States Out"=w1162:string)  [unwired: 13 in]
            n569 = case shown="True" w1145 {
              tunnel: w1152 -> [_ w1179]
              tunnel: w1150 -> [_ w1178]
              tunnel: w1149 -> [_ w1177]
              tunnel: w1148 -> [_ w1176]
              tunnel: w1147 -> [_ w1175]
              tunnel: w1146 -> [_ w1174]
              frame False {
              }
              frame True {
                n570 = case shown="False" w1178 {
                  tunnel: w1176 -> [w1187 w1209]
                  tunnel: w1177 -> [w1185 w1207]
                  tunnel: w1179 -> [w1184 w1206]
                  tunnel: w1179 -> [w1183 w1205]
                  tunnel: w1175 -> [w1181 w1203]
                  tunnel: w1174 -> [w1180 w1202]
                  frame True {
                    n571 = case shown="False" w1184 {
                      tunnel: [w1198 w1200] -> w1186
                      tunnel: w1181 -> [w1199 _]
                      tunnel: w1180 -> [_ w1201]
                      frame False {
                        n572 = property class="DigNum (strict)"(reference=w1199) -> ("Value"=w1198:dbl)  [unwired: 1 in, 2 out]
                      }
                      frame True {
                        n573 = property class="DigNum (strict)"(reference=w1201) -> ("Value"=w1200:dbl)  [unwired: 1 in, 2 out]
                      }
                    }
                    n574 = case shown="False" w1187 {
                      tunnel: w1186 -> [w1194 w1197]
                      tunnel: w1185 -> [w1193 w1196]
                      tunnel: [w1192 w1195] -> w1182
                      frame False {
                        n575 = Add(x=w1194, y=w1193) -> (x+y=w1192:dbl)
                      }
                      frame True {
                        n576 = Subtract(x=w1197, y=w1196) -> (x-y=w1195:dbl)
                      }
                    }
                    n577 = case shown="False" w1183 {
                      tunnel: w1182 -> [w1188 w1190]
                      tunnel: w1181 -> [w1189 _]
                      tunnel: w1180 -> [_ w1191]
                      frame False {
                        n578 = property class="DigNum (strict)"(reference=w1189, "Val(Sgnl)"=w1188) -> ()  [unwired: 1 in, 2 out]
                      }
                      frame True {
                        n579 = property class="DigNum (strict)"(reference=w1191, "Val(Sgnl)"=w1190) -> ()  [unwired: 1 in, 2 out]
                      }
                    }
                  }
                  frame False {
                    n580 = case shown="False" w1206 {
                      tunnel: [w1220 w1222] -> w1208
                      tunnel: w1203 -> [w1221 _]
                      tunnel: w1202 -> [_ w1223]
                      frame False {
                        n581 = property class="DigNum (strict)"(reference=w1221) -> ("Value"=w1220:dbl)  [unwired: 1 in, 2 out]
                      }
                      frame True {
                        n582 = property class="DigNum (strict)"(reference=w1223) -> ("Value"=w1222:dbl)  [unwired: 1 in, 2 out]
                      }
                    }
                    n583 = case shown="False" w1209 {
                      tunnel: w1208 -> [w1216 w1219]
                      tunnel: w1207 -> [w1215 w1218]
                      tunnel: [w1214 w1217] -> w1204
                      frame False {
                        n584 = Subtract(x=w1216, y=w1215) -> (x-y=w1214:dbl)
                      }
                      frame True {
                        n585 = Add(x=w1219, y=w1218) -> (x+y=w1217:dbl)
                      }
                    }
                    n586 = case shown="False" w1205 {
                      tunnel: w1204 -> [w1210 w1212]
                      tunnel: w1203 -> [w1211 _]
                      tunnel: w1202 -> [_ w1213]
                      frame False {
                        n587 = property class="DigNum (strict)"(reference=w1211, "Val(Sgnl)"=w1210) -> ()  [unwired: 1 in, 2 out]
                      }
                      frame True {
                        n588 = property class="DigNum (strict)"(reference=w1213, "Val(Sgnl)"=w1212) -> ()  [unwired: 1 in, 2 out]
                      }
                    }
                  }
                }
              }
            }
            "Moving X" <- w1138
          }
          frame "ManMove X" {
            # "Your code here.\n(You can make a copy of, or modify, this frame)"
            n589 = Equal?(x=w1229, y="Right") -> (x = y?=w1230:bool)
            n590 = Unbundle By Name(w1239) -> ("move properties"=w1234:T2[], "active ccd"=w1227:i32, "active man refs"=w1232:cluster{"Ref X":refnum<vi>, "Ref Y":refnum<vi>}, "active cams"=w1228:string[])
            n591 = Index Array(array=w1228, index=w1227) -> (element=w1225:string)
            n592 = Index Array(array=w1234, index=w1227) -> (element=w1240:T2)
            n593 = Unbundle By Name(w1232) -> ("Ref X"=w1236:refnum<vi>, "Ref Y"=w1235:refnum<vi>)
            n594 = Unbundle By Name(w1240) -> ("Invert Direction X"=w1237:bool, "Invert Axis"=w1238)
            n595 = call <vilib>:"Build State String with Arguments__jki_lib_state_machine.vi"("Arguments (\"\")"=w1225, "State"="Wait" ("State(s) in Front (\"\")")) -> ("State with Arguments"=w1224:string)  [unwired: 4 in]
            n596 = call <vilib>:"Add State(s) to Queue__jki_lib_state_machine.vi"("State(s) in Front (\"\")"=w1224, "State(s) in (\"\")"=w1243) -> ("States Out"=w1242:string)  [unwired: 13 in]
            n597 = case shown="False" w1230 {
              tunnel: w1237 -> [w1251 w1273]
              tunnel: "StepSize" -> [w1249 w1271]
              tunnel: w1238 -> [w1248 w1270]
              tunnel: w1238 -> [w1247 w1269]
              tunnel: w1236 -> [w1245 w1267]
              tunnel: w1235 -> [w1244 w1266]
              frame True {
                n598 = case shown="False" w1248 {
                  tunnel: [w1262 w1264] -> w1250
                  tunnel: w1245 -> [w1263 _]
                  tunnel: w1244 -> [_ w1265]
                  frame False {
                    n599 = property class="DigNum (strict)"(reference=w1263) -> ("Value"=w1262:dbl)  [unwired: 1 in, 2 out]
                  }
                  frame True {
                    n600 = property class="DigNum (strict)"(reference=w1265) -> ("Value"=w1264:dbl)  [unwired: 1 in, 2 out]
                  }
                }
                n601 = case shown="False" w1251 {
                  tunnel: w1250 -> [w1258 w1261]
                  tunnel: w1249 -> [w1257 w1260]
                  tunnel: [w1256 w1259] -> w1246
                  frame False {
                    n602 = Add(x=w1258, y=w1257) -> (x+y=w1256:dbl)
                  }
                  frame True {
                    n603 = Subtract(x=w1261, y=w1260) -> (x-y=w1259:dbl)
                  }
                }
                n604 = case shown="False" w1247 {
                  tunnel: w1246 -> [w1252 w1254]
                  tunnel: w1245 -> [w1253 _]
                  tunnel: w1244 -> [_ w1255]
                  frame False {
                    n605 = property class="DigNum (strict)"(reference=w1253, "Val(Sgnl)"=w1252) -> ()  [unwired: 1 in, 2 out]
                  }
                  frame True {
                    n606 = property class="DigNum (strict)"(reference=w1255, "Val(Sgnl)"=w1254) -> ()  [unwired: 1 in, 2 out]
                  }
                }
              }
              frame False {
                n607 = case shown="True" w1270 {
                  tunnel: [w1284 w1286] -> w1272
                  tunnel: w1267 -> [w1285 _]
                  tunnel: w1266 -> [_ w1287]
                  frame False {
                    n608 = property class="DigNum (strict)"(reference=w1285) -> ("Value"=w1284:dbl)  [unwired: 1 in, 2 out]
                  }
                  frame True {
                    n609 = property class="DigNum (strict)"(reference=w1287) -> ("Value"=w1286:dbl)  [unwired: 1 in, 2 out]
                  }
                }
                n610 = case shown="False" w1273 {
                  tunnel: w1272 -> [w1280 w1283]
                  tunnel: w1271 -> [w1279 w1282]
                  tunnel: [w1278 w1281] -> w1268
                  frame False {
                    n611 = Subtract(x=w1280, y=w1279) -> (x-y=w1278:dbl)
                  }
                  frame True {
                    n612 = Add(x=w1283, y=w1282) -> (x+y=w1281:dbl)
                  }
                }
                n613 = case shown="False" w1269 {
                  tunnel: w1268 -> [w1274 w1276]
                  tunnel: w1267 -> [w1275 _]
                  tunnel: w1266 -> [_ w1277]
                  frame False {
                    n614 = property class="DigNum (strict)"(reference=w1275, "Val(Sgnl)"=w1274) -> ()  [unwired: 1 in, 2 out]
                  }
                  frame True {
                    n615 = property class="DigNum (strict)"(reference=w1277, "Val(Sgnl)"=w1276) -> ()  [unwired: 1 in, 2 out]
                  }
                }
              }
            }
          }
          frame "ManMove Y" {
            # "Your code here.\n(You can make a copy of, or modify, this frame)"
            n616 = Equal?(x=w1293, y="Down") -> (x = y?=w1297:bool)
            n617 = Unbundle By Name(w1303) -> ("active cams"=w1292:string[], "move properties"=w1302:T2[], "active ccd"=w1291:i32, "active man refs"=w1301:cluster{"Ref X":refnum<vi>, "Ref Y":refnum<vi>})
            n618 = Index Array(array=w1292, index=w1291) -> (element=w1289:string)
            n619 = property on="StepSize" class="DigNum (strict)"() -> ("Value"=w1294:dbl)  [unwired: 2 in, 2 out]
            n620 = Index Array(array=w1302, index=w1291) -> (element=w1304:T2)
            n621 = Unbundle By Name(w1301) -> ("Ref Y"=w1296:refnum<vi>, "Ref X"=w1295:refnum<vi>)
            n622 = Unbundle By Name(w1304) -> ("Invert Direction Y"=w1299:bool, "Invert Axis"=w1298)
            n623 = call <vilib>:"Build State String with Arguments__jki_lib_state_machine.vi"("Arguments (\"\")"=w1289, "State"="Wait" ("State(s) in Front (\"\")")) -> ("State with Arguments"=w1288:string)  [unwired: 4 in]
            n624 = call <vilib>:"Add State(s) to Queue__jki_lib_state_machine.vi"("State(s) in Front (\"\")"=w1288, "State(s) in (\"\")"=w1307) -> ("States Out"=w1306:string)  [unwired: 13 in]
            n625 = case shown="True" w1297 {
              tunnel: w1299 -> [w1315 w1337]
              tunnel: w1294 -> [w1313 w1335]
              tunnel: w1298 -> [w1312 w1334]
              tunnel: w1298 -> [w1311 w1333]
              tunnel: w1296 -> [w1309 w1331]
              tunnel: w1295 -> [w1308 w1330]
              frame True {
                n626 = case shown="False" w1312 {
                  tunnel: [w1326 w1328] -> w1314
                  tunnel: w1309 -> [w1327 _]
                  tunnel: w1308 -> [_ w1329]
                  frame False {
                    n627 = property class="DigNum (strict)"(reference=w1327) -> ("Value"=w1326:dbl)  [unwired: 1 in, 2 out]
                  }
                  frame True {
                    n628 = property class="DigNum (strict)"(reference=w1329) -> ("Value"=w1328:dbl)  [unwired: 1 in, 2 out]
                  }
                }
                n629 = case shown="False" w1315 {
                  tunnel: w1314 -> [w1322 w1325]
                  tunnel: w1313 -> [w1321 w1324]
                  tunnel: [w1320 w1323] -> w1310
                  frame False {
                    n630 = Add(x=w1322, y=w1321) -> (x+y=w1320:dbl)
                  }
                  frame True {
                    n631 = Subtract(x=w1325, y=w1324) -> (x-y=w1323:dbl)
                  }
                }
                n632 = case shown="False" w1311 {
                  tunnel: w1310 -> [w1316 w1318]
                  tunnel: w1309 -> [w1317 _]
                  tunnel: w1308 -> [_ w1319]
                  frame False {
                    n633 = property class="DigNum (strict)"(reference=w1317, "Val(Sgnl)"=w1316) -> ()  [unwired: 1 in, 2 out]
                  }
                  frame True {
                    n634 = property class="DigNum (strict)"(reference=w1319, "Val(Sgnl)"=w1318) -> ()  [unwired: 1 in, 2 out]
                  }
                }
              }
              frame False {
                n635 = case shown="False" w1334 {
                  tunnel: [w1348 w1350] -> w1336
                  tunnel: w1331 -> [w1349 _]
                  tunnel: w1330 -> [_ w1351]
                  frame False {
                    n636 = property class="DigNum (strict)"(reference=w1349) -> ("Value"=w1348:dbl)  [unwired: 1 in, 2 out]
                  }
                  frame True {
                    n637 = property class="DigNum (strict)"(reference=w1351) -> ("Value"=w1350:dbl)  [unwired: 1 in, 2 out]
                  }
                }
                n638 = case shown="False" w1337 {
                  tunnel: w1336 -> [w1344 w1347]
                  tunnel: w1335 -> [w1343 w1346]
                  tunnel: [w1342 w1345] -> w1332
                  frame False {
                    n639 = Subtract(x=w1344, y=w1343) -> (x-y=w1342:dbl)
                  }
                  frame True {
                    n640 = Add(x=w1347, y=w1346) -> (x+y=w1345:dbl)
                  }
                }
                n641 = case shown="False" w1333 {
                  tunnel: w1332 -> [w1338 w1340]
                  tunnel: w1331 -> [w1339 _]
                  tunnel: w1330 -> [_ w1341]
                  frame False {
                    n642 = property class="DigNum (strict)"(reference=w1339, "Val(Sgnl)"=w1338) -> ()  [unwired: 1 in, 2 out]
                  }
                  frame True {
                    n643 = property class="DigNum (strict)"(reference=w1341, "Val(Sgnl)"=w1340) -> ()  [unwired: 1 in, 2 out]
                  }
                }
              }
            }
          }
          frame "Move Y" {
            # "Your code here.\n(You can make a copy of, or modify, this frame)"
            n644 = Unbundle By Name(w1371) -> ("Offset Y"=w1370:dbl[][])
            n645 = call-poly <userlib>:"Filter 1D Array__ogtk.vi"("items to filter"=w1353, "array"=w1375) -> ("filtered item indices"=w1359:i32[])  [unwired: 4 in, 1 out]
            n646 = Unbundle By Name(w1371) -> ("active axis refs 2"=w1374:T12, "move properties"=w1357:T2[])
            n647 = for {
              tunnel: w1359 -> [w1380] mode=indexing
              tunnel: w1357 -> [w1384]
              shift-right: [w1379] -> w1358
              shift-left: i32[] [] ("filtered item indices") -> [w1382]
              n648 = Index Array(array=w1384, index=w1380) -> (element=w1383:T2)
              n649 = Unbundle By Name(w1383) -> ("enable feedback"=w1381:bool)
              n650 = case shown="True" w1381 {
                tunnel: w1382 -> [w1385 w1388]
                tunnel: w1380 -> [_ w1387]
                tunnel: [w1385 w1386] -> w1379
                frame False {
                }
                frame True {
                  n651 = Build Array (concatenate)(w1388, w1387) -> (w1386:i32[])
                }
              }
            }
            n652 = Index Array(array=w1358) -> (element=w1355:i32)  [unwired: 1 in]
            n653 = Index Array(array=w1370, index (row)=w1355) -> (element=w1369:dbl[])  [unwired: 1 in]
            n654 = Reverse 1D Array(array=w1369) -> (reversed array=w1368:dbl[])
            n655 = Index Array(array=w1374, index=w1355) -> (element=w1373:cluster{"Ref X":refnum<vi>, "Ref Y":refnum<vi>})
            n656 = Index Array(array=w1368) -> (element=w1366:dbl)  [unwired: 1 in]
            n657 = Index Array(array=w1357, index=w1355) -> (element=w1372:T2)
            n658 = Unbundle By Name(w1373) -> ("Ref Y"=w1362:refnum<vi>, "Ref X"=w1361:refnum<vi>)
            n659 = Unbundle By Name(w1372) -> ("Invert Direction Y"=w1363:bool, "Invert Axis"=w1367, "Stepsize"=w1364:dbl, "enable feedback"=w1360:bool)
            n660 = Greater Or Equal To 0?(x=w1366) -> (x >= 0?=w1365:bool)
            n661 = call <vilib>:"Build State String with Arguments__jki_lib_state_machine.vi"("Arguments (\"\")"=w1353, "State"="Wait" ("State(s) in Front (\"\")")) -> ("State with Arguments"=w1352:string)  [unwired: 4 in]
            n662 = call <vilib>:"Add State(s) to Queue__jki_lib_state_machine.vi"("State(s) in Front (\"\")"=w1352, "State(s) in (\"\")"=w1378) -> ("States Out"=w1377:string)  [unwired: 13 in]
            n663 = case shown="True" w1360 {
              tunnel: w1367 -> [_ w1394]
              tunnel: w1365 -> [_ w1393]
              tunnel: w1364 -> [_ w1392]
              tunnel: w1363 -> [_ w1391]
              tunnel: w1362 -> [_ w1390]
              tunnel: w1361 -> [_ w1389]
              frame False {
              }
              frame True {
                n664 = case shown="True" w1393 {
                  tunnel: w1391 -> [w1402 w1424]
                  tunnel: w1392 -> [w1400 w1422]
                  tunnel: w1394 -> [w1399 w1421]
                  tunnel: w1394 -> [w1398 w1420]
                  tunnel: w1390 -> [w1396 w1418]
                  tunnel: w1389 -> [w1395 w1417]
                  frame True {
                    n665 = case shown="False" w1399 {
                      tunnel: [w1413 w1415] -> w1401
                      tunnel: w1396 -> [w1414 _]
                      tunnel: w1395 -> [_ w1416]
                      frame False {
                        n666 = property class="DigNum (strict)"(reference=w1414) -> ("Value"=w1413:dbl)  [unwired: 1 in, 2 out]
                      }
                      frame True {
                        n667 = property class="DigNum (strict)"(reference=w1416) -> ("Value"=w1415:dbl)  [unwired: 1 in, 2 out]
                      }
                    }
                    n668 = case shown="False" w1402 {
                      tunnel: w1401 -> [w1409 w1412]
                      tunnel: w1400 -> [w1408 w1411]
                      tunnel: [w1407 w1410] -> w1397
                      frame False {
                        n669 = Add(x=w1409, y=w1408) -> (x+y=w1407:dbl)
                      }
                      frame True {
                        n670 = Subtract(x=w1412, y=w1411) -> (x-y=w1410:dbl)
                      }
                    }
                    n671 = case shown="False" w1398 {
                      tunnel: w1397 -> [w1403 w1405]
                      tunnel: w1396 -> [w1404 _]
                      tunnel: w1395 -> [_ w1406]
                      frame False {
                        n672 = property class="DigNum (strict)"(reference=w1404, "Val(Sgnl)"=w1403) -> ()  [unwired: 1 in, 2 out]
                      }
                      frame True {
                        n673 = property class="DigNum (strict)"(reference=w1406, "Val(Sgnl)"=w1405) -> ()  [unwired: 1 in, 2 out]
                      }
                    }
                  }
                  frame False {
                    n674 = case shown="False" w1421 {
                      tunnel: [w1435 w1437] -> w1423
                      tunnel: w1418 -> [w1436 _]
                      tunnel: w1417 -> [_ w1438]
                      frame False {
                        n675 = property class="DigNum (strict)"(reference=w1436) -> ("Value"=w1435:dbl)  [unwired: 1 in, 2 out]
                      }
                      frame True {
                        n676 = property class="DigNum (strict)"(reference=w1438) -> ("Value"=w1437:dbl)  [unwired: 1 in, 2 out]
                      }
                    }
                    n677 = case shown="False" w1424 {
                      tunnel: w1423 -> [w1431 w1434]
                      tunnel: w1422 -> [w1430 w1433]
                      tunnel: [w1429 w1432] -> w1419
                      frame False {
                        n678 = Subtract(x=w1431, y=w1430) -> (x-y=w1429:dbl)
                      }
                      frame True {
                        n679 = Add(x=w1434, y=w1433) -> (x+y=w1432:dbl)
                      }
                    }
                    n680 = case shown="False" w1420 {
                      tunnel: w1419 -> [w1425 w1427]
                      tunnel: w1418 -> [w1426 _]
                      tunnel: w1417 -> [_ w1428]
                      frame False {
                        n681 = property class="DigNum (strict)"(reference=w1426, "Val(Sgnl)"=w1425) -> ()  [unwired: 1 in, 2 out]
                      }
                      frame True {
                        n682 = property class="DigNum (strict)"(reference=w1428, "Val(Sgnl)"=w1427) -> ()  [unwired: 1 in, 2 out]
                      }
                    }
                  }
                }
              }
            }
            "Moving Y" <- w1353
          }
          frame "Wait" {
            # "Your code here.\n(You can make a copy of, or modify, this frame)"
            n683 = flat-sequence {
              tunnel: T20."Disabled and Grayed Out" ("Disabled") -> [w1455]
              tunnel: w1445 -> [w1464]
              tunnel: w1444 -> [w1463]
              tunnel: [w1462] -> w1443
              tunnel: w1442 -> [w1461]
              tunnel: w1441 -> [w1460]
              tunnel: T20."Enabled" ("Disabled") -> [w1474]
              frame #0 {
                n684 = property on="Right" class="Bool (strict)"("DisabledEnum"=w1455) -> ()  [unwired: 2 in, 2 out]
                n685 = property on="Up" class="Bool (strict)"("DisabledEnum"=w1455) -> ()  [unwired: 2 in, 2 out]
                n686 = property on="Left" class="Bool (strict)"("DisabledEnum"=w1455) -> ()  [unwired: 2 in, 2 out]
                n687 = property on="Down" class="Bool (strict)"("DisabledEnum"=w1455) -> ()  [unwired: 2 in, 2 out]
                n688 = property on="StepSize" class="DigNum (strict)"("DisabledEnum"=w1455) -> ()  [unwired: 2 in, 2 out]
              }
              frame #1 {
                n689 = Wait (ms)(milliseconds to wait=u32 800) -> ()  [unwired: 1 out]
              }
              frame #2 {
                n690 = property on="Moving Y" class="Str"("Value"="") -> ()  [unwired: 2 in, 2 out]
                n691 = property on="Moving X" class="Str"("Value"="") -> ()  [unwired: 2 in, 2 out]
              }
              frame #3 {
                n692 = Equal?(x=w1460, y=w1461) -> (x = y?=w1459:bool)
                n693 = case shown="True" w1459 {
                  tunnel: w1464 -> [_ w1471]
                  tunnel: w1463 -> [w1465 w1468]
                  tunnel: [w1465 w1466] -> w1462
                  frame False {
                  }
                  frame True {
                    n694 = Unbundle By Name(w1471) -> ("Ref X"=w1470:refnum<vi>, "Ref Y"=w1469:refnum<vi>)
                    n695 = property class="DigNum (strict)"(reference=w1470, error in=w1468) -> (error out=w1467:errorcluster, "Value"=w1473:dbl)  [unwired: 1 out]
                    n696 = property class="DigNum (strict)"(reference=w1469, error in=w1467) -> (error out=w1466:errorcluster, "Value"=w1472:dbl)  [unwired: 1 out]
                    n697 = property on="Position 1" class="DigNum (strict)"("Value"=w1473) -> ()  [unwired: 2 in, 2 out]
                    n698 = property on="Position 2" class="DigNum (strict)"("Value"=w1472) -> ()  [unwired: 2 in, 2 out]
                  }
                }
              }
              frame #4 {
                n699 = property on="Right" class="Bool (strict)"("DisabledEnum"=w1474) -> ()  [unwired: 2 in, 2 out]
                n700 = property on="Up" class="Bool (strict)"("DisabledEnum"=w1474) -> ()  [unwired: 2 in, 2 out]
                n701 = property on="Left" class="Bool (strict)"("DisabledEnum"=w1474) -> ()  [unwired: 2 in, 2 out]
                n702 = property on="Down" class="Bool (strict)"("DisabledEnum"=w1474) -> ()  [unwired: 2 in, 2 out]
                n703 = property on="StepSize" class="DigNum (strict)"("DisabledEnum"=w1474) -> ()  [unwired: 2 in, 2 out]
              }
            }
            n704 = call-poly <userlib>:"Filter 1D Array__ogtk.vi"("items to filter"=w1448, "array"=w1449) -> ("filtered item indices"=w1447:i32[])  [unwired: 4 in, 1 out]
            n705 = Index Array(array=w1447) -> (element=w1442:i32)  [unwired: 1 in]
            n706 = Unbundle By Name(w1450) -> ("active axis refs 2"=w1446:T12, "active ccd"=w1441:i32)
            n707 = Index Array(array=w1446, index=w1442) -> (element=w1445:cluster{"Ref X":refnum<vi>, "Ref Y":refnum<vi>})
            n708 = call <vilib>:"Add State(s) to Queue__jki_lib_state_machine.vi"("State(s) in (\"\")"=w1454) -> ("States Out"=w1453:string)  [unwired: 14 in]
            n709 = local read "Mean Centroid X"() -> (w1451:dbl[][])
            n710 = Bundle By Name(cluster=w1450, "Mean Centroid X"=w1451, "Mean Centroid Y"=w1451) -> (w1452:T37)
          }
          frame "---------------Statistics--------------" {
            # "Template Separator\n(You can make a copy of, or modify, this frame)"
            n711 = call <vilib>:"Add State(s) to Queue__jki_lib_state_machine.vi"("State(s) in (\"\")"=w1478) -> ("States Out"=w1477:string)  [unwired: 14 in]
          }
          frame "Save Stats" {
            # "Your code here.\n(You can make a copy of, or modify, this frame)"
            n712 = property on="CCD 1" class="XYGraph (strict)"() -> ("Value"=w1488:cluster{timestamp[], dbl[]}[])  [unwired: 2 in, 2 out]
            n713 = property on="CCD 2" class="XYGraph (strict)"() -> ("Value"=w1487:cluster{timestamp[], dbl[]}[])  [unwired: 2 in, 2 out]
            n714 = property on="CCD 3" class="XYGraph (strict)"() -> ("Value"=w1486:cluster{timestamp[], dbl[]}[])  [unwired: 2 in, 2 out]
            n715 = property on="CCD 4" class="XYGraph (strict)"() -> ("Value"=w1485:cluster{timestamp[], dbl[]}[])  [unwired: 2 in, 2 out]
            n716 = property on="CCD 5" class="XYGraph (strict)"() -> ("Value"=w1484:cluster{timestamp[], dbl[]}[])  [unwired: 2 in, 2 out]
            n717 = property on="CCD 6" class="XYGraph (strict)"() -> ("Value"=w1483:cluster{timestamp[], dbl[]}[])  [unwired: 2 in, 2 out]
            n718 = property on="CCD 7" class="XYGraph (strict)"() -> ("Value"=w1482:cluster{timestamp[], dbl[]}[])  [unwired: 2 in, 2 out]
            n719 = property on="CCD 8" class="XYGraph (strict)"() -> ("Value"=w1481:cluster{timestamp[], dbl[]}[])  [unwired: 2 in, 2 out]
            n720 = Build Array(w1488, w1487, w1486, w1485, w1484, w1483, w1482, w1481) -> (w1480:cluster{timestamp[], dbl[]}[][])
            n721 = for {
              tunnel: w1480 -> [w1496] mode=indexing
              tunnel: w1479 -> [w1495] mode=indexing
              n722 = Empty String/Path?(string/path=w1495) -> (empty?=w1494:bool)
              n723 = case shown="False" w1494 {
                tunnel: w1496 -> [w1502 _]
                tunnel: w1495 -> [w1500 _]
                frame False {
                  n724 = Index Array(array=w1502, index #1=0 ("index"), index #2=1 ("index"), index #3=2 ("index"), index #4=3 ("index")) -> (element #1=w1537:cluster{timestamp[], dbl[]}, element #2=w1531:cluster{timestamp[], dbl[]}, element #3=w1530:cluster{timestamp[], dbl[]}, element #4=w1529:cluster{timestamp[], dbl[]})  [unwired: 1 in, 1 out]
                  n725 = Concatenate Strings(w1500, ".dat" ("string")) -> (w1498:string)
                  n726 = Unbundle(w1537) -> (w1536:timestamp[], w1514:dbl[])
                  n727 = Unbundle(w1531) -> (w1505:dbl[])  [unwired: 1 out]
                  n728 = Unbundle(w1530) -> (w1504:dbl[])  [unwired: 1 out]
                  n729 = Unbundle(w1529) -> (w1503:dbl[])  [unwired: 1 out]
                  n730 = Build Path(base path="save path", name or relative path=w1498) -> (appended path=w1497:path)
                  n731 = for {
                    tunnel: w1536 -> [w1539] mode=indexing
                    tunnel: [w1538] -> w1512 mode=indexing
                    n732 = Format Date/Time String(time format string (%c)="%Y%m%d%H%M%S", seconds (now)=w1539) -> (date/time string=w1538:string)  [unwired: 1 in]
                  }
                  n733 = Array Size(array=w1514) -> (size(s)=w1515:i32)
                  n734 = Number To Fractional String(number=w1514) -> (F-format string=w1511:string[])  [unwired: 3 in]
                  n735 = Number To Fractional String(number=w1505) -> (F-format string=w1508:string[])  [unwired: 3 in]
                  n736 = Number To Fractional String(number=w1504) -> (F-format string=w1507:string[])  [unwired: 3 in]
                  n737 = Number To Fractional String(number=w1503) -> (F-format string=w1506:string[])  [unwired: 3 in]
                  n738 = Initialize Array("", w1515, 5 ("dimension size")) -> (w1513:string[][])
                  n739 = Insert Into Array(array=w1513, index (col)=0 ("disabled index (col)"), new element=w1512) -> (w1523:string[][])  [unwired: 1 in]
                  n740 = Insert Into Array(array=w1523, index (col)=1 ("disabled index (col)"), new element=w1511) -> (w1522:string[][])  [unwired: 1 in]
                  n741 = Insert Into Array(array=w1522, index (col)=2 ("disabled index (col)"), new element=w1508) -> (w1526:string[][])  [unwired: 1 in]
                  n742 = Insert Into Array(array=w1526, index (col)=3 ("disabled index (col)"), new element=w1507) -> (w1527:string[][])  [unwired: 1 in]
                  n743 = Insert Into Array(array=w1527, index (col)=4 ("disabled index (col)"), new element=w1506) -> (w1528:string[][])  [unwired: 1 in]
                  n744 = Insert Into Array(array=w1528, index (row)=0, new element=string[] ["time", "Centroid X", "Centroid Y", "Motor Axis 1", "Motor Axis 2"] ("new element/subarray 2")) -> (w1510:string[][])  [unwired: 1 in]
                  n745 = call-poly <vilib>:"Write To Spreadsheet File.vi"("2D data"=w1510, "file path (dialog if empty)"=w1497) -> ()  [unwired: 6 in, 1 out]
                }
                frame True {
                }
              }
            }
            n746 = call <vilib>:"Add State(s) to Queue__jki_lib_state_machine.vi"("State(s) in (\"\")"=w1493) -> ("States Out"=w1492:string)  [unwired: 14 in]
            n747 = property on="Save Stats" class="Bool (strict)"("Value"=FALSE ("Save Stats")) -> ()  [unwired: 2 in, 2 out]
          }
          frame "tdms" {
            w1564 = 21600.0 ("new tdms")
            # "Your code here.\n(You can make a copy of, or modify, this frame)"
            n748 = Unbundle By Name(w1556) -> ("active cams"=w1557:string[], "Data Value Reference out"=w1574:refnum<k34>, "Offset X"=w1573:dbl[][], "Offset Y"=w1572:dbl[][], "active axis refs 2"=w1571:T12)
            n749 = for {
              tunnel: w1573 -> [w1619]
              tunnel: w1572 -> [w1618]
              tunnel: w1557 -> [w1582] mode=indexing
              tunnel: w1574 -> [w1583]
              tunnel: w1571 -> [w1604]
              tunnel: w1570 -> [w1588]
              tunnel: [w1586] -> w1569
              i -> [w1605]
              n750 = Index Array(array=w1619, index (row)=w1605) -> (element=w1617:dbl[])  [unwired: 1 in]
              n751 = Index Array(array=w1618, index (row)=w1605) -> (element=w1616:dbl[])  [unwired: 1 in]
              n752 = Index Array(array=w1604, index=w1605) -> (element=w1603:cluster{"Ref X":refnum<vi>, "Ref Y":refnum<vi>})
              n753 = Reverse 1D Array(array=w1616) -> (reversed array=w1614:dbl[])
              n754 = Reverse 1D Array(array=w1617) -> (reversed array=w1615:dbl[])
              n755 = Unbundle By Name(w1603) -> ("Ref X"=w1602:refnum<vi>, "Ref Y"=w1601:refnum<vi>)
              n756 = Index Array(array=w1615) -> (element=w1613:dbl)  [unwired: 1 in]
              n757 = Index Array(array=w1614) -> (element=w1612:dbl)  [unwired: 1 in]
              n758 = property class="DigNum (strict)"(reference=w1602, error in=w1588) -> (error out=w1587:errorcluster, "Value"=w1596:dbl)  [unwired: 1 out]
              n759 = Build Array(w1613) -> (w1585:dbl[])
              n760 = Build Array(w1612) -> (w1607:dbl[])
              n761 = Get Date/Time In Seconds() -> (seconds since 1Jan1904=w1584:timestamp)
              n762 = Build Array(w1584) -> (w1580:timestamp[])
              n763 = property class="DigNum (strict)"(reference=w1601, error in=w1587) -> (error out=w1578:errorcluster, "Value"=w1590:dbl)  [unwired: 1 out]
              n764 = Build Array(w1596) -> (w1595:dbl[])
              n765 = TDMS Write(0:w1583, 5:w1582, 7:"time", 9:w1580, 11:w1578) -> (4:w1579:refnum<k34>, 15:w1577:errorcluster)  [unwired: 1 in, 2 out]
              n766 = Build Array(w1590) -> (w1589:dbl[])
              n767 = TDMS Write(0:w1579, 5:w1582, 7:"centroid X", 9:w1585, 11:w1577) -> (4:w1610:refnum<k34>, 6:w1609:string, 15:w1608:errorcluster)  [unwired: 1 in, 1 out]
              n768 = TDMS Write(0:w1610, 5:w1609, 7:"centroid Y", 9:w1607, 11:w1608) -> (4:w1599:refnum<k34>, 6:w1598:string, 15:w1600:errorcluster)  [unwired: 1 in, 1 out]
              n769 = TDMS Write(0:w1599, 5:w1598, 7:"Motor Axis 1", 9:w1595, 11:w1600) -> (4:w1594:refnum<k34>, 6:w1593:string, 15:w1591:errorcluster)  [unwired: 1 in, 1 out]
              n770 = TDMS Write(0:w1594, 5:w1593, 7:"Motor Axis 2", 9:w1589, 11:w1591) -> (15:w1586:errorcluster)  [unwired: 1 in, 3 out]
            }
            n771 = property on="millisecond timer value" class="DigNum (strict)"() -> ("Value"=w1543:u32)  [unwired: 2 in, 2 out]
            n772 = Tick Count (ms)() -> (millisecond timer value=w1542:u32)
            n773 = Subtract(x=w1542, y=w1543) -> (x-y=w1547:u32)
            n774 = Divide(x=w1547, y=u32 1000) -> (x/y=w1545:dbl)
            n775 = Unbundle By Name(w1556) -> ("img to avg"=w1544:i32)
            n776 = Multiply(x=5.0 ("new tdms"), y=w1544) -> (x*y=w1550:dbl)
            n777 = Quotient & Remainder(x=w1545, y=w1550) -> (x-y*floor(x/y)=w1549:dbl)  [unwired: 1 out]
            "x-y*floor(x/y)" <- w1549
            n778 = Subtract(x=w1550, y=2.0) -> (x-y=w1552:dbl)
            n779 = Greater?(x=w1549, y=w1552) -> (0:w1553:bool)
            n780 = Select(t="Device Ini", s=w1553, f="") -> (s? t:f=w1541:string)
            n781 = Subtract(x=w1542, y=w1543) -> (x-y=w1559:u32)
            n782 = Divide(x=w1559, y=u32 1000) -> (x/y=w1561:dbl)
            n783 = Quotient & Remainder(x=w1561, y=w1564) -> (x-y*floor(x/y)=w1562:dbl)  [unwired: 1 out]
            n784 = Subtract(x=w1564, y=20.0) -> (x-y=w1566:dbl)
            n785 = Greater?(x=w1562, y=w1566) -> (0:w1563:bool)
            n786 = Select(t="newtdms", s=w1563, f="") -> (s? t:f=w1558:string)
            n787 = call <vilib>:"Add State(s) to Queue__jki_lib_state_machine.vi"("State(s) in Front (\"\")"=w1541, "State(s) in (\"\")"=w1576, "State(s) at Back (\"\")"=w1558) -> ("States Out"=w1575:string)  [unwired: 12 in]
          }
          frame "Reset History" {
            # "Your code here.\n(You can make a copy of, or modify, this frame)"
            n788 = for {
              N: 1 -> [_]
              shift-right: [w1629] -> w1621
              shift-left: timestamp[][] [] ("Time") -> [w1631]
              n789 = for {
                N: 12 -> [_]
                tunnel: w1631 -> [w1634] mode=indexing
                tunnel: [w1632] -> w1629 mode=indexing
                n790 = Get Date/Time In Seconds() -> (seconds since 1Jan1904=w1633:timestamp)
                n791 = Build Array (concatenate)(w1634, w1633) -> (w1632:timestamp[])
              }
            }
            n792 = local read "Offset X"() -> (w1620:dbl[][])
            n793 = Bundle By Name(cluster=w1625, "Offset X"=w1620, "Offset Y"=w1620, "Time"=w1621, "Motor X"=w1620) -> (w1624:T37)
            n794 = call <vilib>:"Add State(s) to Queue__jki_lib_state_machine.vi"("State(s) in (\"\")"=w1628) -> ("States Out"=w1627:string)  [unwired: 14 in]
          }
          frame "New Category: 2" {
            # "Your code here.\n(You can make a copy of, or modify, this frame)"
            n795 = call <vilib>:"Add State(s) to Queue__jki_lib_state_machine.vi"("State(s) in (\"\")"=w1638) -> ("States Out"=w1637:string)  [unwired: 14 in]
          }
          frame "stats" {
            # "Your code here.\n(You can make a copy of, or modify, this frame)"
            n796 = Unbundle By Name(w1646) -> ("Offset X"=w1644:dbl[][], "Offset Y"=w1643:dbl[][], "Time"=w1642:timestamp[][], "Motor X"=w1641:dbl[][], "Motor Y"=w1640:dbl[][])
            n797 = for {
              tunnel: w1645 -> [_] mode=indexing
              tunnel: w1644 -> [w1683]
              tunnel: w1643 -> [w1682]
              tunnel: w1642 -> [w1681]
              tunnel: w1641 -> [w1677]
              tunnel: w1640 -> [w1676]
              tunnel: [w1685] -> w1639 mode=indexing
              i -> [w1684]
              n798 = Index Array(array=w1682, index (row)=w1684) -> (element=w1678:dbl[])  [unwired: 1 in]
              n799 = Index Array(array=w1677, index (row)=w1684) -> (element=w1675:dbl[])  [unwired: 1 in]
              n800 = Index Array(array=w1676, index (row)=w1684) -> (element=w1674:dbl[])  [unwired: 1 in]
              n801 = Index Array(array=w1683, index (row)=w1684) -> (element=w1679:dbl[])  [unwired: 1 in]
              n802 = Index Array(array=w1681, index (row)=w1684) -> (element=w1680:timestamp[])  [unwired: 1 in]
              n803 = Bundle("Time"=w1680, "Motor X"=w1675) -> (w1688:cluster{"Time":timestamp[], "Motor X":dbl[]})  [unwired: 1 in]
              n804 = Bundle("Time"=w1680, "Motor Y"=w1674) -> (w1689:cluster{"Time":timestamp[], "Motor Y":dbl[]})  [unwired: 1 in]
              n805 = Bundle("Time"=w1680, "Offset X"=w1679) -> (w1687:cluster{"Time":timestamp[], "Offset X":dbl[]})  [unwired: 1 in]
              n806 = Bundle("Time"=w1680, "Offset Y"=w1678) -> (w1686:cluster{"Time":timestamp[], "Offset Y":dbl[]})  [unwired: 1 in]
              n807 = Build Array(w1686, w1687, w1688, w1689) -> (w1685:cluster{"Time":timestamp[], "Motor Y":dbl[]}[])
            }
            n808 = call <vilib>:"Add State(s) to Queue__jki_lib_state_machine.vi"("State(s) in (\"\")"=w1673) -> ("States Out"=w1672:string)  [unwired: 14 in]
            n809 = Index Array(array=w1639, index (row) #1=0 ("index (row)"), index (row) #2=1 ("index (row)"), index (row) #3=2 ("index (row)"), index (row) #4=3 ("index (row)"), index (row) #5=4 ("index (row)"), index (row) #6=5 ("index (row)"), index (row) #7=6 ("index (row)"), index (row) #8=7 ("index (row)"), index (row) #9=8 ("index (row)"), index (row) #10=9 ("index (row)"), index (row) #11=10 ("index (row)"), index (row) #12=11 ("index (row)")) -> (element #1=→"CCD 1":cluster{"Time":timestamp[], "Motor Y":dbl[]}[], element #2=→"CCD 2":cluster{"Time":timestamp[], "Motor Y":dbl[]}[], element #3=→"CCD 3":cluster{"Time":timestamp[], "Motor Y":dbl[]}[], element #4=→"CCD 4":cluster{"Time":timestamp[], "Motor Y":dbl[]}[], element #5=→"CCD 5":cluster{"Time":timestamp[], "Motor Y":dbl[]}[], element #6=→"CCD 6":cluster{"Time":timestamp[], "Motor Y":dbl[]}[], element #7=→"CCD 7":cluster{"Time":timestamp[], "Motor Y":dbl[]}[], element #8=→"CCD 8":cluster{"Time":timestamp[], "Motor Y":dbl[]}[], element #9=→"CCD 9":cluster{"Time":timestamp[], "Motor Y":dbl[]}[], element #10=→"CCD 10":cluster{"Time":timestamp[], "Motor Y":dbl[]}[], element #11=→"CCD 11":cluster{"Time":timestamp[], "Motor Y":dbl[]}[], element #12=→"CCD 12":cluster{"Time":timestamp[], "Motor Y":dbl[]}[])  [unwired: 12 in]
          }
          frame "newtdms" {
            # "Your code here.\n(You can make a copy of, or modify, this frame)"
            n810 = Unbundle By Name(w1700) -> ("Data Value Reference out"=w1701:refnum<k34>, "active cams"=w1693:string[])
            n811 = TDMS Close(8:w1694, 11:w1701) -> (0:w1691:errorcluster)  [unwired: 1 out]
            n812 = call <vilib>:"Clear Errors.vi"("error in (no error)"=w1691) -> ("error out"=w1690:errorcluster)  [unwired: 5 in, 1 out]
            n813 = property on="new tdms" class="Bool (strict)"("Value"=FALSE ("new tdms")) -> ()  [unwired: 2 in, 2 out]
            n814 = Get Date/Time In Seconds() -> (seconds since 1Jan1904=w1711:timestamp)
            n815 = Format Date/Time String(time format string (%c)="%Y%m%d%H%M", seconds (now)=w1711) -> (date/time string=w1702:string)  [unwired: 1 in]
            n816 = Concatenate Strings(w1702, "Beampointing_TRA.tdms" ("string")) -> (w1708:string)
            n817 = String To Path(string=w1708) -> (path=w1709:path)
            n818 = Build Path(base path=path "W:/BP_DATA", name or relative path=w1709) -> (appended path=w1703:path)
            n819 = TDMS Open(6:FALSE ("disable buffering (T)"), 7:enum16{"1.0", "2.0"}."2.0" ("file format version (2.0)"), 8:w1690, 10:T17."create or replace" ("operation"), 11:w1703) -> (0:w1697:errorcluster, 3:w1696:refnum<k34>)  [unwired: 2 in]
            n820 = call <vilib>:"Add State(s) to Queue__jki_lib_state_machine.vi"("State(s) in (\"\")"=w1714) -> ("States Out"=w1713:string)  [unwired: 14 in]
            n821 = call "TDMSbuffersize.vi"("error in (no error)"=w1697, "group names"=w1693, "Data Value Reference in"=w1696) -> ("error out"=w1692:errorcluster, "Data Value Reference out"=w1695:refnum<k34>)  [unwired: 7 in]
            n822 = Bundle By Name(cluster=w1700, "Data Value Reference out"=w1695) -> (w1699:T37)
          }
          frame "Center" {
            # "Your code here.\n(You can make a copy of, or modify, this frame)"
            n823 = control-ref of="image::1"() -> (w1729:refnum<vi>)
            n824 = control-ref of="image::2"() -> (w1728:refnum<vi>)
            n825 = control-ref of="image::3"() -> (w1727:refnum<vi>)
            n826 = control-ref of="image::4"() -> (w1726:refnum<vi>)
            n827 = control-ref of="image::5"() -> (w1725:refnum<vi>)
            n828 = control-ref of="image::6"() -> (w1724:refnum<vi>)
            n829 = control-ref of="image::7"() -> (w1723:refnum<vi>)
            n830 = control-ref of="image::8"() -> (w1722:refnum<vi>)
            n831 = control-ref of="image::9"() -> (w1721:refnum<vi>)
            n832 = control-ref of="image::10"() -> (w1720:refnum<vi>)
            n833 = control-ref of="image::11"() -> (w1719:refnum<vi>)
            n834 = control-ref of="image::12"() -> (w1718:refnum<vi>)
            n835 = for {
              tunnel: [w1738] -> w1717 mode=indexing
              tunnel: w1716 -> [w1737] mode=indexing
              n836 = Unbundle By Name(w1737) -> ("Target.X::12"=w1736:refnum<vi>, "Target.Y::12"=w1735:refnum<vi>)
              n837 = property class="DigNum (strict)"(reference=w1736) -> ("Value"=w1739:dbl)  [unwired: 1 in, 2 out]
              n838 = property class="DigNum (strict)"(reference=w1735) -> ("Value"=w1740:dbl)  [unwired: 1 in, 2 out]
              n839 = Bundle("Value"=w1739, "Value"=w1740) -> (w1738:cluster{"Value":dbl, "Value":dbl})  [unwired: 1 in]
            }
            n840 = call <vilib>:"Add State(s) to Queue__jki_lib_state_machine.vi"("State(s) in (\"\")"=w1734) -> ("States Out"=w1733:string)  [unwired: 14 in]
            n841 = Build Array(w1729, w1728, w1727, w1726, w1725, w1724, w1723, w1722, w1721, w1720, w1719, w1718) -> (w1730:refnum<vi>[])
            n842 = for {
              tunnel: w1730 -> [w1742] mode=indexing
              tunnel: w1717 -> [w1741] mode=indexing
              n843 = property class="ImageControl"(reference=w1742, "Image Center Position"=w1741) -> ()  [unwired: 1 in, 2 out]
            }
            n844 = property on="Center" class="Bool (strict)"("Value"=FALSE ("Center")) -> ()  [unwired: 2 in, 2 out]
          }
          frame "ImgToAvg" {
            n845 = Decimal String To Number(string=w1749) -> (number=w1746:i32)  [unwired: 2 in, 1 out]
            n846 = Bundle By Name(cluster=w1748, "img to avg"=w1746) -> (w1747:T37)
            n847 = call <vilib>:"Add State(s) to Queue__jki_lib_state_machine.vi"("State(s) in (\"\")"=w1745) -> ("States Out"=w1744:string)  [unwired: 14 in]
          }
          frame "history" {
            # "Your code here.\n(You can make a copy of, or modify, this frame)"
            n848 = Unbundle By Name(w1759) -> ("Offset X"=w1765:dbl[][], "Offset Y"=w1764:dbl[][], "Mean Centroid X"=w1763:dbl[][], "Mean Centroid Y"=w1762:dbl[][], "Motor X"=w1761:dbl[][], "Motor Y"=w1760:dbl[][], "Time"=w1751:timestamp[][])
            n849 = for {
              tunnel: w1765 -> [w1783] mode=indexing
              tunnel: w1764 -> [w1781] mode=indexing
              tunnel: w1763 -> [w1780] mode=indexing
              tunnel: w1762 -> [w1779] mode=indexing
              tunnel: w1761 -> [w1778] mode=indexing
              tunnel: w1760 -> [w1777] mode=indexing
              tunnel: [w1782] -> w1757 mode=indexing
              tunnel: [w1776] -> w1756 mode=indexing
              tunnel: [w1772] -> w1755 mode=indexing
              tunnel: [w1775] -> w1754 mode=indexing
              tunnel: [w1774] -> w1753 mode=indexing
              tunnel: [w1773] -> w1752 mode=indexing
              tunnel: w1751 -> [w1771] mode=indexing
              tunnel: [w1769] -> w1750 mode=indexing
              w1770 = 0
              n850 = Delete From Array(array=w1778, index=w1770) -> (array with subset deleted=w1774:dbl[])  [unwired: 1 in, 1 out]
              n851 = Delete From Array(array=w1777, index=w1770) -> (array with subset deleted=w1773:dbl[])  [unwired: 1 in, 1 out]
              n852 = Delete From Array(array=w1771, index=w1770) -> (array with subset deleted=w1769:timestamp[])  [unwired: 1 in, 1 out]
              n853 = Delete From Array(array=w1780, index=w1770) -> (array with subset deleted=w1772:dbl[])  [unwired: 1 in, 1 out]
              n854 = Delete From Array(array=w1779, index=w1770) -> (array with subset deleted=w1775:dbl[])  [unwired: 1 in, 1 out]
              n855 = Delete From Array(array=w1781, index=w1770) -> (array with subset deleted=w1776:dbl[])  [unwired: 1 in, 1 out]
              n856 = Delete From Array(array=w1783, index=w1770) -> (array with subset deleted=w1782:dbl[])  [unwired: 1 in, 1 out]
            }
            n857 = call <vilib>:"Add State(s) to Queue__jki_lib_state_machine.vi"("State(s) in (\"\")"=w1768) -> ("States Out"=w1767:string)  [unwired: 14 in]
            n858 = Bundle By Name(cluster=w1759, "Offset X"=w1757, "Offset Y"=w1756, "Mean Centroid X"=w1755, "Mean Centroid Y"=w1754, "Motor X"=w1753, "Motor Y"=w1752, "Time"=w1750) -> (w1758:T37)
          }
        }
        n859 = property on="Box" class="Arr (strict)"() -> ("Value"=w135:T6)  [unwired: 2 in, 2 out]
        n860 = for {
          tunnel: w137 -> [w158]
          tunnel: w136 -> [w159]
          tunnel: w133 -> [w151] mode=indexing
          tunnel: w135 -> [w152] mode=indexing
          n861 = call-poly <userlib>:"Filter 1D Array__ogtk.vi"("items to filter"=w151, "array"=w159) -> ("filtered item indices"=w160:i32[])  [unwired: 4 in, 1 out]
          n862 = Index Array(array=w160) -> (element=w154:i32)  [unwired: 1 in]
          n863 = Index Array(array=w158, index=w154) -> (element=w157:T31)
          n864 = Unbundle By Name(w157) -> ("Target.X::12"=w162:refnum<vi>, "Target.Y::12"=w161:refnum<vi>)
          n865 = property class="DigNum (strict)"(reference=w162) -> ("Value"=w156:dbl)  [unwired: 1 in, 2 out]
          n866 = property class="DigNum (strict)"(reference=w161) -> ("Value"=w155:dbl)  [unwired: 1 in, 2 out]
          n867 = call "draw crosshair imaq.vi"(5:u32 16774656 ("Color"), 6:w155, "clear overlay"=cluster{"xhair size":dbl, "xhair size 2":dbl} {"xhair size"=25.0, "xhair size 2"=25.0} ("size"), "Crosshair"=w156, "Bounding Rectangle"=T15 {"Left"=0, "Top"=0, "Right"=0, "Bottom"=0}, "image in"=w151) -> ("image out"=w150:T9)  [unwired: 4 in, 1 out]
          n868 = call "draw box imaq.vi"("Color"=u32 1244928, "Rectangle"=w152, "image in"=w150) -> ()  [unwired: 7 in, 2 out]
        }
      }
      n869 = control-ref of="This Application"() -> (w123:refnum<vi>)
      n870 = control-ref of="This VI"() -> (w127:refnum<vi>)
      n871 = Current VI's Menubar() -> (w126:refnum<k9>)
      n872 = call "GUI_Master_subvi_reentrant_queues.vi"("This Application"=w123, "error in (no error)"=w124, "tcp data event"=w122, "Caller menu reference"=w126, "Caller VI ref"=w127) -> ("error out"=→"error IO 2":errorcluster)  [unwired: 6 in]
      n873 = Unbundle By Name(w66) -> ("Data Value Reference out"=w65:refnum<k34>)
      n874 = for {
        tunnel: w95 -> [w131] mode=indexing
        tunnel: w94 -> [w130]
        tunnel: [w129] -> w64
        n875 = call "IMAQ Dispose"("Image"=w131, "error in (no error)"=w130) -> ("error out"=w129:errorcluster)  [unwired: 4 in]
      }
      n876 = TDMS Close(8:w64, 11:w65) -> (0:→"error out 2":errorcluster)  [unwired: 1 out]
      "Names" <- w34
    }
  }
